vi "Auto_New.vi"() -> ()   [LabVIEW 2017]
uses:
  Control/Saurabh/prosucer_consumer_enum1.ctl
  <vilib>/Utility/error.llb/DialogType.ctl
  <vilib>/addons/database/Connection.llb/DB Tools Open Connec (String).vi
  Global/Global 1.vi
  Global/DATA LOG.vi
  <vilib>/addons/database/NI_Database_API.lvlib
panel:
  out "OP30 BARCODE STRING EMPRTY 2":bool
  out "SHIFT":string
  in  "BARCODE RECIPE":string(combo)
  out "PLC COM.":bool
  out "SHIFT_DATA":string[](array[string])
  out "OP30 BARCODE STRING EMPRTY":bool
  out "stop":bool
  out "error out 2":errorcluster
  out "Shift 4":i32
  out "Time Stamp Out":timestamp[](array[timestamp]) format="%<%X>T"
  out "Time Stamp Out 4":timestamp[](array[timestamp]) format="%<%X>T"
  out "Shift_change":bool
  out "appended array":string[][](array[string])
  out "SHIFT_DATA 2":string[](array[string])
  in  "error in (no error)":errorcluster
  in  "Tab Control":enum32{"Screen 1", "Screen 2"}(tab)
  out "OP 50":bool
  out "OP 40":bool
  out "OP 30":bool
  out "OP - 50":T1
  out "OP - 40":T2
  out "OP - 30":T3
  in  "stop 2":bool
  out "OP - 10":T4
  in  "SIMULATE INPUT":bool[](array[boolean])=[FALSE, FALSE, FALSE, FALSE]
  out "OP - 20":T5
  out "OP 10 & 20":bool
  out "OP - 110":cluster{"BARCODE":string}
  out "OP - 80":T6
  out "OP - 70":T7
  out "OP - 90":T8
  out "OP - 100":T9
  out "OP - 60":T10
  out "OP 60":bool
  out "OP 70 & 80":bool
  out "OP 90 -100 - 110":bool
  # "Op10 20\nOp30\nOp 40\nOp50\nOp60\nOp70-80\nOp 90-100-110"
  # "SENSOR MIN VLTG"
  # "Op10 20\nOp30\nOp 40\nOp50\nOp60\nOp70-80\nOp 90-100-110"
  # "OP - 50"
  # "OP - 40"
  # "OP - 30"
  # "OP - 10"
  # "OP - 20"
  # "OP - 110"
  # "OP - 80"
  # "OP - 70"
  # "OP - 90"
  # "OP - 100"
  # "OP - 60"
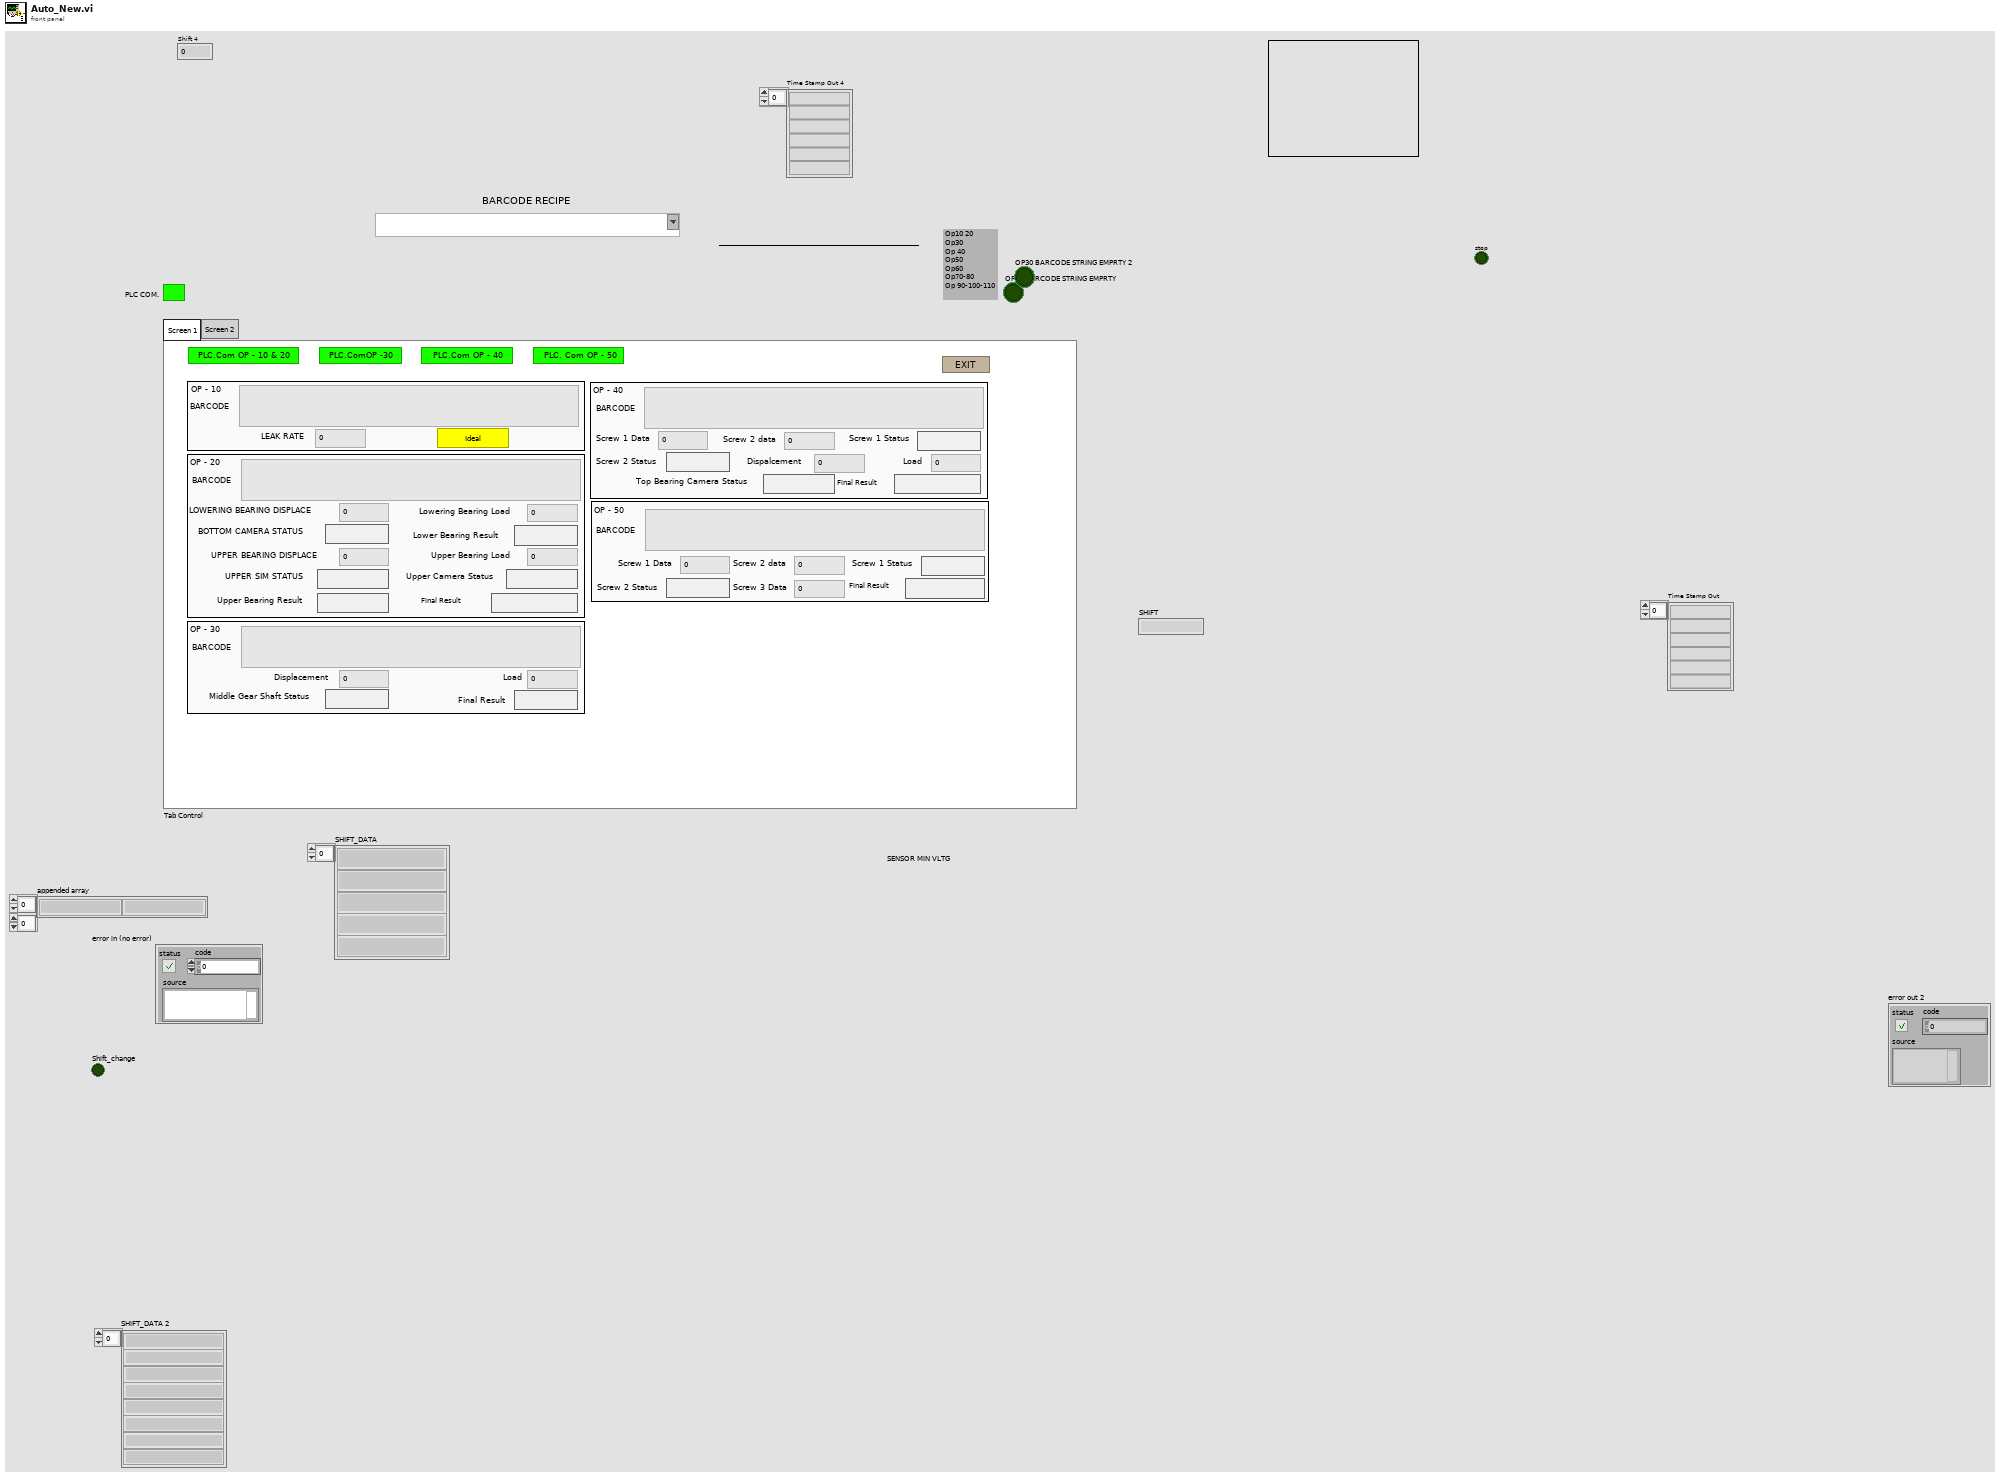
[diagram p1: front panel]
types:
  T1 = cluster{"BARCODE":string, "Screw 1 Data":dbl, "Screw 2 data":dbl, "Screw 1 Status":bool, "Screw 2 Status":bool, "Screw 3 Data":dbl, "Final Result":bool}
  T2 = cluster{"BARCODE":string, "Screw 1 Data":dbl, "Screw 2 data":dbl, "Screw 1 Status":bool, "Screw 2 Status":bool, "Dispalcement ":dbl, "Load ":dbl, "Top Bearing Camera Status":bool, "Final Result":bool}
  T3 = cluster{"BARCODE":string, "Displacement":dbl, "Load":dbl, "Middle Gear Shaft Status":bool, "Final Result":bool}
  T4 = cluster{"BARCODE":string, "LEAK RATE":dbl, "RESULT":bool}
  T5 = cluster{"BARCODE":string, "LOWERING BEARING DISPLACE":dbl, "Lowering Bearing Load":dbl, "BOTTOM CAMERA STATUS":bool, "Lower Bearing Result":bool, "UPPER BEARING DISPLACE":dbl, "Upper Bearing Load ":dbl, "UPPER SIM STATUS":bool, "Upper Camera Status":bool, "Upper Bearing Result":bool, "Final Result":bool}
  T6 = cluster{"BARCODE":string, "Load":dbl, "Final Result":bool, "Dispensing":bool}
  T7 = cluster{"BARCODE":string, "Sensor MIN Vltg":dbl, "Sensor MAX Vltg":dbl, "Final Result":bool}
  T8 = cluster{"BARCODE":string, "Seat LT Data":dbl, "Seat Status":bool, "Steam LT Data":dbl, "Final Result":bool}
  T9 = cluster{"BARCODE":string, "Sensor O/P Open V":dbl, "Start Of Close Sensor V":dbl, "Final Result":bool, "Sensor O/P Full Close V":dbl, "Response Time FWD (mSec)":dbl, "Response Time REV (mSec)":dbl, "Motor V Start Of Close A":dbl, "Motor V Full Close B R":dbl, "Motor V Start Back C":dbl, "Motor V Full Open D":dbl, "Motor RMS Current A":dbl}
  T10 = cluster{"BARCODE":string, "Screw 1 Data":dbl, "Screw 2 data":dbl, "Screw 1 Status":bool, "Screw 2 Status":bool, "Screw3 Data":dbl, "Final Result":bool, "Screw3 Status":bool, "Screw4 Data":dbl, "Screw5 Data":dbl, "Screw4 Status":bool, "Screw5 Status":bool, "Screw6 Data":dbl, "Screw6 Status":bool}
  T11 = cluster{"OP - 10":cluster{"BARCODE":string, "LEAK RATE":dbl, "RESULT":bool}, "OP - 20":cluster{"BARCODE":string, "LOWERING BEARING DISPLACE":dbl, "LOWERING BEARING LOAD":dbl, "BOTTOM CAMERA STATUS":bool, "LOWER BEARING RESULT":bool, "UPPER BEARING DISPLACE":dbl, "UPPER BEARING LOAD ":dbl, "UPPER SIM STATUS":bool, "UPPER CAMERA STATUS":bool, "UPPER BEARING RESULT":bool, "FINAL RESULT":bool}, "OP - 30":cluster{"BARCODE":string, "Displacement":dbl, "Load":dbl, "Middle Gear Shaft Status":bool, "Final Result":bool}, "OP - 40":cluster{"BARCODE":string, "Screw 1 Data":dbl, "Screw 2 data":dbl, "Screw 1 Status":bool, "Screw 2 Status":bool, "Dispalcement ":dbl, "Load ":dbl, "Top Bearing Camera Status":bool, "Final Result":bool}, "OP - 50":cluster{"BARCODE":string, "Screw 1 Data":dbl, "Screw 2 data":dbl, "Screw 1 Status":bool, "Screw 2 Status":bool, "Screw 3 Data":dbl, "Final Result":bool}, "OP - 60":cluster{"BARCODE":string, "Screw 1 Data":dbl, "Screw 2 data":dbl, "Screw 1 Status":bool, "Screw 2 Status":bool, "Screw3 Data":dbl, "Final Result":bool, "Screw3 Status":bool, "Screw4 Data":dbl, "Screw5 Data":dbl, "Screw4 Status":bool, "Screw5 Status":bool, "Screw6 Data":dbl, "Screw6 Status":bool}, "OP - 70":cluster{"BARCODE":string, "Sensor MIN Vltg":dbl, "Sensor MAX Vltg":dbl, "Final Result":bool}, "OP - 80":cluster{"BARCODE":string, "Load":dbl, "Final Result":bool, "Dispensing":bool}, "OP - 90":cluster{"BARCODE":string, "Seat LT Data":dbl, "Seat Status":bool, "Steam LT Data":dbl, "Final Result":bool}, "OP - 100":cluster{"BARCODE":string, "Sensor O/P Open V":dbl, "Start Of Close Sensor V":dbl, "Final Result":bool, "Sensor O/P Full Close V":dbl, "Response Time FWD (mSec)":dbl, "Response Time REV (mSec)":dbl, "Motor V Start Of Close A":dbl, "Motor V Full Close B R":dbl, "Motor V Start Back C":dbl, "Motor V Full Open D":dbl, "Motor RMS Current A":dbl}, "OP - 110":cluster{"BARCODE":string}}
  T12 = typedef "prosucer_consumer_enum1.ctl" = enum16{"SCAN1", "SCAN2", "SCAN3", "SCAN4", "SCAN5", "SCAN6", "SCAN7", "SCAN8", "SCAN9", "SCAN10", "SCAN11", "STOP", "DATALOG1", "DATALOG2", "DATALOG3", "DATALOG4", "DATALOG5", "DATALOG6", "DATALOG7", "DATALOG8", "DATALOG9", "DATALOG10", "DATALOG11", "-1", "CYCLE_START1", "CYCLE_START2", "CYCLE_START3", "CYCLE_START4", "BARCODE RECIPE", "EMERGENCY STOP"}
  T13 = typedef "NI_Database_API.lvlib/Conn ObjectReference.ctl" = refnum<k1>
  T14 = typedef "DialogType.ctl" = u16
  T15 = cluster{"trimmed string":string, "SHIFT":string, "date/time string":string, string, "Input 2":string}
  T16 = cluster{"SHIFT":string, "date/time string":string, "Input 2":string, string}
  T17 = cluster{"date/time string":string, "Input 2":string, "Input 2":string, "Input 2":string, "Input 2":string, "Input 2":string, "Input 2":string, "Input 2":string, "Input 2":string, "Input 2":string, "Input 2":string}
  T18 = cluster{"date/time string":string, "SHIFT":string, "Input 2":string, "Input 2":string, "Input 2":string, "Input 2":string, "Input 2":string, "Input 2":string, "Input 2":string, "Input 2":string, "Input 2":string, "Input 2":string}
  T19 = cluster{"date/time string":string, "Input 2":string, "Input 2":string, "Input 2":string, "Input 2":string}
  T20 = cluster{"date/time string":string, "SHIFT":string, "Input 2":string, "Input 2":string, "Input 2":string, "Input 2":string}
  T21 = cluster{"date/time string":string, "Input 2":string, "Input 2":string, "Input 2":string, "Input 2":string, "Input 2":string, "Input 2":string, "Input 2":string, "Input 2":string}
  T22 = cluster{"date/time string":string, "SHIFT":string, "Input 2":string, "Input 2":string, "Input 2":string, "Input 2":string, "Input 2":string, "Input 2":string, "Input 2":string, "Input 2":string}
  T23 = cluster{"date/time string":string, "Input 2":string, "Input 2":string, "Input 2":string, "Input 2":string, "Input 2":string, "Input 2":string}
  T24 = cluster{"date/time string":string, "SHIFT":string, "Input 2":string, "Input 2":string, "Input 2":string, "Input 2":string, "Input 2":string, "Input 2":string}
  T25 = cluster{"date/time string":string, "Input 2":string, "Input 2":string, "Input 2":string, "Input 2":string, "Input 2":string, "Input 2":string, "Input 2":string, "Input 2":string, "Input 2":string, "Input 2":string, "Input 2":string, "Input 2":string}
  T26 = cluster{"date/time string":string, "SHIFT":string, "Input 2":string, "Input 2":string, "Input 2":string, "Input 2":string, "Input 2":string, "Input 2":string, "Input 2":string, "Input 2":string, "Input 2":string, "Input 2":string, "Input 2":string, "Input 2":string}
  T27 = cluster{"date/time string":string, "Input 2":string, "Input 2":string, "Input 2":string}
  T28 = cluster{"date/time string":string, "SHIFT":string, "Input 2":string, "Input 2":string, "Input 2":string}
  T29 = cluster{"date/time string":string, "Input 2":string, "Input 2":string, "Input 2":string, "time string":string, "time string":string, "Input 2":string, "Input 2":string, "Input 2":string, "Input 2":string, "Input 2":string, "Input 2":string, "Input 2":string}
  T30 = cluster{"date/time string":string, "SHIFT":string, "Input 2":string, "Input 2":string, "Input 2":string, "time string":string, "time string":string, "Input 2":string, "Input 2":string, "Input 2":string, "Input 2":string, "Input 2":string, "Input 2":string, "Input 2":string}
  T31 = cluster{"BARCODE":string, "LOWERING BEARING DISPLACE":dbl, "LOWERING BEARING LOAD":dbl, "BOTTOM CAMERA STATUS":bool, "LOWER BEARING RESULT":bool, "UPPER BEARING DISPLACE":dbl, "UPPER BEARING LOAD ":dbl, "UPPER SIM STATUS":bool, "UPPER CAMERA STATUS":bool, "UPPER BEARING RESULT":bool, "FINAL RESULT":bool}
  T32 = enum32{"invalid app kind", "Development System", "Run Time System", "Student Edition", "Embedded LabVIEW", "Evaluation", "Custom"}
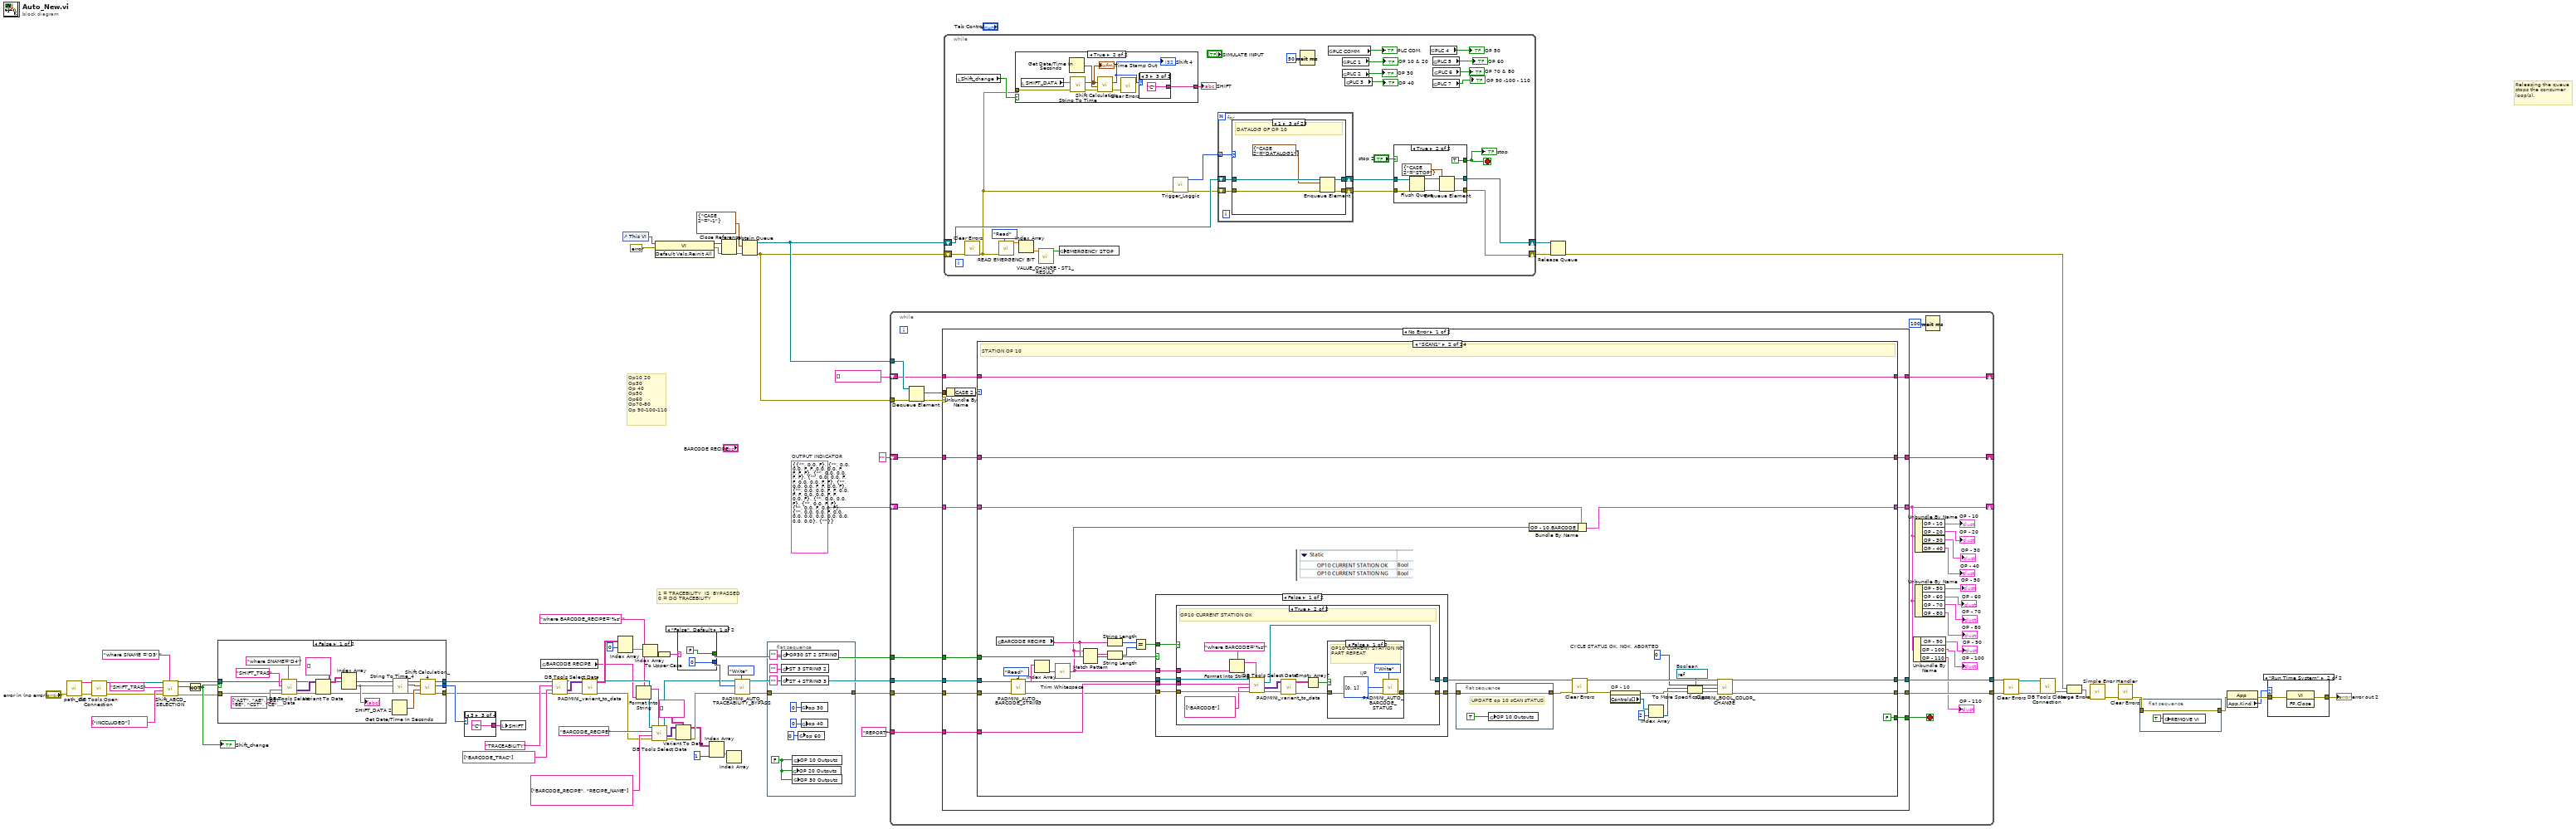
[diagram p0: block diagram]
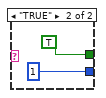
[diagram p2: hidden frame]
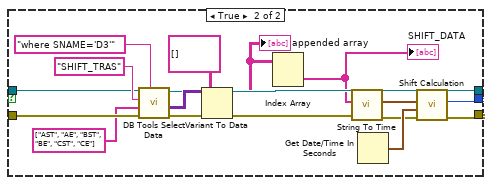
[diagram p3: hidden frame]
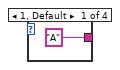
[diagram p4: hidden frame]
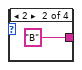
[diagram p5: hidden frame]
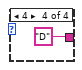
[diagram p6: hidden frame]
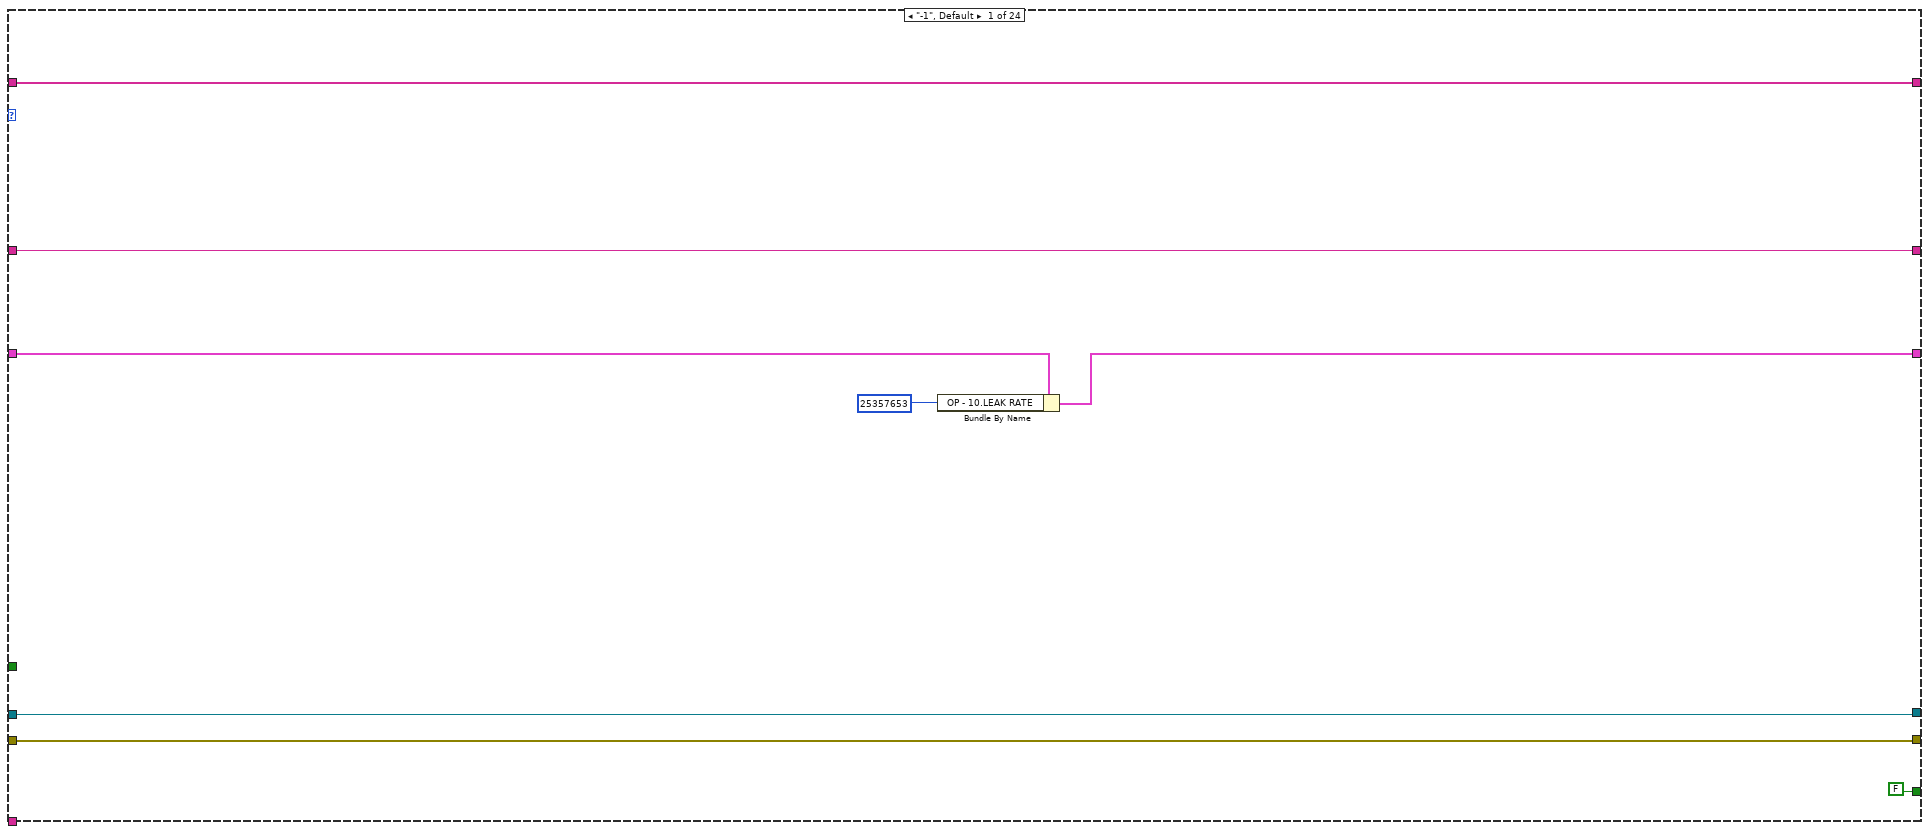
[diagram p7: hidden frame]
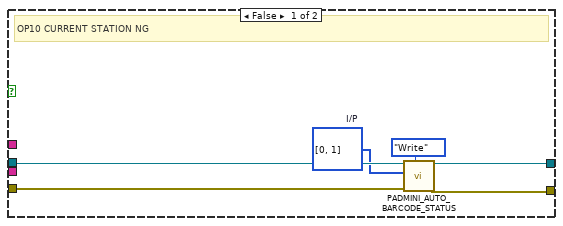
[diagram p8: hidden frame]
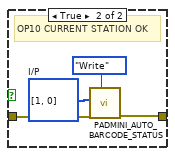
[diagram p9: hidden frame]
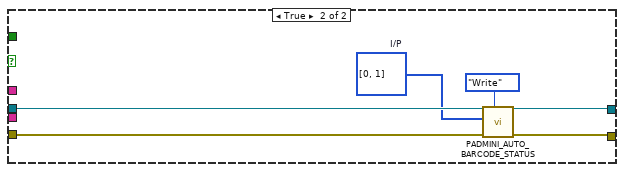
[diagram p10: hidden frame]
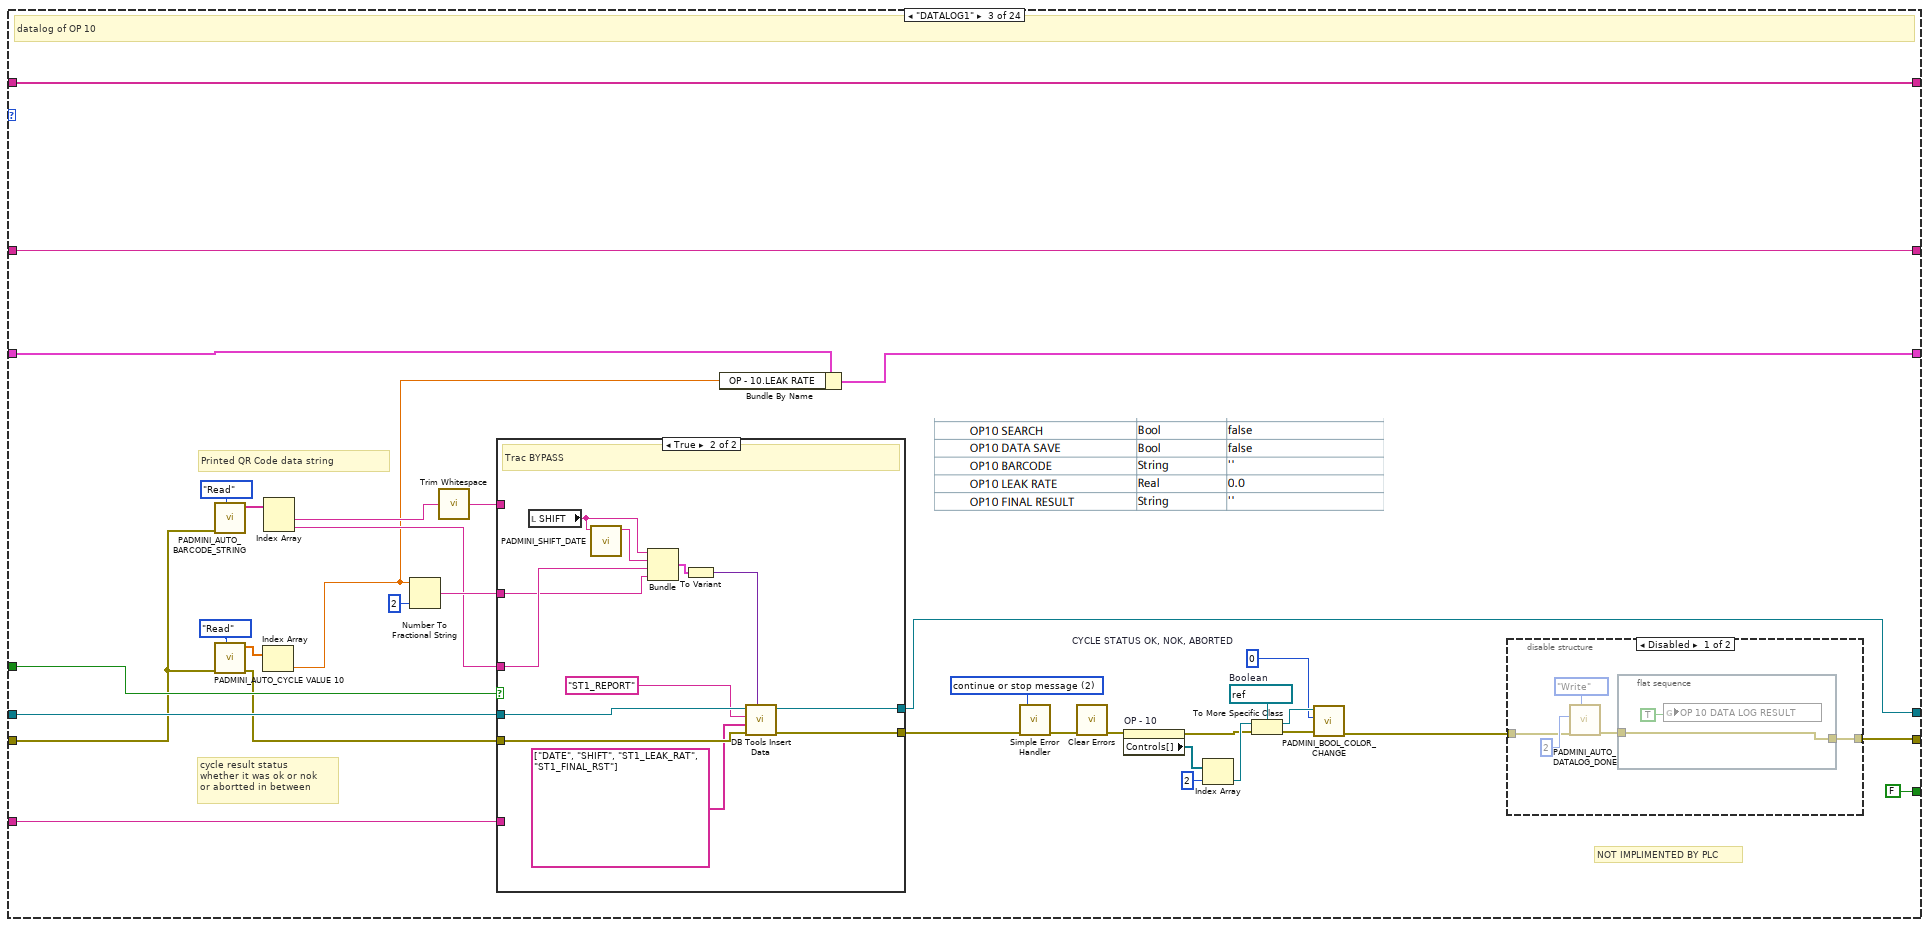
[diagram p11: hidden frame]
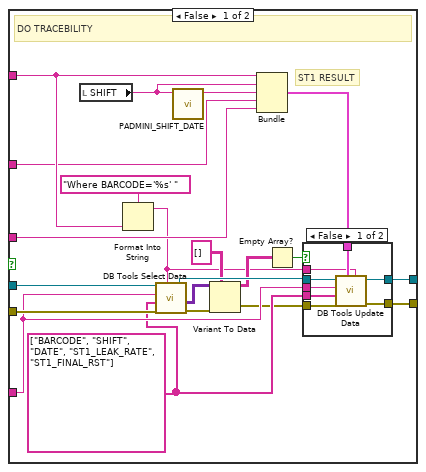
[diagram p13: hidden frame]
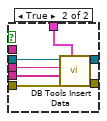
[diagram p14: hidden frame]
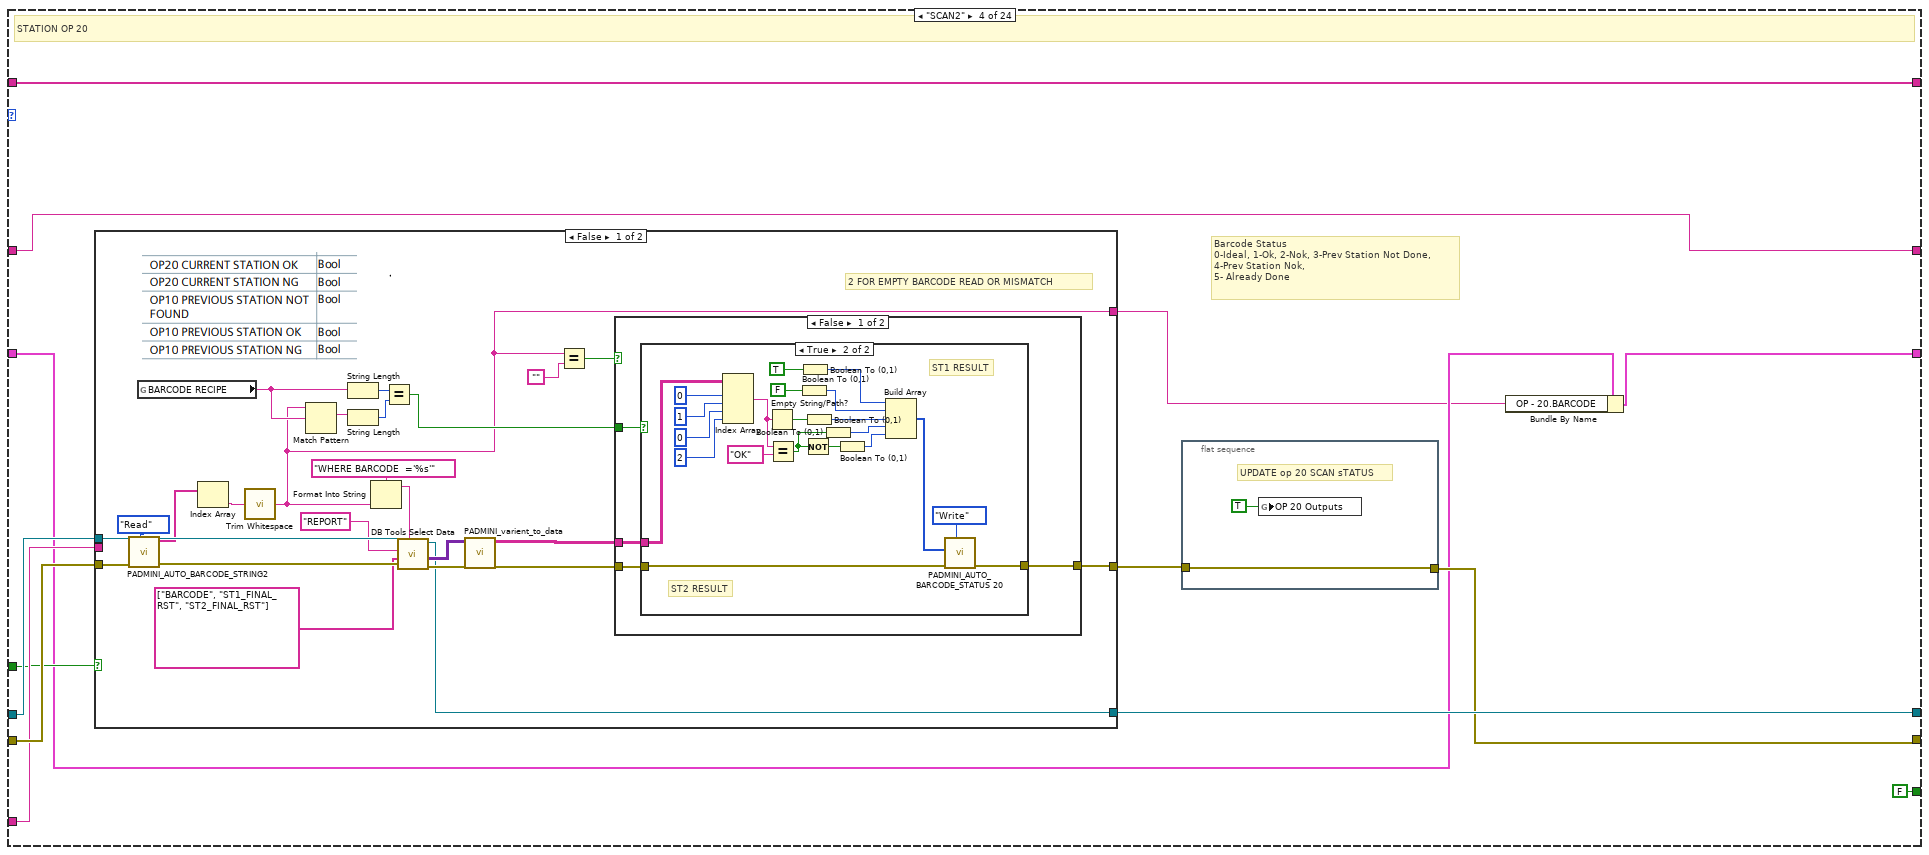
[diagram p15: hidden frame]
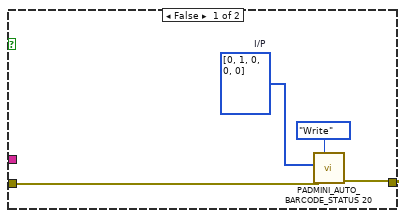
[diagram p16: hidden frame]
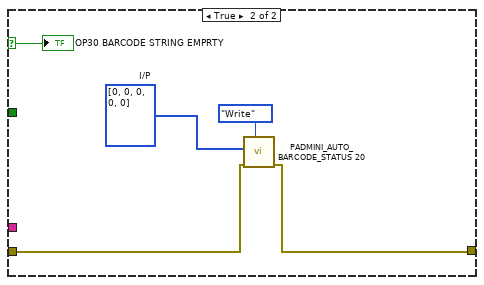
[diagram p17: hidden frame]
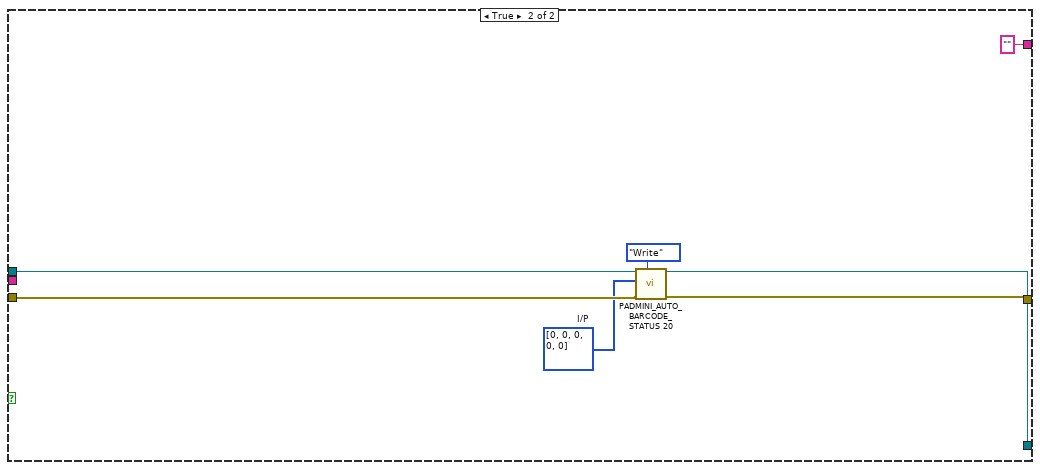
[diagram p18: hidden frame]
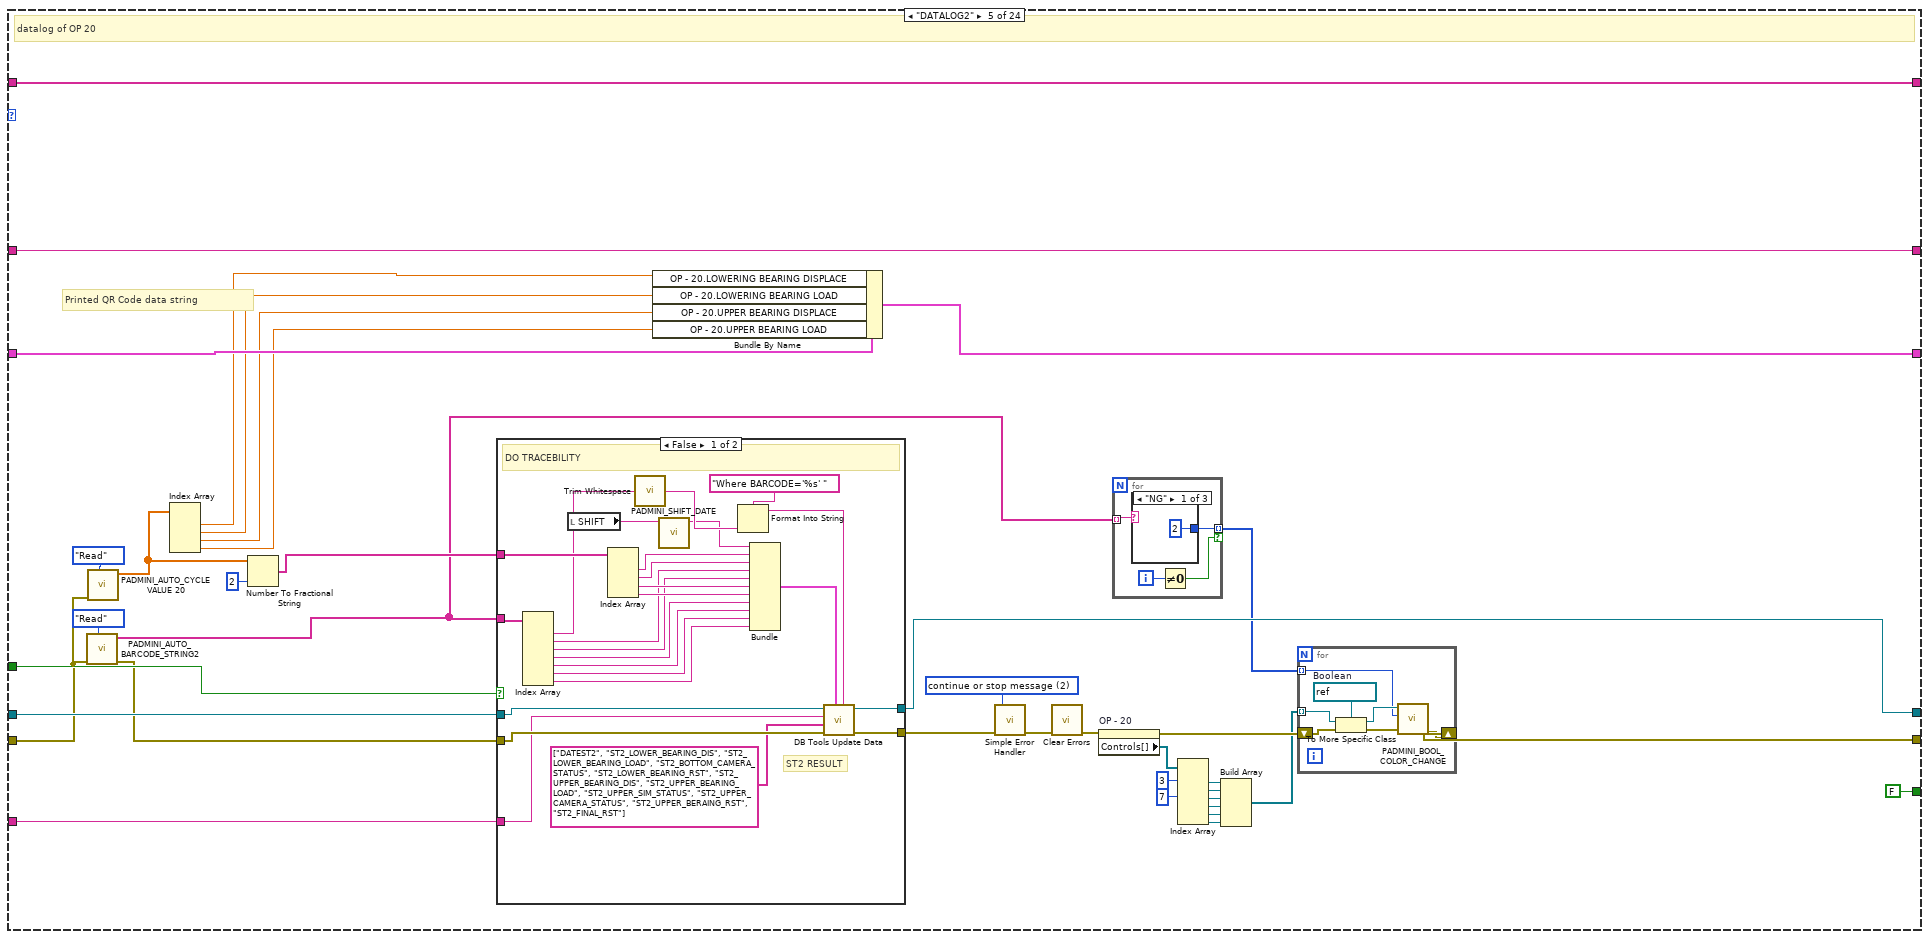
[diagram p19: hidden frame]
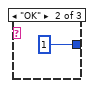
[diagram p20: hidden frame]
diagram:
  w2 = T11 {"OP - 10"={"BARCODE"="", "LEAK RATE"=0.0, "RESULT"=FALSE}, "OP - 20"={"BARCODE"="", "LOWERING BEARING DISPLACE"=0.0, "LOWERING BEARING LOAD"=0.0, "BOTTOM CAMERA STATUS"=FALSE, "LOWER BEARING RESULT"=FALSE, "UPPER BEARING DISPLACE"=0.0, "UPPER BEARING LOAD "=0.0, "UPPER SIM STATUS"=FALSE, "UPPER CAMERA STATUS"=FALSE, "UPPER BEARING RESULT"=FALSE, "FINAL RESULT"=FALSE}, "OP - 30"={"BARCODE"="", "Displacement"=0.0, "Load"=0.0, "Middle Gear Shaft Status"=FALSE, "Final Result"=FALSE}, "OP - 40"={"BARCODE"="", "Screw 1 Data"=0.0, "Screw 2 data"=0.0, "Screw 1 Status"=FALSE, "Screw 2 Status"=FALSE, "Dispalcement "=0.0, "Load "=0.0, "Top Bearing Camera Status"=FALSE, "Final Result"=FALSE}, "OP - 50"={"BARCODE"="", "Screw 1 Data"=0.0, "Screw 2 data"=0.0, "Screw 1 Status"=FALSE, "Screw 2 Status"=FALSE, "Screw 3 Data"=0.0, "Final Result"=FALSE}, "OP - 60"={"BARCODE"="", "Screw 1 Data"=0.0, "Screw 2 data"=0.0, "Screw 1 Status"=FALSE, "Screw 2 Status"=FALSE, "Screw3 Data"=0.0, "Final Result"=FALSE, "Screw3 Status"=FALSE, "Screw4 Data"=0.0, "Screw5 Data"=0.0, "Screw4 Status"=FALSE, "Screw5 Status"=FALSE, "Screw6 Data"=0.0, "Screw6 Status"=FALSE}, "OP - 70"={"BARCODE"="", "Sensor MIN Vltg"=0.0, "Sensor MAX Vltg"=0.0, "Final Result"=FALSE}, "OP - 80"={"BARCODE"="", "Load"=0.0, "Final Result"=FALSE, "Dispensing"=FALSE}, "OP - 90"={"BARCODE"="", "Seat LT Data"=0.0, "Seat Status"=FALSE, "Steam LT Data"=0.0, "Final Result"=FALSE}, "OP - 100"={"BARCODE"="", "Sensor O/P Open V"=0.0, "Start Of Close Sensor V"=0.0, "Final Result"=FALSE, "Sensor O/P Full Close V"=0.0, "Response Time FWD (mSec)"=0.0, "Response Time REV (mSec)"=0.0, "Motor V Start Of Close A"=0.0, "Motor V Full Close B R"=0.0, "Motor V Start Back C"=0.0, "Motor V Full Open D"=0.0, "Motor RMS Current A"=0.0}, "OP - 110"={"BARCODE"=""}}  # OUTPUT INDICATOR
  # "Op10 20\nOp30\nOp 40\nOp50\nOp60\nOp70-80\nOp 90-100-110"
  # "1 = TRACEBILITY  IS  BYPASSED\n0 = DO TRACEBILITY"
  # "Releasing the queue stops the consumer loop(s)."
  n1 = call "path_db.vi"("error in"="error in (no error)") -> ("error out"=w47:errorcluster, "resulting string"=w68:string)  [unwired: 9 in]
  n2 = call-poly <vilib>:"DB Tools Open Connection.vi"("error in (no error)"=w47, "connection information"=w68) -> ("error out"=w46:errorcluster, "connection reference"=w39:T13)  [unwired: 6 in]
  n3 = call "Shift_ABCD_SELECTION.vi"("Where"="where SNAME ='D3' ", "error in (no error)"=w46, "Array"=string[] ["INCCLUDED"], "table"="SHIFT_TRAS", "Refnum in"=w39) -> ("error out"=w1:errorcluster, "Boolean"=w59:bool, "Refnum out"=w60:T13)  [unwired: 4 in]
  n4 = Not(x=w59) -> (.not. x?=w58:bool)
  "Shift_change" <- w58
  n5 = case shown="False" w58 {
    tunnel: [w73 w97] -> w64
    tunnel: w60 -> [w76 w95]
    tunnel: w1 -> [w75 w94]
    tunnel: [w74 w93] -> w28
    tunnel: [w72 w87] -> w27
    frame False {
      n6 = call <vilib>:"DB Tools Select Data.vi"("condition"="where SNAME='D4'", "error in (no error)"=w75, "columns"=string[] ["AST", "AE", "BST", "BE", "CST", "CE", "DST", "DE"], "table"="SHIFT_TRAS", "connection reference"=w76) -> ("error out"=w82:errorcluster, "data"=w86:variant[][], "connection reference out"=w74:T13)  [unwired: 1 in]
      n7 = Variant To Data(error in=w82, type=string[][] [], Variant=w86) -> (data=w79:string[][], error out=w72:errorcluster)
      n8 = Index Array(array=w79) -> (element=w78:string[])  [unwired: 2 in]
      "SHIFT_DATA 2" <- w78
      n9 = Get Date/Time In Seconds() -> (seconds since 1Jan1904=w81:timestamp)
      n10 = call "String To Time_4.vi"("String Array In"=w78) -> ("Time Stamp Out"=w77:timestamp[])  [unwired: 9 in, 1 out]
      n11 = call "Shift Calculation_4.vi"("Current Time"=w81, "Time Stamp Out"=w77) -> ("Shift"=w73:i32)  [unwired: 8 in, 1 out]
    }
    frame True {
      n12 = call <vilib>:"DB Tools Select Data.vi"("condition"="where SNAME='D3'", "error in (no error)"=w94, "columns"=string[] ["AST", "AE", "BST", "BE", "CST", "CE"], "table"="SHIFT_TRAS", "connection reference"=w95) -> ("error out"=w99:errorcluster, "data"=w103:variant[][], "connection reference out"=w93:T13)  [unwired: 1 in]
      n13 = Variant To Data(error in=w99, type=string[][] [], Variant=w103) -> (data=w91:string[][], error out=w89:errorcluster)
      "appended array" <- w91
      n14 = Index Array(array=w91) -> (element=w90:string[])  [unwired: 2 in]
      "SHIFT_DATA" <- w90
      n15 = call "String To Time.vi"("error in (no error)"=w89, "String Array In"=w90) -> ("error out"=w88:errorcluster, "Time Stamp Out"=w96:timestamp[])  [unwired: 8 in]
      n16 = Get Date/Time In Seconds() -> (seconds since 1Jan1904=w98:timestamp)
      n17 = call "Shift Calculation.vi"("error in (no error)"=w88, "Current Time"=w98, "Time Stamp Out"=w96) -> ("error out"=w87:errorcluster, "Shift"=w97:i32)  [unwired: 7 in]
    }
  }
  n18 = case shown="3" w64 {
    tunnel: ["A" "B" "C" "D"] -> w57
    frame 1, Default {
    }
    frame 2 {
    }
    frame 3 {
    }
    frame 4 {
    }
  }
  n19 = local write "SHIFT"(w57) -> ()
  n20 = global read "Global 1.vi" "BARCODE RECIPE"() -> (w8:string)
  n21 = call <vilib>:"DB Tools Select Data.vi"("error in (no error)"=w27, "columns"=string[] ["BARCODE_TRAC"], "table"="TRACEABILITY", "connection reference"=w28) -> ("error out"=w37:errorcluster, "data"=w36:variant[][], "connection reference out"=w14:T13)  [unwired: 2 in]
  n22 = call "PADMINI_varient_to_data.vi"("error in (no error)"=w37, "data"=w36) -> ("error out"=w12:errorcluster, "Array"=w35:string[][])  [unwired: 8 in]
  n23 = Index Array(array=w35, index (row)=0 ("disabled index (col)")) -> (element=w34:string[])  [unwired: 1 in]
  n24 = control-ref of="This VI"() -> (w44:refnum<vi>)
  n25 = Format Into String(format string="where BARCODE_RECIPE='%s' ", w8) -> (resulting string=w6:string)  [unwired: 2 in, 1 out]
  n26 = Index Array(array=w34) -> (element=w30:string)  [unwired: 1 in]
  n27 = call <vilib>:"DB Tools Select Data.vi"("condition"=w6, "error in (no error)"=w12, "columns"=string[] ["BARCODE_RECIPE", "RECIPE_NAME"], "table"="BARCODE_RECIPE", "connection reference"=w14) -> ("error out"=w16:errorcluster, "data"=w15:variant[][], "connection reference out"=w13:T13)  [unwired: 1 in]
  n28 = invoke class="VI" method="Default Vals.Reinit All"(reference=w44, error in=errorcluster {"status"=FALSE, "code"=0, "source"=""} ("error in (no error)")) -> (reference out=w42:refnum<vi>, error out=w43:errorcluster)  [unwired: 1 in, 1 out]
  n29 = To Upper Case(1:w30) -> (0:w29:string)
  n30 = Variant To Data(error in=w16, type=string[][] [], Variant=w15) -> (data=w9:string[][], error out=w11:errorcluster)
  n31 = case shown="\"False\", Default" w29 {
    tunnel: [FALSE ("BARCODE TRACEABILITY") TRUE ("BARCODE TRACEABILITY")] -> w19
    tunnel: [0 1] -> w25
    frame "False", Default {
    }
    frame "TRUE" {
    }
  }
  n32 = Index Array(array=w9, index (col)=1 ("disabled index (col)")) -> (element=w4:string[])  [unwired: 1 in]
  n33 = Close Reference(reference=w42, error in (no error)=w43) -> (error out=w40:errorcluster)
  n34 = Index Array(array=w4) -> ()  [unwired: 1 in, 1 out]
  n35 = call "PADMINI_AUTO_TRACEABILITY_BYPASS.vi"("Enum"=enum16{"Read", "Write"}."Write", "error in (no error)"=w11, "I/P"=w25) -> ("error out"=w23:errorcluster)  [unwired: 7 in, 1 out]
  n36 = Obtain Queue(element data type=cluster{"CASE 2":T12} {"CASE 2"=enum."-1"}, error in (no error)=w40) -> (queue out=w69:refnum<queue>, error out=w20:errorcluster)  [unwired: 3 in, 1 out]
  n37 = flat-sequence {
    tunnel: w23 -> [w116]
    tunnel: [w116] -> w22
    frame #0 {
      w112 = FALSE
      n38 = global write "DATA LOG.vi" "OP30 ST 2 STRING"("" ("OP30 ST 2 STRING")) -> ()
      n39 = global write "DATA LOG.vi" "ST 3 STRING 2"("" ("ST 3 STRING 2")) -> ()
      n40 = global write "DATA LOG.vi" "ST 4 STRING 3"("" ("ST 4 STRING 3")) -> ()
      n41 = global write "DATA LOG.vi" "OP 20 Outputs"(w112) -> ()
      n42 = global write "DATA LOG.vi" "OP 10 Outputs"(w112) -> ()
      n43 = global write "DATA LOG.vi" "OP 30 Outputs"(w112) -> ()
      n44 = global write "DATA LOG.vi" "op 60"(0 ("op 30")) -> ()
      n45 = global write "DATA LOG.vi" "op 30"(0 ("op 30")) -> ()
      n46 = global write "DATA LOG.vi" "op 40"(0 ("op 30")) -> ()
    }
  }
  n47 = while {
    tunnel: w69 -> [w148]
    tunnel: w20 -> [w144]
    tunnel: w22 -> [w143]
    tunnel: w13 -> [w142]
    tunnel: [w141] -> w67
    tunnel: [w140] -> w66
    tunnel: w19 -> [w139]
    tunnel: "REPORT" -> [w138]
    shift-right: [w136] -> _
    shift-left: string[] [] -> [w137]
    shift-right: [w135] -> _
    shift-left: "" ("trimmed string") -> [w134]
    shift-right: [w123] -> _
    shift-left: w2 -> [w132]
    stop <- w145 stop-if-true
    n48 = Dequeue Element(queue=w148, error in (no error)=w144) -> (element=w146:cluster{"CASE 2":T12}, error out=w147:errorcluster)  [unwired: 1 in, 2 out]
    n49 = case shown="No Error" w147 {
      tunnel: w146 -> [w163 _]
      tunnel: [w159 TRUE] -> w145
      tunnel: w143 -> [w160 w1951]
      tunnel: w142 -> [w161 w1950]
      tunnel: [w157 w1951] -> w141
      tunnel: [w158 w1950] -> w140
      tunnel: w139 -> [w156 _]
      tunnel: w138 -> [w155 _]
      tunnel: w137 -> [w154 w1949]
      tunnel: [w153 w1949] -> w136
      tunnel: [w152 w1948] -> w135
      tunnel: w134 -> [w151 w1948]
      tunnel: w132 -> [w150 w1947]
      tunnel: [w149 w1947] -> w123
      frame No Error {
        n50 = Unbundle By Name(w163) -> ("CASE 2"=w162:T12)
        n51 = case shown="\"SCAN1\"" w162 {
          tunnel: w161 -> [w170 w202 w278 w348 w451 w526 w624 w687 w789 w860 w959 w1026 w1134 w1213 w1305 w1366 w1461 w1522 w1618 w1681 w1757 w1863 w1934 w1942]
          tunnel: w160 -> [w169 w198 w245 w347 w432 w525 w605 w686 w770 w859 w940 w1025 w1115 w1212 w1286 w1365 w1442 w1521 w1599 w1680 w1756 w1828 w1933 w1944]
          tunnel: [FALSE FALSE FALSE FALSE FALSE FALSE FALSE FALSE FALSE FALSE FALSE FALSE FALSE FALSE FALSE FALSE FALSE FALSE FALSE FALSE FALSE FALSE FALSE TRUE] -> w159
          tunnel: [w170 w200 w275 w345 w448 w523 w621 w684 w786 w857 w956 w1023 w1131 w1210 w1302 w1363 w1458 w1519 w1615 w1678 w1754 w1860 w1934 w1941] -> w158
          tunnel: [w169 w177 w274 w342 w438 w520 w611 w681 w776 w854 w946 w1020 w1121 w1207 w1292 w1360 w1448 w1516 w1605 w1675 w1751 w1850 w1933 w1943] -> w157
          tunnel: w156 -> [_ w195 w277 w344 w450 w522 w623 w683 w788 w856 w958 w1022 w1133 w1209 w1304 w1362 w1460 w1518 w1617 w1677 w1753 w1862 _ _]
          tunnel: w155 -> [_ w201 w276 w346 w449 w524 w622 w685 w787 w858 w957 w1024 w1132 w1211 w1303 w1364 w1459 w1520 w1616 w1679 w1755 w1861 _ _]
          tunnel: w154 -> [w168 w199 w271 w339 w447 w518 w620 w679 w785 w852 w955 w1018 w1130 w1205 w1301 w1358 w1457 w1514 w1614 w1673 w1749 w1859 w1931 w1945]
          tunnel: [w168 w199 w271 w339 w447 w518 w620 w679 w785 w852 w955 w1018 w1130 w1205 w1301 w1358 w1457 w1514 w1614 w1673 w1749 w1859 w1931 w1945] -> w153
          tunnel: [w167 w194 w267 w340 w443 w517 w616 w678 w781 w851 w951 w1017 w1126 w1204 w1297 w1357 w1453 w1513 w1610 w1672 w1748 w1855 w1930 w1936] -> w152
          tunnel: w151 -> [w167 w194 w267 w340 w443 w517 w616 w678 w781 w851 w951 w1017 w1126 w1204 w1297 w1357 w1453 w1513 w1610 w1672 w1748 w1855 w1930 w1936]
          tunnel: w150 -> [w166 w188 w256 w338 w437 w516 w610 w677 w775 w850 w945 w1016 w1120 w1203 w1291 w1356 w1447 w1512 w1604 w1671 w1747 w1849 w1929 w1935]
          tunnel: [w165 w187 w255 w337 w436 w515 w609 w676 w774 w849 w944 w1015 w1119 w1202 w1290 w1355 w1446 w1511 w1603 w1670 w1747 w1848 w1929 w1935] -> w149
          frame "-1", Default {
            n52 = Bundle By Name(cluster=w166, "OP - 10.LEAK RATE"=25357653) -> (w165:T11)
          }
          frame "SCAN1" {
            w180 = u16 0  # CYCLE STATUS OK, NOK, ABORTED
            w179 = refnum<vi> refnum  # Boolean
            # "STATION OP 10"
            n53 = global read "Global 1.vi" "BARCODE RECIPE"() -> (w189:string)
            n54 = call "PADMINI_AUTO_BARCODE_STRING.vi"("Enum"=enum16{"Read", "Write"}."Read", "error in (no error)"=w198) -> ("error out"=w197:errorcluster, "Input 2"=w174:string[])  [unwired: 8 in]
            n55 = Index Array(array=w174) -> (element=w173:string)  [unwired: 1 in]
            n56 = call <vilib>:"Trim Whitespace.vi"("string"=w173) -> ("trimmed string"=w172:string)  [unwired: 1 in]
            n57 = Match Pattern(string=w172, regular expression=w189) -> (match substring=w192:string)  [unwired: 1 in, 3 out]
            n58 = String Length(string=w189) -> (length=w191:i32)
            n59 = String Length(string=w192) -> (length=w190:i32)
            n60 = Equal?(x=w191, y=w190) -> (x = y?=w196:bool)
            n61 = case shown="False" w195 {
              tunnel: w202 -> [w212 w244]
              tunnel: w197 -> [w211 w242]
              tunnel: w201 -> [w210 _]
              tunnel: [w209 w241] -> w176
              tunnel: [w208 w244] -> w200
              tunnel: w196 -> [w207 _]
              tunnel: w172 -> [w206 _]
              frame False {
                n62 = case shown="True" w207 {
                  tunnel: w212 -> [w214 w231]
                  tunnel: w211 -> [w216 w230]
                  tunnel: w210 -> [_ w229]
                  tunnel: [w215 w220] -> w209
                  tunnel: [w214 w219] -> w208
                  tunnel: w206 -> [_ w218]
                  frame False {
                    w213 = i32[] [0, 1]  # I/P
                    # "OP10 CURRENT STATION NG"
                    n63 = call "PADMINI_AUTO_BARCODE_STATUS.vi"("Enum"=enum16{"Read", "Write"}."Write", "error in (no error)"=w216, "I/P"=w213) -> ("error out"=w215:errorcluster)  [unwired: 7 in, 1 out]
                  }
                  frame True {
                    # "OP10 CURRENT STATION OK"
                    n64 = Format Into String(format string="where BARCODE='%s'", w218) -> (resulting string=w226:string)  [unwired: 2 in, 1 out]
                    n65 = call <vilib>:"DB Tools Select Data.vi"("condition"=w226, "error in (no error)"=w230, "columns"=string[] ["BARCODE"], "table"=w229, "connection reference"=w231) -> ("error out"=w225:errorcluster, "data"=w224:variant[][], "connection reference out"=w219:T13)  [unwired: 1 in]
                    n66 = call "PADMINI_varient_to_data.vi"("error in (no error)"=w225, "data"=w224) -> ("error out"=w221:errorcluster, "Array"=w223:string[][])  [unwired: 8 in]
                    n67 = Empty Array?(array=w223) -> (empty?=w222:bool)
                    n68 = case shown="False" w222 {
                      tunnel: w221 -> [w235 w239]
                      tunnel: [w234 w237] -> w220
                      frame False {
                        w232 = i32[] [0, 1]  # I/P
                        # "OP10 CURRENT STATION NG\nPART REPEAT"
                        n69 = call "PADMINI_AUTO_BARCODE_STATUS.vi"("Enum"=enum16{"Read", "Write"}."Write", "error in (no error)"=w235, "I/P"=w232) -> ("error out"=w234:errorcluster)  [unwired: 7 in, 1 out]
                      }
                      frame True {
                        w236 = i32[] [1, 0]  # I/P
                        # "OP10 CURRENT STATION OK"
                        n70 = call "PADMINI_AUTO_BARCODE_STATUS.vi"("Enum"=enum16{"Read", "Write"}."Write", "error in (no error)"=w239, "I/P"=w236) -> ("error out"=w237:errorcluster)  [unwired: 7 in, 1 out]
                      }
                    }
                  }
                }
              }
              frame True {
                w240 = i32[] [0, 1]  # I/P
                n71 = call "PADMINI_AUTO_BARCODE_STATUS.vi"("Enum"=enum16{"Read", "Write"}."Write", "error in (no error)"=w242, "I/P"=w240) -> ("error out"=w241:errorcluster)  [unwired: 7 in, 1 out]
              }
            }
            n72 = flat-sequence {
              tunnel: [w205] -> w175
              tunnel: w176 -> [w205]
              frame #0 {
                # "UPDATE op 10 sCAN sTATUS"
                n73 = global write "DATA LOG.vi" "OP 10 Outputs"(TRUE) -> ()
              }
            }
            n74 = Bundle By Name(cluster=w188, "OP - 10.BARCODE"=w172) -> (w187:T11)
            n75 = call <vilib>:"Clear Errors.vi"("error in (no error)"=w175) -> ("error out"=w181:errorcluster)  [unwired: 5 in, 1 out]
            n76 = property on="OP - 10" class="Clust"(error in=w181) -> (error out=w185:errorcluster, "Controls[]"=w183:refnum<vi>[])  [unwired: 1 in, 1 out]
            n77 = Index Array(array=w183, index=2) -> (element=w184:refnum<vi>)
            n78 = To More Specific Class(target class=w179, reference=w184, error in=w185) -> (specific class reference=w182:refnum<vi>, error out=w186:errorcluster)
            n79 = call "PADMINI_BOOL_COLOR_CHANGE.vi"("error in (no error)"=w186, "Numeric"=w180, "Boolean in"=w182) -> ("error out"=w177:errorcluster)  [unwired: 8 in]
          }
          frame "DATALOG1" {
            w257 = u16 0  # CYCLE STATUS OK, NOK, ABORTED
            w261 = refnum<vi> refnum  # Boolean
            w269 = T14 2 items=["no dialog", "OK message", "continue or stop message", "OK message + warnings", "continue/stop + warnings"] ("type of dialog (OK msg:1)")
            # "NOT IMPLIMENTED BY PLC"
            # "cycle result status\nwhether it was ok or nok\nor abortted in between"
            # "Printed QR Code data string"
            # "datalog of OP 10"
            n80 = call "PADMINI_AUTO_BARCODE_STRING.vi"("Enum"=enum16{"Read", "Write"}."Read", "error in (no error)"=w245) -> ("Input 2"=w252:string[])  [unwired: 8 in, 1 out]
            n81 = call "PADMINI_AUTO_CYCLE VALUE 10.vi"("Enum"=enum16{"Read", "Write"}."Read", "error in (no error)"=w245) -> ("error out"=w248:errorcluster, "Input 2"=w247:dbl[])  [unwired: 8 in]
            n82 = Index Array(array=w247) -> (element=w246:dbl)  [unwired: 1 in]
            n83 = Index Array(array=w252) -> (element #1=w251:string, element #2=w250:string)  [unwired: 2 in]
            n84 = Number To Fractional String(number=w246, precision (6)=i16 2) -> (F-format string=w253:string)  [unwired: 2 in]
            n85 = call <vilib>:"Trim Whitespace.vi"("string"=w251) -> ("trimmed string"=w272:string)  [unwired: 1 in]
            n86 = case shown="True" w277 {
              tunnel: w278 -> [w300 w335]
              tunnel: w248 -> [w302 w334]
              tunnel: [w308 w333] -> w275
              tunnel: [w307 w332] -> w270
              tunnel: w276 -> [w297 _]
              tunnel: w272 -> [w294 _]
              tunnel: w250 -> [w304 w325]
              tunnel: w253 -> [w288 w324]
              frame False {
                w296 = string[] ["BARCODE", "SHIFT", "DATE", "ST1_LEAK_RATE", "ST1_FINAL_RST"]
                # "ST1 RESULT"
                # "DO TRACEBILITY"
                n87 = local read "SHIFT"() -> (w306:string)
                n88 = Format Into String(format string="Where BARCODE='%s' ", w294) -> (resulting string=w289:string)  [unwired: 2 in, 1 out]
                n89 = call <vilib>:"DB Tools Select Data.vi"("condition"=w289, "error in (no error)"=w302, "columns"=w296, "table"=w297, "connection reference"=w300) -> ("error out"=w298:errorcluster, "data"=w301:variant[][], "connection reference out"=w299:T13)  [unwired: 1 in]
                n90 = call "PADMINI_SHIFT_DATE.vi"("SHIFT"=w306) -> ("date/time string"=w305:string)  [unwired: 10 in]
                n91 = Variant To Data(error in=w298, type=string[][] [], Variant=w301) -> (data=w292:string[][], error out=w290:errorcluster)
                n92 = Bundle("trimmed string"=w294, "SHIFT"=w306, "date/time string"=w305, w288, "Input 2"=w304) -> (w303:T15)  [unwired: 1 in]
                n93 = Empty Array?(array=w292) -> (empty?=w291:bool)
                n94 = case shown="False" w291 {
                  tunnel: w299 -> [w313 w323]
                  tunnel: w290 -> [w312 w322]
                  tunnel: [w316 w321] -> w308
                  tunnel: [w315 w320] -> w307
                  tunnel: w296 -> [w310 w319]
                  tunnel: w297 -> [w311 w318]
                  tunnel: w303 -> [w314 w317]
                  tunnel: w289 -> [w309 _]
                  frame False {
                    n95 = call <vilib>:"DB Tools Update Data.vi"("condition"=w309, "data"=w314, "error in (no error)"=w312, "columns"=w310, "table"=w311, "connection reference"=w313) -> ("error out"=w315:errorcluster, "connection reference out"=w316:T13)  [unwired: 4 in]
                  }
                  frame True {
                    n96 = call <vilib>:"DB Tools Insert Data.vi"("data"=w317, "error in (no error)"=w322, "columns"=w319, "table"=w318, "connection reference"=w323) -> ("error out"=w320:errorcluster, "connection reference out"=w321:T13)  [unwired: 5 in]
                  }
                }
              }
              frame True {
                # "Trac BYPASS"
                n97 = local read "SHIFT"() -> (w330:string)
                n98 = call "PADMINI_SHIFT_DATE.vi"("SHIFT"=w330) -> ("date/time string"=w329:string)  [unwired: 10 in]
                n99 = Bundle("SHIFT"=w330, "date/time string"=w329, "Input 2"=w325, w324) -> (w328:T16)  [unwired: 1 in]
                n100 = To Variant(anything=w328) -> (Variant=w327:variant)
                n101 = call <vilib>:"DB Tools Insert Data.vi"("data"=w327, "error in (no error)"=w334, "columns"=string[] ["DATE", "SHIFT", "ST1_LEAK_RAT", "ST1_FINAL_RST"], "table"="ST1_REPORT", "connection reference"=w335) -> ("error out"=w332:errorcluster, "connection reference out"=w333:T13)  [unwired: 5 in]
              }
            }
            n102 = Bundle By Name(cluster=w256, "OP - 10.LEAK RATE"=w246) -> (w255:T11)
            n103 = call <vilib>:"Simple Error Handler.vi"("type of dialog (OK msg:1)"=w269, "error in (no error)"=w270) -> ("error out"=w268:errorcluster)  [unwired: 3 in, 4 out]
            n104 = call <vilib>:"Clear Errors.vi"("error in (no error)"=w268) -> ("error out"=w266:errorcluster)  [unwired: 5 in, 1 out]
            n105 = property on="OP - 10" class="Clust"(error in=w266) -> (error out=w260:errorcluster, "Controls[]"=w264:refnum<vi>[])  [unwired: 1 in, 1 out]
            n106 = Index Array(array=w264, index=2) -> (element=w262:refnum<vi>)
            n107 = To More Specific Class(target class=w261, reference=w262, error in=w260) -> (specific class reference=w265:refnum<vi>, error out=w259:errorcluster)
            n108 = call "PADMINI_BOOL_COLOR_CHANGE.vi"("error in (no error)"=w259, "Numeric"=w257, "Boolean in"=w265) -> ("error out"=w258:errorcluster)  [unwired: 8 in]
            n109 = disable-structure shown="Disabled" {
              disable-tunnel: [w281 w287] -> w274
              disable-tunnel: w258 -> [w280 w287]
              frame Disabled {
                n110 = call "PADMINI_AUTO_DATALOG_DONE.vi"("Enum"=enum16{"Read", "Write"}."Write", "error in (no error)"=w280, "I/P"=u16 2) -> ("error out"=w282:errorcluster)  [unwired: 7 in, 1 out]
                n111 = flat-sequence {
                  tunnel: [w285] -> w281
                  tunnel: w282 -> [w285]
                  frame #0 {
                    n112 = global write "DATA LOG.vi" "OP 10 DATA LOG RESULT"(TRUE ("DATA LOG RESET")) -> ()
                  }
                }
              }
              frame Enabled {
              }
            }
          }
          frame "SCAN2" {
            # "Barcode Status\n0-Ideal, 1-Ok, 2-Nok, 3-Prev Station Not Done,\n4-Prev Station Nok,\n5- Already Done"
            # "STATION OP 20"
            n113 = case shown="False" w344 {
              tunnel: w348 -> [w372 w412]
              tunnel: w347 -> [w364 w410]
              tunnel: w346 -> [_ _]
              tunnel: [w367 w409] -> w343
              tunnel: [w365 w412] -> w345
              tunnel: [w349 "" ("trimmed string")] -> w336
              frame False {
                # "2 FOR EMPTY BARCODE READ OR MISMATCH"
                n114 = call "PADMINI_AUTO_BARCODE_STRING2.vi"("Enum"=enum16{"Read", "Write"}."Read", "error in (no error)"=w364) -> ("error out"=w363:errorcluster, "Input 2"=w351:string[])  [unwired: 8 in]
                n115 = global read "Global 1.vi" "BARCODE RECIPE"() -> (w352:string)
                n116 = Index Array(array=w351) -> (element=w350:string)  [unwired: 1 in]
                n117 = call <vilib>:"Trim Whitespace.vi"("string"=w350) -> ("trimmed string"=w349:string)  [unwired: 1 in]
                n118 = Match Pattern(string=w349, regular expression=w352) -> (match substring=w353:string)  [unwired: 1 in, 3 out]
                n119 = String Length(string=w352) -> (length=w355:i32)
                n120 = String Length(string=w353) -> (length=w354:i32)
                n121 = Format Into String(format string="WHERE BARCODE  ='%s'", w349) -> (resulting string=w359:string)  [unwired: 2 in, 1 out]
                n122 = Equal?(x=w355, y=w354) -> (x = y?=w356:bool)
                n123 = call <vilib>:"DB Tools Select Data.vi"("condition"=w359, "error in (no error)"=w363, "columns"=string[] ["BARCODE", "ST1_FINAL_RST", "ST2_FINAL_RST"], "table"="REPORT", "connection reference"=w372) -> ("error out"=w370:errorcluster, "data"=w369:variant[][], "connection reference out"=w365:T13)  [unwired: 1 in]
                n124 = call "PADMINI_varient_to_data.vi"("error in (no error)"=w370, "data"=w369) -> ("error out"=w368:errorcluster, "Array"=w366:string[][])  [unwired: 8 in]
                n125 = Equal?(x=w349, y="") -> (x = y?=w357:bool)
                n126 = case shown="False" w357 {
                  selector: w357 -> [_ w406]
                  tunnel: w368 -> [w376 w405]
                  tunnel: [w375 w404] -> w367
                  tunnel: w366 -> [w374 _]
                  tunnel: w356 -> [w373 _]
                  frame False {
                    n127 = case shown="True" w373 {
                      tunnel: w376 -> [w379 w394]
                      tunnel: [w378 w401] -> w375
                      tunnel: w374 -> [_ w400]
                      frame False {
                        w377 = i32[] [0, 1, 0, 0, 0]  # I/P
                        n128 = call "PADMINI_AUTO_BARCODE_STATUS 20.vi"("Enum"=enum16{"Read", "Write"}."Write", "error in (no error)"=w379, "I/P"=w377) -> ("error out"=w378:errorcluster)  [unwired: 7 in, 1 out]
                      }
                      frame True {
                        # "ST2 RESULT"
                        # "ST1 RESULT"
                        n129 = Index Array(array=w400, index (row) #1=0 ("index (row)"), index (col) #1=1 ("disabled index (col)"), index (row) #2=0 ("index (row)"), index (col) #2=2 ("disabled index (col)")) -> (element #1=w393:string)  [unwired: 1 out]
                        n130 = Empty String/Path?(string/path=w393) -> (empty?=w391:bool)
                        n131 = Equal?(x=w393, y="OK") -> (x = y?=w387:bool)
                        n132 = Boolean To (0,1)(Boolean=FALSE ("element")) -> (0, 1=w384:i16)
                        n133 = Boolean To (0,1)(Boolean=TRUE ("element")) -> (0, 1=w385:i16)
                        n134 = Not(x=w387) -> (.not. x?=w386:bool)
                        n135 = Boolean To (0,1)(Boolean=w391) -> (0, 1=w383:i16)
                        n136 = Boolean To (0,1)(Boolean=w387) -> (0, 1=w382:i16)
                        n137 = Boolean To (0,1)(Boolean=w386) -> (0, 1=w381:i16)
                        n138 = Build Array(w385, w384, w383, w382, w381) -> (w390:i16[])
                        n139 = call "PADMINI_AUTO_BARCODE_STATUS 20.vi"("Enum"=enum16{"Read", "Write"}."Write", "error in (no error)"=w394, "I/P"=w390) -> ("error out"=w401:errorcluster)  [unwired: 7 in, 1 out]
                      }
                    }
                  }
                  frame True {
                    w402 = i32[] [0, 0, 0, 0, 0]  # I/P
                    n140 = call "PADMINI_AUTO_BARCODE_STATUS 20.vi"("Enum"=enum16{"Read", "Write"}."Write", "error in (no error)"=w405, "I/P"=w402) -> ("error out"=w404:errorcluster)  [unwired: 7 in, 1 out]
                    "OP30 BARCODE STRING EMPRTY" <- w406
                  }
                }
              }
              frame True {
                w407 = i32[] [0, 0, 0, 0, 0]  # I/P
                n141 = call "PADMINI_AUTO_BARCODE_STATUS 20.vi"("Enum"=enum16{"Read", "Write"}."Write", "error in (no error)"=w410, "I/P"=w407) -> ("error out"=w409:errorcluster)  [unwired: 7 in, 1 out]
              }
            }
            n142 = flat-sequence {
              tunnel: [w414] -> w342
              tunnel: w343 -> [w414]
              frame #0 {
                # "UPDATE op 20 SCAN sTATUS"
                n143 = global write "DATA LOG.vi" "OP 20 Outputs"(TRUE) -> ()
              }
            }
            n144 = Bundle By Name(cluster=w338, "OP - 20.BARCODE"=w336) -> (w337:T11)
          }
          frame "DATALOG2" {
            w445 = T14 2 items=["no dialog", "OK message", "continue or stop message", "OK message + warnings", "continue/stop + warnings"] ("type of dialog (OK msg:1)")
            # "Printed QR Code data string"
            # "datalog of OP 20"
            n145 = call "PADMINI_AUTO_BARCODE_STRING2.vi"("Enum"=enum16{"Read", "Write"}."Read", "error in (no error)"=w432) -> ("error out"=w434:errorcluster, "Input 2"=w416:string[])  [unwired: 8 in]
            n146 = call "PADMINI_AUTO_CYCLE VALUE 20.vi"("Enum"=enum16{"Read", "Write"}."Read", "error in (no error)"=w432) -> ("Input 2"=w426:dbl[])  [unwired: 8 in, 1 out]
            n147 = Index Array(array=w426) -> (element #1=w431:dbl, element #2=w430:dbl, element #3=w429:dbl, element #4=w428:dbl)  [unwired: 4 in]
            n148 = Number To Fractional String(number=w426, precision (6)=i16 2) -> (F-format string=w425:string[])  [unwired: 2 in]
            n149 = case shown="False" w450 {
              tunnel: w451 -> [w487 w513]
              tunnel: w434 -> [w488 w512]
              tunnel: [w491 w511] -> w448
              tunnel: [w490 w510] -> w446
              tunnel: w449 -> [w486 _]
              tunnel: w425 -> [w482 w495]
              tunnel: w416 -> [w474 w496]
              frame False {
                # "ST2 RESULT"
                # "DO TRACEBILITY"
                n150 = Index Array(array=w474) -> (element #1=w475:string, element #2=w473:string, element #3=w472:string, element #4=w471:string, element #5=w470:string, element #6=w469:string, element #7=w468:string)  [unwired: 7 in]
                n151 = local read "SHIFT"() -> (w489:string)
                n152 = Index Array(array=w482) -> (element #1=w481:string, element #2=w480:string, element #3=w479:string, element #4=w478:string)  [unwired: 4 in]
                n153 = call <vilib>:"Trim Whitespace.vi"("string"=w475) -> ("trimmed string"=w476:string)  [unwired: 1 in]
                n154 = call "PADMINI_SHIFT_DATE.vi"("SHIFT"=w489) -> ("date/time string"=w467:string)  [unwired: 10 in]
                n155 = Format Into String(format string="Where BARCODE='%s' ", w476) -> (resulting string=w484:string)  [unwired: 2 in, 1 out]
                n156 = Bundle("date/time string"=w467, "Input 2"=w481, "Input 2"=w480, "Input 2"=w473, "Input 2"=w472, "Input 2"=w479, "Input 2"=w478, "Input 2"=w471, "Input 2"=w470, "Input 2"=w469, "Input 2"=w468) -> (w477:T17)  [unwired: 1 in]
                n157 = call <vilib>:"DB Tools Update Data.vi"("condition"=w484, "data"=w477, "error in (no error)"=w488, "columns"=string[] ["DATEST2", "ST2_LOWER_BEARING_DIS", "ST2_LOWER_BEARING_LOAD", "ST2_BOTTOM_CAMERA_STATUS", "ST2_LOWER_BEARING_RST", "ST2_UPPER_BEARING_DIS", "ST2_UPPER_BEARING_LOAD", "ST2_UPPER_SIM_STATUS", "ST2_UPPER_CAMERA_STATUS", "ST2_UPPER_BERAING_RST", "ST2_FINAL_RST"], "table"=w486, "connection reference"=w487) -> ("error out"=w490:errorcluster, "connection reference out"=w491:T13)  [unwired: 4 in]
              }
              frame True {
                n158 = local read "SHIFT"() -> (w493:string)
                n159 = Index Array(array=w496) -> (element #2=w502:string, element #3=w501:string, element #4=w500:string, element #5=w499:string, element #6=w498:string, element #7=w492:string)  [unwired: 7 in, 1 out]
                n160 = call "PADMINI_SHIFT_DATE.vi"("SHIFT"=w493) -> ("date/time string"=w494:string)  [unwired: 10 in]
                n161 = Index Array(array=w495) -> (element #1=w506:string, element #2=w505:string, element #3=w504:string, element #4=w503:string)  [unwired: 4 in]
                n162 = Bundle("date/time string"=w494, "SHIFT"=w493, "Input 2"=w506, "Input 2"=w505, "Input 2"=w502, "Input 2"=w501, "Input 2"=w504, "Input 2"=w503, "Input 2"=w500, "Input 2"=w499, "Input 2"=w498, "Input 2"=w492) -> (w497:T18)  [unwired: 1 in]
                n163 = To Variant(anything=w497) -> (Variant=w508:variant)
                n164 = call <vilib>:"DB Tools Insert Data.vi"("data"=w508, "error in (no error)"=w512, "columns"=string[] ["DATE", "SHIFT", "ST2_LOWER_BEARING_DIS", "ST2_LOWER_BEARING_LOAD", "ST2_BOTTOM_CAMERA_STATUS", "ST2_LOWER_BEARING_RST", "ST2_UPPER_BEARING_DIS", "ST2_UPPER_BEARING_LOAD", "ST2_UPPER_SIM_STATUS", "ST2_UPPER_CAMERA_STATUS", "ST2_UPPER_BERAING_RST", "ST2_FINAL_RST"], "table"="ST2_REPORT", "connection reference"=w513) -> ("error out"=w510:errorcluster, "connection reference out"=w511:T13)  [unwired: 5 in]
              }
            }
            n165 = Bundle By Name(cluster=w437, "OP - 20.LOWERING BEARING DISPLACE"=w431, "OP - 20.LOWERING BEARING LOAD"=w430, "OP - 20.UPPER BEARING DISPLACE"=w429, "OP - 20.UPPER BEARING LOAD"=w428) -> (w436:T11)
            n166 = call <vilib>:"Simple Error Handler.vi"("type of dialog (OK msg:1)"=w445, "error in (no error)"=w446) -> ("error out"=w444:errorcluster)  [unwired: 3 in, 4 out]
            n167 = call <vilib>:"Clear Errors.vi"("error in (no error)"=w444) -> ("error out"=w442:errorcluster)  [unwired: 5 in, 1 out]
            n168 = property on="OP - 20" class="Clust"(error in=w442) -> (error out=w439:errorcluster, "Controls[]"=w441:refnum<vi>[])  [unwired: 1 in, 1 out]
            n169 = for {
              tunnel: w416 -> [w456] mode=indexing
              tunnel: [w455] -> w415 mode=indexing if=w453
              i -> [w454]
              n170 = case shown="\"NG\"" w456 {
                tunnel: [2 ("CYCLE STATUS OK, NOK, ABORTED") 1 ("CYCLE STATUS OK, NOK, ABORTED") 0 ("CYCLE STATUS OK, NOK, ABORTED")] -> w455
                frame "NG" {
                }
                frame "OK" {
                }
                frame "-1", Default {
                }
              }
              n171 = Not Equal To 0?(x=w454) -> (x != 0?=w453:bool)
            }
            n172 = Index Array(array=w441, index #1=3 ("index"), index #3=7 ("index")) -> (element #1=w423:refnum<vi>, element #2=w422:refnum<vi>, element #3=w421:refnum<vi>, element #4=w420:refnum<vi>, element #5=w419:refnum<vi>, element #6=w418:refnum<vi>)  [unwired: 4 in]
            n173 = Build Array(w423, w422, w421, w420, w419, w418) -> (w417:refnum<vi>[])
            n174 = for {
              tunnel: w417 -> [w465] mode=indexing
              shift-right: [w461] -> w438
              shift-left: w439 -> [w463]
              tunnel: w415 -> [w460] mode=indexing
              w464 = refnum<vi> refnum  # Boolean
              n175 = To More Specific Class(target class=w464, reference=w465, error in=w463) -> (specific class reference=w466:refnum<vi>, error out=w462:errorcluster)
              n176 = call "PADMINI_BOOL_COLOR_CHANGE.vi"("error in (no error)"=w462, "Numeric"=w460, "Boolean in"=w466) -> ("error out"=w461:errorcluster)  [unwired: 8 in]
            }
          }
          frame "SCAN3" {
            # "STATION OP 30"
            n177 = case shown="False" w522 {
              tunnel: w526 -> [w550 w590]
              tunnel: w525 -> [w542 w588]
              tunnel: w524 -> [_ _]
              tunnel: [w545 w587] -> w521
              tunnel: [w543 w590] -> w523
              tunnel: [w527 "" ("trimmed string")] -> w514
              frame False {
                n178 = call "PADMINI_AUTO_BARCODE_STRING 30.vi"("Enum"=enum16{"Read", "Write"}."Read", "error in (no error)"=w542) -> ("error out"=w541:errorcluster, "Input 2"=w529:string[])  [unwired: 8 in]
                n179 = global read "Global 1.vi" "BARCODE RECIPE"() -> (w530:string)
                n180 = Index Array(array=w529) -> (element=w528:string)  [unwired: 1 in]
                n181 = call <vilib>:"Trim Whitespace.vi"("string"=w528) -> ("trimmed string"=w527:string)  [unwired: 1 in]
                n182 = Match Pattern(string=w527, regular expression=w530) -> (match substring=w531:string)  [unwired: 1 in, 3 out]
                n183 = String Length(string=w530) -> (length=w533:i32)
                n184 = String Length(string=w531) -> (length=w532:i32)
                n185 = Format Into String(format string="WHERE BARCODE  ='%s'", w527) -> (resulting string=w537:string)  [unwired: 2 in, 1 out]
                n186 = Equal?(x=w533, y=w532) -> (x = y?=w534:bool)
                n187 = call <vilib>:"DB Tools Select Data.vi"("condition"=w537, "error in (no error)"=w541, "columns"=string[] ["BARCODE", "ST2_FINAL_RST", "ST3_FINAL_RST"], "table"="REPORT", "connection reference"=w550) -> ("error out"=w548:errorcluster, "data"=w547:variant[][], "connection reference out"=w543:T13)  [unwired: 1 in]
                n188 = call "PADMINI_varient_to_data.vi"("error in (no error)"=w548, "data"=w547) -> ("error out"=w546:errorcluster, "Array"=w544:string[][])  [unwired: 8 in]
                n189 = Equal?(x=w527, y="") -> (x = y?=w535:bool)
                n190 = case shown="True" w535 {
                  selector: w535 -> [_ w584]
                  tunnel: w546 -> [w554 w583]
                  tunnel: [w553 w582] -> w545
                  tunnel: w544 -> [w552 _]
                  tunnel: w534 -> [w551 _]
                  frame False {
                    n191 = case shown="False" w551 {
                      tunnel: w554 -> [w557 w572]
                      tunnel: [w556 w579] -> w553
                      tunnel: w552 -> [_ w578]
                      frame False {
                        w555 = i32[] [0, 1, 0, 0, 0]  # I/P
                        n192 = call "PADMINI_AUTO_BARCODE_STATUS 30.vi"("Enum"=enum16{"Read", "Write"}."Write", "error in (no error)"=w557, "I/P"=w555) -> ("error out"=w556:errorcluster)  [unwired: 7 in, 1 out]
                      }
                      frame True {
                        n193 = Index Array(array=w578, index (row) #1=0 ("index (row)"), index (col) #1=1 ("disabled index (col)"), index (row) #2=0 ("index (row)"), index (col) #2=2 ("disabled index (col)")) -> (element #1=w571:string)  [unwired: 1 out]
                        n194 = Empty String/Path?(string/path=w571) -> (empty?=w569:bool)
                        n195 = Equal?(x=w571, y="OK") -> (x = y?=w566:bool)
                        n196 = Boolean To (0,1)(Boolean=FALSE ("element")) -> (0, 1=w563:i16)
                        n197 = Boolean To (0,1)(Boolean=w569) -> (0, 1=w562:i16)
                        n198 = Boolean To (0,1)(Boolean=TRUE ("element")) -> (0, 1=w564:i16)
                        n199 = Not(x=w566) -> (.not. x?=w565:bool)
                        n200 = Boolean To (0,1)(Boolean=w566) -> (0, 1=w561:i16)
                        n201 = Boolean To (0,1)(Boolean=w565) -> (0, 1=w560:i16)
                        n202 = Build Array(w564, w563, w562, w561, w560) -> (w559:i16[])
                        n203 = call "PADMINI_AUTO_BARCODE_STATUS 30.vi"("Enum"=enum16{"Read", "Write"}."Write", "error in (no error)"=w572, "I/P"=w559) -> ("error out"=w579:errorcluster)  [unwired: 7 in, 1 out]
                      }
                    }
                  }
                  frame True {
                    w580 = i32[] [0, 0, 0, 0, 0]  # I/P
                    n204 = call "PADMINI_AUTO_BARCODE_STATUS 30.vi"("Enum"=enum16{"Read", "Write"}."Write", "error in (no error)"=w583, "I/P"=w580) -> ("error out"=w582:errorcluster)  [unwired: 7 in, 1 out]
                    "OP30 BARCODE STRING EMPRTY 2" <- w584
                  }
                }
              }
              frame True {
                w585 = i32[] [0, 0, 0, 0, 0]  # I/P
                n205 = call "PADMINI_AUTO_BARCODE_STATUS 30.vi"("Enum"=enum16{"Read", "Write"}."Write", "error in (no error)"=w588, "I/P"=w585) -> ("error out"=w587:errorcluster)  [unwired: 7 in, 1 out]
              }
            }
            n206 = flat-sequence {
              tunnel: [w593] -> w520
              tunnel: w521 -> [w593]
              frame #0 {
                # "UPDATE op 30 SCAN sTATUS"
                n207 = local write "OP30 BARCODE STRING EMPRTY 2"(FALSE ("Boolean 5")) -> ()
                n208 = global write "DATA LOG.vi" "OP 30 Outputs"(TRUE) -> ()
              }
            }
            n209 = Bundle By Name(cluster=w516, "OP - 30.BARCODE"=w514) -> (w515:T11)
          }
          frame "DATALOG3" {
            w618 = T14 2 items=["no dialog", "OK message", "continue or stop message", "OK message + warnings", "continue/stop + warnings"] ("type of dialog (OK msg:1)")
            # "Printed QR Code data string"
            # "datalog of OP 30"
            n210 = call "PADMINI_AUTO_BARCODE_STRING 30.vi"("Enum"=enum16{"Read", "Write"}."Read", "error in (no error)"=w605) -> ("error out"=w607:errorcluster, "Input 2"=w596:string[])  [unwired: 8 in]
            n211 = call "PADMINI_AUTO_CYCLE VALUE 30.vi"("Enum"=enum16{"Read", "Write"}."Read", "error in (no error)"=w605) -> ("Input 2"=w601:dbl[])  [unwired: 8 in, 1 out]
            n212 = Index Array(array=w601) -> (element #1=w604:dbl, element #2=w603:dbl)  [unwired: 2 in]
            n213 = Number To Fractional String(number=w601, precision (6)=i16 2) -> (F-format string=w600:string[])  [unwired: 2 in]
            n214 = case shown="False" w623 {
              tunnel: w624 -> [w654 w674]
              tunnel: w607 -> [w655 w673]
              tunnel: [w658 w672] -> w621
              tunnel: [w657 w671] -> w619
              tunnel: w622 -> [w653 _]
              tunnel: w600 -> [w649 w659]
              tunnel: w596 -> [w643 w660]
              frame False {
                # "DO TRACEBILITY"
                n215 = Index Array(array=w643) -> (element #1=w644:string, element #2=w642:string, element #3=w641:string)  [unwired: 3 in]
                n216 = local read "SHIFT"() -> (w656:string)
                n217 = Index Array(array=w649) -> (element #1=w648:string, element #2=w647:string)  [unwired: 2 in]
                n218 = call <vilib>:"Trim Whitespace.vi"("string"=w644) -> ("trimmed string"=w645:string)  [unwired: 1 in]
                n219 = call "PADMINI_SHIFT_DATE.vi"("SHIFT"=w656) -> ("date/time string"=w640:string)  [unwired: 10 in]
                n220 = Format Into String(format string="Where BARCODE='%s' ", w645) -> (resulting string=w651:string)  [unwired: 2 in, 1 out]
                n221 = Bundle("date/time string"=w640, "Input 2"=w648, "Input 2"=w647, "Input 2"=w642, "Input 2"=w641) -> (w646:T19)  [unwired: 1 in]
                n222 = call <vilib>:"DB Tools Update Data.vi"("condition"=w651, "data"=w646, "error in (no error)"=w655, "columns"=string[] ["DATEST3", "ST3_DISPLACEMENT", "ST3_LOAD", "ST3_MIDDLE_GEAR_SHAFT_STATUS", "ST3_FINAL_RST"], "table"=w653, "connection reference"=w654) -> ("error out"=w657:errorcluster, "connection reference out"=w658:T13)  [unwired: 4 in]
              }
              frame True {
                # "TRAC BYPASS"
                n223 = local read "SHIFT"() -> (w661:string)
                n224 = call "PADMINI_SHIFT_DATE.vi"("SHIFT"=w661) -> ("date/time string"=w662:string)  [unwired: 10 in]
                n225 = Index Array(array=w660) -> (element #2=w666:string, element #3=w665:string)  [unwired: 3 in, 1 out]
                n226 = Index Array(array=w659) -> (element #1=w668:string, element #2=w667:string)  [unwired: 2 in]
                n227 = Bundle("date/time string"=w662, "SHIFT"=w661, "Input 2"=w668, "Input 2"=w667, "Input 2"=w666, "Input 2"=w665) -> (w663:T20)  [unwired: 1 in]
                n228 = To Variant(anything=w663) -> (Variant=w664:variant)
                n229 = call <vilib>:"DB Tools Insert Data.vi"("data"=w664, "error in (no error)"=w673, "columns"=string[] ["DATE", "SHIFT", "ST3_DISPLACEMENT", "ST3_LOAD", "ST3_MIDDLE_GEAR_SHAFT_STATUS", "ST3_FINAL_RST"], "table"="ST3_REPORT", "connection reference"=w674) -> ("error out"=w671:errorcluster, "connection reference out"=w672:T13)  [unwired: 5 in]
              }
            }
            n230 = Bundle By Name(cluster=w610, "OP - 30.Displacement"=w604, "OP - 30.Load"=w603) -> (w609:T11)
            n231 = call <vilib>:"Simple Error Handler.vi"("type of dialog (OK msg:1)"=w618, "error in (no error)"=w619) -> ("error out"=w617:errorcluster)  [unwired: 3 in, 4 out]
            n232 = call <vilib>:"Clear Errors.vi"("error in (no error)"=w617) -> ("error out"=w615:errorcluster)  [unwired: 5 in, 1 out]
            n233 = property on="OP - 30" class="Clust"(error in=w615) -> (error out=w612:errorcluster, "Controls[]"=w614:refnum<vi>[])  [unwired: 1 in, 1 out]
            n234 = for {
              tunnel: w596 -> [w629] mode=indexing
              tunnel: [w628] -> w595 mode=indexing if=w626
              i -> [w627]
              n235 = case shown="\"NG\"" w629 {
                tunnel: [2 ("CYCLE STATUS OK, NOK, ABORTED") 1 ("CYCLE STATUS OK, NOK, ABORTED") 0 ("CYCLE STATUS OK, NOK, ABORTED")] -> w628
                frame "NG" {
                }
                frame "OK" {
                }
                frame "-1", Default {
                }
              }
              n236 = Not Equal To 0?(x=w627) -> (x != 0?=w626:bool)
            }
            n237 = Index Array(array=w614, index #1=3 ("index"), index #2=4 ("index")) -> (element #1=w599:refnum<vi>, element #2=w598:refnum<vi>)
            n238 = Build Array(w599, w598) -> (w597:refnum<vi>[])
            n239 = for {
              tunnel: w597 -> [w638] mode=indexing
              shift-right: [w634] -> w611
              shift-left: w612 -> [w636]
              tunnel: w595 -> [w633] mode=indexing
              w637 = refnum<vi> refnum  # Boolean
              n240 = To More Specific Class(target class=w637, reference=w638, error in=w636) -> (specific class reference=w639:refnum<vi>, error out=w635:errorcluster)
              n241 = call "PADMINI_BOOL_COLOR_CHANGE.vi"("error in (no error)"=w635, "Numeric"=w633, "Boolean in"=w639) -> ("error out"=w634:errorcluster)  [unwired: 8 in]
            }
          }
          frame "SCAN4" {
            # "STATION OP 40"
            n242 = case shown="False" w683 {
              tunnel: w687 -> [w711 w750]
              tunnel: w686 -> [w703 w749]
              tunnel: w685 -> [_ _]
              tunnel: [w706 w748] -> w682
              tunnel: [w704 w750] -> w684
              tunnel: [w688 "" ("trimmed string")] -> w675
              frame False {
                n243 = call "PADMINI_AUTO_BARCODE_STRING 40.vi"("Enum"=enum16{"Read", "Write"}."Read", "error in (no error)"=w703) -> ("error out"=w702:errorcluster, "Input 2"=w690:string[])  [unwired: 8 in]
                n244 = global read "Global 1.vi" "BARCODE RECIPE"() -> (w691:string)
                n245 = Index Array(array=w690) -> (element=w689:string)  [unwired: 1 in]
                n246 = call <vilib>:"Trim Whitespace.vi"("string"=w689) -> ("trimmed string"=w688:string)  [unwired: 1 in]
                n247 = Match Pattern(string=w688, regular expression=w691) -> (match substring=w692:string)  [unwired: 1 in, 3 out]
                n248 = String Length(string=w691) -> (length=w694:i32)
                n249 = String Length(string=w692) -> (length=w693:i32)
                n250 = Format Into String(format string="WHERE BARCODE  ='%s'", w688) -> (resulting string=w698:string)  [unwired: 2 in, 1 out]
                n251 = Equal?(x=w694, y=w693) -> (x = y?=w695:bool)
                n252 = call <vilib>:"DB Tools Select Data.vi"("condition"=w698, "error in (no error)"=w702, "columns"=string[] ["BARCODE", "ST3_FINAL_RST", "ST4_FINAL_RST"], "table"="REPORT", "connection reference"=w711) -> ("error out"=w709:errorcluster, "data"=w708:variant[][], "connection reference out"=w704:T13)  [unwired: 1 in]
                n253 = call "PADMINI_varient_to_data.vi"("error in (no error)"=w709, "data"=w708) -> ("error out"=w707:errorcluster, "Array"=w705:string[][])  [unwired: 8 in]
                n254 = Equal?(x=w688, y="") -> (x = y?=w696:bool)
                n255 = case shown="False" w696 {
                  tunnel: w707 -> [w715 w744]
                  tunnel: [w714 w743] -> w706
                  tunnel: w705 -> [w713 _]
                  tunnel: w695 -> [w712 _]
                  frame False {
                    n256 = case shown="True" w712 {
                      tunnel: w715 -> [w719 w728]
                      tunnel: [w718 w727] -> w714
                      tunnel: w713 -> [_ w740]
                      frame False {
                        w716 = i32[] [0, 0, 0, 0, 0]  # I/P
                        n257 = call "PADMINI_AUTO_BARCODE_STATUS 40.vi"("Enum"=enum16{"Read", "Write"}."Write", "error in (no error)"=w719, "I/P"=w716) -> ("error out"=w718:errorcluster)  [unwired: 7 in, 1 out]
                      }
                      frame True {
                        n258 = Index Array(array=w740, index (row) #1=0 ("index (row)"), index (col) #1=1 ("disabled index (col)"), index (row) #2=0 ("index (row)"), index (col) #2=2 ("disabled index (col)")) -> (element #1=w734:string)  [unwired: 1 out]
                        n259 = Empty String/Path?(string/path=w734) -> (empty?=w732:bool)
                        n260 = Equal?(x=w734, y="OK") -> (x = y?=w730:bool)
                        n261 = Boolean To (0,1)(Boolean=FALSE ("element")) -> (0, 1=w724:i16)
                        n262 = Boolean To (0,1)(Boolean=w732) -> (0, 1=w723:i16)
                        n263 = Boolean To (0,1)(Boolean=TRUE ("element")) -> (0, 1=w725:i16)
                        n264 = Not(x=w730) -> (.not. x?=w729:bool)
                        n265 = Boolean To (0,1)(Boolean=w730) -> (0, 1=w722:i16)
                        n266 = Boolean To (0,1)(Boolean=w729) -> (0, 1=w721:i16)
                        n267 = Build Array(w725, w724, w723, w722, w721) -> (w720:i16[])
                        n268 = call "PADMINI_AUTO_BARCODE_STATUS 40.vi"("Enum"=enum16{"Read", "Write"}."Write", "error in (no error)"=w728, "I/P"=w720) -> ("error out"=w727:errorcluster)  [unwired: 7 in, 1 out]
                      }
                    }
                  }
                  frame True {
                    w741 = i32[] [0, 0, 0, 0, 0]  # I/P
                    n269 = call "PADMINI_AUTO_BARCODE_STATUS 40.vi"("Enum"=enum16{"Read", "Write"}."Write", "error in (no error)"=w744, "I/P"=w741) -> ("error out"=w743:errorcluster)  [unwired: 7 in, 1 out]
                  }
                }
              }
              frame True {
                w745 = i32[] [0, 0, 0, 0, 0]  # I/P
                n270 = call "PADMINI_AUTO_BARCODE_STATUS 40.vi"("Enum"=enum16{"Read", "Write"}."Write", "error in (no error)"=w749, "I/P"=w745) -> ("error out"=w748:errorcluster)  [unwired: 7 in, 1 out]
              }
            }
            n271 = flat-sequence {
              tunnel: [w752] -> w681
              tunnel: w682 -> [w752]
              frame #0 {
                # "UPDATE op 40 SCAN sTATUS"
                n272 = global write "DATA LOG.vi" "OP 40 Outputs"(TRUE) -> ()
              }
            }
            n273 = Bundle By Name(cluster=w677, "OP - 40.BARCODE"=w675) -> (w676:T11)
          }
          frame "DATALOG4" {
            w783 = T14 2 items=["no dialog", "OK message", "continue or stop message", "OK message + warnings", "continue/stop + warnings"] ("type of dialog (OK msg:1)")
            # "datalog of OP 40"
            n274 = call "PADMINI_AUTO_BARCODE_STRING 40.vi"("Enum"=enum16{"Read", "Write"}."Read", "error in (no error)"=w770) -> ("error out"=w772:errorcluster, "Input 2"=w761:string[])  [unwired: 8 in]
            n275 = call "PADMINI_AUTO_CYCLE VALUE 40.vi"("Enum"=enum16{"Read", "Write"}."Read", "error in (no error)"=w770) -> ("Input 2"=w766:dbl[])  [unwired: 8 in, 1 out]
            n276 = Index Array(array=w766) -> (element #1=w769:dbl, element #2=w768:dbl, element #3=w758:dbl, element #4=w757:dbl)  [unwired: 4 in]
            n277 = Number To Fractional String(number=w766, precision (6)=i16 2) -> (F-format string=w765:string[])  [unwired: 2 in]
            n278 = case shown="False" w788 {
              tunnel: w789 -> [w823 w847]
              tunnel: w772 -> [w824 w846]
              tunnel: [w827 w845] -> w786
              tunnel: [w826 w844] -> w784
              tunnel: w787 -> [w822 _]
              tunnel: w765 -> [w818 w829]
              tunnel: w761 -> [w813 w828]
              frame False {
                # "DO TRACEBILITY"
                n279 = Index Array(array=w813) -> (element #1=w814:string, element #2=w809:string, element #3=w808:string, element #4=w807:string, element #5=w806:string)  [unwired: 5 in]
                n280 = local read "SHIFT"() -> (w825:string)
                n281 = Index Array(array=w818) -> (element #1=w817:string, element #2=w812:string, element #3=w811:string, element #4=w810:string)  [unwired: 4 in]
                n282 = call <vilib>:"Trim Whitespace.vi"("string"=w814) -> ("trimmed string"=w815:string)  [unwired: 1 in]
                n283 = call "PADMINI_SHIFT_DATE.vi"("SHIFT"=w825) -> ("date/time string"=w805:string)  [unwired: 10 in]
                n284 = Format Into String(format string="Where BARCODE='%s' ", w815) -> (resulting string=w820:string)  [unwired: 2 in, 1 out]
                n285 = Bundle("date/time string"=w805, "Input 2"=w817, "Input 2"=w809, "Input 2"=w812, "Input 2"=w808, "Input 2"=w811, "Input 2"=w810, "Input 2"=w806, "Input 2"=w807) -> (w816:T21)  [unwired: 1 in]
                n286 = call <vilib>:"DB Tools Update Data.vi"("condition"=w820, "data"=w816, "error in (no error)"=w824, "columns"=string[] ["DATEST4", "ST4_SCREW1_DATA", "ST4_SCREW1_STATUS", "ST4_SCREW2_DATA", "ST4_SCREW2_STATUS", "ST4_DISPLACEMENT", "ST4_LOAD", "ST4_TOP_BEARING_CAMERA_STAUS", "ST4_FINAL_RST"], "table"=w822, "connection reference"=w823) -> ("error out"=w826:errorcluster, "connection reference out"=w827:T13)  [unwired: 4 in]
              }
              frame True {
                # "TRAC BYPASS"
                n287 = local read "SHIFT"() -> (w830:string)
                n288 = Index Array(array=w828) -> (element #2=w838:string, element #3=w837:string, element #4=w836:string, element #5=w835:string)  [unwired: 5 in, 1 out]
                n289 = call "PADMINI_SHIFT_DATE.vi"("SHIFT"=w830) -> ("date/time string"=w831:string)  [unwired: 10 in]
                n290 = Index Array(array=w829) -> (element #1=w832:string, element #2=w841:string, element #3=w840:string, element #4=w839:string)  [unwired: 4 in]
                n291 = Bundle("date/time string"=w831, "SHIFT"=w830, "Input 2"=w832, "Input 2"=w838, "Input 2"=w841, "Input 2"=w837, "Input 2"=w840, "Input 2"=w839, "Input 2"=w835, "Input 2"=w836) -> (w834:T22)  [unwired: 1 in]
                n292 = To Variant(anything=w834) -> (Variant=w833:variant)
                n293 = call <vilib>:"DB Tools Insert Data.vi"("data"=w833, "error in (no error)"=w846, "columns"=string[] ["DATE", "SHIFT", "ST4_SCREW1_DATA", "ST4_SCREW1_STATUS", "ST4_SCREW2_DATA", "ST4_SCREW2_STATUS", "ST4_DISPLACEMENT", "ST4_LOAD", "ST4_TOP_BEARING_CAMERA_STAUS", "ST4_FINAL_RST"], "table"="ST4_REPORT", "connection reference"=w847) -> ("error out"=w844:errorcluster, "connection reference out"=w845:T13)  [unwired: 5 in]
              }
            }
            n294 = Bundle By Name(cluster=w775, "OP - 40.Screw 1 Data"=w769, "OP - 40.Screw 2 data"=w768, "OP - 40.Dispalcement"=w758, "OP - 40.Load"=w757) -> (w774:T11)
            n295 = call <vilib>:"Simple Error Handler.vi"("type of dialog (OK msg:1)"=w783, "error in (no error)"=w784) -> ("error out"=w782:errorcluster)  [unwired: 3 in, 4 out]
            n296 = call <vilib>:"Clear Errors.vi"("error in (no error)"=w782) -> ("error out"=w780:errorcluster)  [unwired: 5 in, 1 out]
            n297 = property on="OP - 40" class="Clust"(error in=w780) -> (error out=w777:errorcluster, "Controls[]"=w779:refnum<vi>[])  [unwired: 1 in, 1 out]
            n298 = for {
              tunnel: w761 -> [w794] mode=indexing
              tunnel: [w793] -> w760 mode=indexing if=w791
              i -> [w792]
              n299 = case shown="\"NG\"" w794 {
                tunnel: [2 ("CYCLE STATUS OK, NOK, ABORTED") 1 ("CYCLE STATUS OK, NOK, ABORTED") 0 ("CYCLE STATUS OK, NOK, ABORTED")] -> w793
                frame "NG" {
                }
                frame "OK" {
                }
                frame "-1", Default {
                }
              }
              n300 = Not Equal To 0?(x=w792) -> (x != 0?=w791:bool)
            }
            n301 = Index Array(array=w779, index #1=3 ("index"), index #2=4 ("index"), index #3=8 ("index"), index #4=7 ("index")) -> (element #1=w764:refnum<vi>, element #2=w763:refnum<vi>, element #3=w754:refnum<vi>, element #4=w753:refnum<vi>)
            n302 = Build Array(w764, w763, w754, w753) -> (w762:refnum<vi>[])
            n303 = for {
              tunnel: w762 -> [w803] mode=indexing
              shift-right: [w799] -> w776
              shift-left: w777 -> [w801]
              tunnel: w760 -> [w798] mode=indexing
              w802 = refnum<vi> refnum  # Boolean
              n304 = To More Specific Class(target class=w802, reference=w803, error in=w801) -> (specific class reference=w804:refnum<vi>, error out=w800:errorcluster)
              n305 = call "PADMINI_BOOL_COLOR_CHANGE.vi"("error in (no error)"=w800, "Numeric"=w798, "Boolean in"=w804) -> ("error out"=w799:errorcluster)  [unwired: 8 in]
            }
          }
          frame "SCAN5" {
            # "STATION OP 50"
            n306 = case shown="False" w856 {
              tunnel: w860 -> [w884 w923]
              tunnel: w859 -> [w876 w922]
              tunnel: w858 -> [_ _]
              tunnel: [w879 w921] -> w855
              tunnel: [w877 w923] -> w857
              tunnel: [w861 "" ("trimmed string")] -> w848
              frame False {
                n307 = call "PADMINI_AUTO_BARCODE_STRING 50.vi"("Enum"=enum16{"Read", "Write"}."Read", "error in (no error)"=w876) -> ("error out"=w875:errorcluster, "Input 2"=w863:string[])  [unwired: 8 in]
                n308 = global read "Global 1.vi" "BARCODE RECIPE"() -> (w864:string)
                n309 = Index Array(array=w863) -> (element=w862:string)  [unwired: 1 in]
                n310 = call <vilib>:"Trim Whitespace.vi"("string"=w862) -> ("trimmed string"=w861:string)  [unwired: 1 in]
                n311 = Match Pattern(string=w861, regular expression=w864) -> (match substring=w865:string)  [unwired: 1 in, 3 out]
                n312 = String Length(string=w864) -> (length=w867:i32)
                n313 = String Length(string=w865) -> (length=w866:i32)
                n314 = Format Into String(format string="WHERE BARCODE  ='%s'", w861) -> (resulting string=w871:string)  [unwired: 2 in, 1 out]
                n315 = Equal?(x=w867, y=w866) -> (x = y?=w868:bool)
                n316 = call <vilib>:"DB Tools Select Data.vi"("condition"=w871, "error in (no error)"=w875, "columns"=string[] ["BARCODE", "ST4_FINAL_RST", "ST5_FINAL_RST"], "table"="REPORT", "connection reference"=w884) -> ("error out"=w882:errorcluster, "data"=w881:variant[][], "connection reference out"=w877:T13)  [unwired: 1 in]
                n317 = call "PADMINI_varient_to_data.vi"("error in (no error)"=w882, "data"=w881) -> ("error out"=w880:errorcluster, "Array"=w878:string[][])  [unwired: 8 in]
                n318 = Equal?(x=w861, y="") -> (x = y?=w869:bool)
                n319 = case shown="False" w869 {
                  tunnel: w880 -> [w888 w917]
                  tunnel: [w887 w916] -> w879
                  tunnel: w878 -> [w886 _]
                  tunnel: w868 -> [w885 _]
                  frame False {
                    n320 = case shown="False" w885 {
                      tunnel: w888 -> [w892 w901]
                      tunnel: [w891 w900] -> w887
                      tunnel: w886 -> [_ w913]
                      frame False {
                        w889 = i32[] [0, 0, 0, 0, 0]  # I/P
                        n321 = call "PADMINI_AUTO_BARCODE_STATUS 50.vi"("Enum"=enum16{"Read", "Write"}."Write", "error in (no error)"=w892, "I/P"=w889) -> ("error out"=w891:errorcluster)  [unwired: 7 in, 1 out]
                      }
                      frame True {
                        n322 = Index Array(array=w913, index (row) #1=0 ("index (row)"), index (col) #1=1 ("disabled index (col)"), index (row) #2=0 ("index (row)"), index (col) #2=2 ("disabled index (col)")) -> (element #1=w907:string)  [unwired: 1 out]
                        n323 = Empty String/Path?(string/path=w907) -> (empty?=w905:bool)
                        n324 = Equal?(x=w907, y="OK") -> (x = y?=w903:bool)
                        n325 = Boolean To (0,1)(Boolean=FALSE ("element")) -> (0, 1=w897:i16)
                        n326 = Boolean To (0,1)(Boolean=w905) -> (0, 1=w896:i16)
                        n327 = Boolean To (0,1)(Boolean=TRUE ("element")) -> (0, 1=w898:i16)
                        n328 = Not(x=w903) -> (.not. x?=w902:bool)
                        n329 = Boolean To (0,1)(Boolean=w903) -> (0, 1=w895:i16)
                        n330 = Boolean To (0,1)(Boolean=w902) -> (0, 1=w894:i16)
                        n331 = Build Array(w898, w897, w896, w895, w894) -> (w893:i16[])
                        n332 = call "PADMINI_AUTO_BARCODE_STATUS 50.vi"("Enum"=enum16{"Read", "Write"}."Write", "error in (no error)"=w901, "I/P"=w893) -> ("error out"=w900:errorcluster)  [unwired: 7 in, 1 out]
                      }
                    }
                  }
                  frame True {
                    w914 = i32[] [0, 0, 0, 0, 0]  # I/P
                    n333 = call "PADMINI_AUTO_BARCODE_STATUS 50.vi"("Enum"=enum16{"Read", "Write"}."Write", "error in (no error)"=w917, "I/P"=w914) -> ("error out"=w916:errorcluster)  [unwired: 7 in, 1 out]
                  }
                }
              }
              frame True {
                w918 = i32[] [0, 0, 0, 0, 0]  # I/P
                n334 = call "PADMINI_AUTO_BARCODE_STATUS 50.vi"("Enum"=enum16{"Read", "Write"}."Write", "error in (no error)"=w922, "I/P"=w918) -> ("error out"=w921:errorcluster)  [unwired: 7 in, 1 out]
              }
            }
            n335 = flat-sequence {
              tunnel: [w925] -> w854
              tunnel: w855 -> [w925]
              frame #0 {
                # "UPDATE op 50 SCAN sTATUS"
                n336 = global write "DATA LOG.vi" "OP 50 Outputs"(TRUE) -> ()
              }
            }
            n337 = Bundle By Name(cluster=w850, "OP - 50.BARCODE"=w848) -> (w849:T11)
          }
          frame "DATALOG5" {
            w953 = T14 2 items=["no dialog", "OK message", "continue or stop message", "OK message + warnings", "continue/stop + warnings"] ("type of dialog (OK msg:1)")
            # "datalog of OP 50"
            n338 = call "PADMINI_AUTO_BARCODE_STRING 50.vi"("Enum"=enum16{"Read", "Write"}."Read", "error in (no error)"=w940) -> ("error out"=w942:errorcluster, "Input 2"=w931:string[])  [unwired: 8 in]
            n339 = call "PADMINI_AUTO_CYCLE VALUE 50.vi"("Enum"=enum16{"Read", "Write"}."Read", "error in (no error)"=w940) -> ("Input 2"=w936:dbl[])  [unwired: 8 in, 1 out]
            n340 = Index Array(array=w936) -> (element #1=w939:dbl, element #2=w938:dbl, element #3=w928:dbl)  [unwired: 3 in]
            n341 = Number To Fractional String(number=w936, precision (6)=i16 2) -> (F-format string=w935:string[])  [unwired: 2 in]
            n342 = case shown="False" w958 {
              tunnel: w959 -> [w991 w1013]
              tunnel: w942 -> [w992 w1012]
              tunnel: [w995 w1011] -> w956
              tunnel: [w994 w1010] -> w954
              tunnel: w957 -> [w990 _]
              tunnel: w935 -> [w986 w997]
              tunnel: w931 -> [w981 w996]
              frame False {
                # "DO TRACEBILITY"
                n343 = Index Array(array=w981) -> (element #1=w982:string, element #2=w978:string, element #3=w977:string, element #4=w976:string)  [unwired: 4 in]
                n344 = local read "SHIFT"() -> (w993:string)
                n345 = Index Array(array=w986) -> (element #1=w985:string, element #2=w980:string, element #3=w979:string)  [unwired: 3 in]
                n346 = call <vilib>:"Trim Whitespace.vi"("string"=w982) -> ("trimmed string"=w983:string)  [unwired: 1 in]
                n347 = call "PADMINI_SHIFT_DATE.vi"("SHIFT"=w993) -> ("date/time string"=w975:string)  [unwired: 10 in]
                n348 = Format Into String(format string="Where BARCODE='%s' ", w983) -> (resulting string=w988:string)  [unwired: 2 in, 1 out]
                n349 = Bundle("date/time string"=w975, "Input 2"=w985, "Input 2"=w978, "Input 2"=w980, "Input 2"=w977, "Input 2"=w979, "Input 2"=w976) -> (w984:T23)  [unwired: 1 in]
                n350 = call <vilib>:"DB Tools Update Data.vi"("condition"=w988, "data"=w984, "error in (no error)"=w992, "columns"=string[] ["DATEST5", "ST5_SCREW1_DATA", "ST5_SCREW1_STATUS", "ST5_SCREW2_DATA", "ST5_SCREW2_STATUS", "ST5_SCREW3_DATA", "ST5_FINAL_RST"], "table"=w990, "connection reference"=w991) -> ("error out"=w994:errorcluster, "connection reference out"=w995:T13)  [unwired: 4 in]
              }
              frame True {
                # "TRAC BYPASS"
                n351 = local read "SHIFT"() -> (w998:string)
                n352 = Index Array(array=w996) -> (element #2=w1002:string, element #3=w1001:string, element #4=w1006:string)  [unwired: 4 in, 1 out]
                n353 = Index Array(array=w997) -> (element #1=w1005:string, element #2=w1004:string, element #3=w1003:string)  [unwired: 3 in]
                n354 = call "PADMINI_SHIFT_DATE.vi"("SHIFT"=w998) -> ("date/time string"=w999:string)  [unwired: 10 in]
                n355 = Bundle("date/time string"=w999, "SHIFT"=w998, "Input 2"=w1005, "Input 2"=w1002, "Input 2"=w1004, "Input 2"=w1001, "Input 2"=w1003, "Input 2"=w1006) -> (w1000:T24)  [unwired: 1 in]
                n356 = To Variant(anything=w1000) -> (Variant=w1009:variant)
                n357 = call <vilib>:"DB Tools Insert Data.vi"("data"=w1009, "error in (no error)"=w1012, "columns"=string[] ["DATE", "SHIFT", "ST5_SCREW1_DATA", "ST5_SCREW1_STATUS", "ST5_SCREW2_DATA", "ST5_SCREW2_STATUS", "ST5_SCREW3_DATA", "ST5_FINAL_RST"], "table"="ST5_REPORT", "connection reference"=w1013) -> ("error out"=w1010:errorcluster, "connection reference out"=w1011:T13)  [unwired: 5 in]
              }
            }
            n358 = Bundle By Name(cluster=w945, "OP - 50.Screw 1 Data"=w939, "OP - 50.Screw 2 data"=w938, "OP - 50.Screw 3 Data"=w928) -> (w944:T11)
            n359 = call <vilib>:"Simple Error Handler.vi"("type of dialog (OK msg:1)"=w953, "error in (no error)"=w954) -> ("error out"=w952:errorcluster)  [unwired: 3 in, 4 out]
            n360 = call <vilib>:"Clear Errors.vi"("error in (no error)"=w952) -> ("error out"=w950:errorcluster)  [unwired: 5 in, 1 out]
            n361 = property on="OP - 50" class="Clust"(error in=w950) -> (error out=w947:errorcluster, "Controls[]"=w949:refnum<vi>[])  [unwired: 1 in, 1 out]
            n362 = for {
              tunnel: w931 -> [w964] mode=indexing
              tunnel: [w963] -> w930 mode=indexing if=w961
              i -> [w962]
              n363 = case shown="\"NG\"" w964 {
                tunnel: [2 ("CYCLE STATUS OK, NOK, ABORTED") 1 ("CYCLE STATUS OK, NOK, ABORTED") 0 ("CYCLE STATUS OK, NOK, ABORTED")] -> w963
                frame "NG" {
                }
                frame "OK" {
                }
                frame "-1", Default {
                }
              }
              n364 = Not Equal To 0?(x=w962) -> (x != 0?=w961:bool)
            }
            n365 = Index Array(array=w949, index #1=3 ("index"), index #2=4 ("index"), index #3=6 ("index")) -> (element #1=w934:refnum<vi>, element #2=w933:refnum<vi>, element #3=w926:refnum<vi>)
            n366 = Build Array(w934, w933, w926) -> (w932:refnum<vi>[])
            n367 = for {
              tunnel: w932 -> [w973] mode=indexing
              shift-right: [w969] -> w946
              shift-left: w947 -> [w971]
              tunnel: w930 -> [w968] mode=indexing
              w972 = refnum<vi> refnum  # Boolean
              n368 = To More Specific Class(target class=w972, reference=w973, error in=w971) -> (specific class reference=w974:refnum<vi>, error out=w970:errorcluster)
              n369 = call "PADMINI_BOOL_COLOR_CHANGE.vi"("error in (no error)"=w970, "Numeric"=w968, "Boolean in"=w974) -> ("error out"=w969:errorcluster)  [unwired: 8 in]
            }
          }
          frame "SCAN6" {
            # "STATION OP 60"
            n370 = case shown="True" w1022 {
              tunnel: w1026 -> [w1050 w1087]
              tunnel: w1025 -> [w1042 w1086]
              tunnel: w1024 -> [_ _]
              tunnel: [w1045 w1085] -> w1021
              tunnel: [w1043 w1087] -> w1023
              tunnel: [w1027 "" ("trimmed string")] -> w1014
              frame False {
                n371 = call "PADMINI_AUTO_BARCODE_STRING 60.vi"("Enum"=enum16{"Read", "Write"}."Read", "error in (no error)"=w1042) -> ("error out"=w1041:errorcluster, "Input 2"=w1029:string[])  [unwired: 8 in]
                n372 = global read "Global 1.vi" "BARCODE RECIPE"() -> (w1030:string)
                n373 = Index Array(array=w1029) -> (element=w1028:string)  [unwired: 1 in]
                n374 = call <vilib>:"Trim Whitespace.vi"("string"=w1028) -> ("trimmed string"=w1027:string)  [unwired: 1 in]
                n375 = Match Pattern(string=w1027, regular expression=w1030) -> (match substring=w1031:string)  [unwired: 1 in, 3 out]
                n376 = String Length(string=w1030) -> (length=w1033:i32)
                n377 = String Length(string=w1031) -> (length=w1032:i32)
                n378 = Format Into String(format string="WHERE BARCODE  ='%s'", w1027) -> (resulting string=w1037:string)  [unwired: 2 in, 1 out]
                n379 = Equal?(x=w1033, y=w1032) -> (x = y?=w1034:bool)
                n380 = call <vilib>:"DB Tools Select Data.vi"("condition"=w1037, "error in (no error)"=w1041, "columns"=string[] ["BARCODE", "ST5_FINAL_RST", "ST6_FINAL_RST"], "table"="REPORT", "connection reference"=w1050) -> ("error out"=w1048:errorcluster, "data"=w1047:variant[][], "connection reference out"=w1043:T13)  [unwired: 1 in]
                n381 = call "PADMINI_varient_to_data.vi"("error in (no error)"=w1048, "data"=w1047) -> ("error out"=w1046:errorcluster, "Array"=w1044:string[][])  [unwired: 8 in]
                n382 = Equal?(x=w1027, y="") -> (x = y?=w1035:bool)
                n383 = case shown="False" w1035 {
                  tunnel: w1046 -> [w1054 w1081]
                  tunnel: [w1053 w1080] -> w1045
                  tunnel: w1044 -> [w1052 _]
                  tunnel: w1034 -> [w1051 _]
                  frame False {
                    n384 = case shown="True" w1051 {
                      tunnel: w1054 -> [w1058 w1070]
                      tunnel: [w1057 w1069] -> w1053
                      tunnel: w1052 -> [_ w1077]
                      frame False {
                        w1055 = i32[] [0, 0, 0, 0, 0]  # I/P
                        n385 = call "PADMINI_AUTO_BARCODE_STATUS 60.vi"("Enum"=enum16{"Read", "Write"}."Write", "error in (no error)"=w1058, "I/P"=w1055) -> ("error out"=w1057:errorcluster)  [unwired: 7 in, 1 out]
                      }
                      frame True {
                        n386 = Index Array(array=w1077, index (row) #1=0 ("index (row)"), index (col) #1=1 ("disabled index (col)"), index (row) #2=0 ("index (row)"), index (col) #2=2 ("disabled index (col)")) -> (element #1=w1071:string)  [unwired: 1 out]
                        n387 = Empty String/Path?(string/path=w1071) -> (empty?=w1060:bool)
                        n388 = Equal?(x=w1071, y="OK") -> (x = y?=w1063:bool)
                        n389 = Boolean To (0,1)(Boolean=w1060) -> (0, 1=w1059:i16)
                        n390 = Not(x=w1063) -> (.not. x?=w1062:bool)
                        n391 = Boolean To (0,1)(Boolean=w1063) -> (0, 1=w1064:i16)
                        n392 = Boolean To (0,1)(Boolean=w1062) -> (0, 1=w1061:i16)
                        n393 = Build Array(1, 0, w1059, w1064, w1061) -> (w1068:i32[])
                        n394 = call "PADMINI_AUTO_BARCODE_STATUS 60.vi"("Enum"=enum16{"Read", "Write"}."Write", "error in (no error)"=w1070, "I/P"=w1068) -> ("error out"=w1069:errorcluster)  [unwired: 7 in, 1 out]
                      }
                    }
                  }
                  frame True {
                    w1078 = i32[] [0, 0, 0, 0, 0]  # I/P
                    n395 = call "PADMINI_AUTO_BARCODE_STATUS 60.vi"("Enum"=enum16{"Read", "Write"}."Write", "error in (no error)"=w1081, "I/P"=w1078) -> ("error out"=w1080:errorcluster)  [unwired: 7 in, 1 out]
                  }
                }
              }
              frame True {
                w1082 = i32[] [0, 0, 0, 0, 0]  # I/P
                n396 = call "PADMINI_AUTO_BARCODE_STATUS 60.vi"("Enum"=enum16{"Read", "Write"}."Write", "error in (no error)"=w1086, "I/P"=w1082) -> ("error out"=w1085:errorcluster)  [unwired: 7 in, 1 out]
              }
            }
            n397 = flat-sequence {
              tunnel: [w1089] -> w1020
              tunnel: w1021 -> [w1089]
              frame #0 {
                # "UPDATE op 60 SCAN sTATUS"
                n398 = global write "DATA LOG.vi" "OP 60 Outputs"(TRUE) -> ()
              }
            }
            n399 = Bundle By Name(cluster=w1016, "OP - 60.BARCODE"=w1014) -> (w1015:T11)
          }
          frame "DATALOG6" {
            w1128 = T14 2 items=["no dialog", "OK message", "continue or stop message", "OK message + warnings", "continue/stop + warnings"] ("type of dialog (OK msg:1)")
            # "datalog of OP 60"
            n400 = call "PADMINI_AUTO_BARCODE_STRING 60.vi"("Enum"=enum16{"Read", "Write"}."Read", "error in (no error)"=w1115) -> ("error out"=w1117:errorcluster, "Input 2"=w1106:string[])  [unwired: 8 in]
            n401 = call "PADMINI_AUTO_CYCLE VALUE 60.vi"("Enum"=enum16{"Read", "Write"}."Read", "error in (no error)"=w1115) -> ("Input 2"=w1111:dbl[])  [unwired: 8 in, 1 out]
            n402 = Index Array(array=w1111) -> (element #1=w1114:dbl, element #2=w1113:dbl, element #3=w1103:dbl, element #4=w1100:dbl, element #5=w1099:dbl, element #6=w1098:dbl)  [unwired: 6 in]
            n403 = Number To Fractional String(number=w1111, precision (6)=i16 2) -> (F-format string=w1110:string[])  [unwired: 2 in]
            n404 = case shown="False" w1133 {
              tunnel: w1134 -> [w1172 w1200]
              tunnel: w1117 -> [w1173 w1199]
              tunnel: [w1176 w1198] -> w1131
              tunnel: [w1175 w1197] -> w1129
              tunnel: w1132 -> [w1171 _]
              tunnel: w1110 -> [w1167 w1180]
              tunnel: w1106 -> [w1162 w1179]
              frame False {
                # "DO TRACEBILITY"
                n405 = Index Array(array=w1162) -> (element #1=w1163:string, element #2=w1159:string, element #3=w1158:string, element #4=w1157:string, element #5=w1155:string, element #6=w1152:string, element #7=w1151:string)  [unwired: 7 in]
                n406 = local read "SHIFT"() -> (w1174:string)
                n407 = Index Array(array=w1167) -> (element #1=w1166:string, element #2=w1161:string, element #3=w1160:string, element #4=w1156:string, element #5=w1154:string, element #6=w1153:string)  [unwired: 6 in]
                n408 = call <vilib>:"Trim Whitespace.vi"("string"=w1163) -> ("trimmed string"=w1164:string)  [unwired: 1 in]
                n409 = call "PADMINI_SHIFT_DATE.vi"("SHIFT"=w1174) -> ("date/time string"=w1150:string)  [unwired: 10 in]
                n410 = Format Into String(format string="Where BARCODE='%s' ", w1164) -> (resulting string=w1169:string)  [unwired: 2 in, 1 out]
                n411 = Bundle("date/time string"=w1150, "Input 2"=w1166, "Input 2"=w1159, "Input 2"=w1161, "Input 2"=w1158, "Input 2"=w1160, "Input 2"=w1157, "Input 2"=w1156, "Input 2"=w1155, "Input 2"=w1154, "Input 2"=w1153, "Input 2"=w1152, "Input 2"=w1151) -> (w1165:T25)  [unwired: 1 in]
                n412 = call <vilib>:"DB Tools Update Data.vi"("condition"=w1169, "data"=w1165, "error in (no error)"=w1173, "columns"=string[] ["DATEST6", "ST6_SCREW1_DATA", "ST6_SCREW1_STATUS", "ST6_SCREW2_DATA", "ST6_SCREW2_STATUS", "ST6_SCREW3_DATA", "ST6_SCREW3_STATUS", "ST6_SCREW4_DATA", "ST6_SCREW4_STATUS", "ST6_SCREW5_DATA", "ST6_SCREW5_STATUS", "ST6_SCREW6_DATA", "ST6_SCREW6_STATUS", "ST6_FINAL_RST"], "table"=w1171, "connection reference"=w1172) -> ("error out"=w1175:errorcluster, "connection reference out"=w1176:T13)  [unwired: 4 in]
              }
              frame True {
                # "TRAC BYPASS"
                n413 = local read "SHIFT"() -> (w1177:string)
                n414 = call "PADMINI_SHIFT_DATE.vi"("SHIFT"=w1177) -> ("date/time string"=w1178:string)  [unwired: 10 in]
                n415 = Index Array(array=w1179) -> (element #2=w1188:string, element #3=w1187:string, element #4=w1186:string, element #5=w1184:string, element #6=w1192:string, element #7=w1193:string)  [unwired: 7 in, 1 out]
                n416 = Index Array(array=w1180) -> (element #1=w1191:string, element #2=w1190:string, element #3=w1189:string, element #4=w1185:string, element #5=w1183:string, element #6=w1182:string)  [unwired: 6 in]
                n417 = Bundle("date/time string"=w1178, "SHIFT"=w1177, "Input 2"=w1191, "Input 2"=w1188, "Input 2"=w1190, "Input 2"=w1187, "Input 2"=w1189, "Input 2"=w1186, "Input 2"=w1185, "Input 2"=w1184, "Input 2"=w1183, "Input 2"=w1182, "Input 2"=w1192, "Input 2"=w1193) -> (w1181:T26)  [unwired: 1 in]
                n418 = To Variant(anything=w1181) -> (Variant=w1196:variant)
                n419 = call <vilib>:"DB Tools Insert Data.vi"("data"=w1196, "error in (no error)"=w1199, "columns"=string[] ["DATE", "SHIFT", "ST6_SCREW1_DATA", "ST6_SCREW1_STATUS", "ST6_SCREW2_DATA", "ST6_SCREW2_STATUS", "ST6_SCREW3_DATA", "ST6_SCREW3_STATUS", "ST6_SCREW4_DATA", "ST6_SCREW4_STATUS", "ST6_SCREW5_DATA", "ST6_SCREW5_STATUS", "ST6_SCREW6_DATA", "ST6_SCREW6_STATUS", "ST6_FINAL_RST"], "table"="ST6_REPORT", "connection reference"=w1200) -> ("error out"=w1197:errorcluster, "connection reference out"=w1198:T13)  [unwired: 5 in]
              }
            }
            n420 = Bundle By Name(cluster=w1120, "OP - 60.Screw 1 Data"=w1114, "OP - 60.Screw 2 data"=w1113, "OP - 60.Screw3 Data"=w1103, "OP - 60.Screw4 Data"=w1100, "OP - 60.Screw5 Data"=w1099, "OP - 60.Screw6 Data"=w1098) -> (w1119:T11)
            n421 = call <vilib>:"Simple Error Handler.vi"("type of dialog (OK msg:1)"=w1128, "error in (no error)"=w1129) -> ("error out"=w1127:errorcluster)  [unwired: 3 in, 4 out]
            n422 = call <vilib>:"Clear Errors.vi"("error in (no error)"=w1127) -> ("error out"=w1125:errorcluster)  [unwired: 5 in, 1 out]
            n423 = property on="OP - 60" class="Clust"(error in=w1125) -> (error out=w1122:errorcluster, "Controls[]"=w1124:refnum<vi>[])  [unwired: 1 in, 1 out]
            n424 = for {
              tunnel: w1106 -> [w1139] mode=indexing
              tunnel: [w1138] -> w1105 mode=indexing if=w1136
              i -> [w1137]
              n425 = case shown="\"NG\"" w1139 {
                tunnel: [2 ("CYCLE STATUS OK, NOK, ABORTED") 1 ("CYCLE STATUS OK, NOK, ABORTED") 0 ("CYCLE STATUS OK, NOK, ABORTED")] -> w1138
                frame "NG" {
                }
                frame "OK" {
                }
                frame "-1", Default {
                }
              }
              n426 = Not Equal To 0?(x=w1137) -> (x != 0?=w1136:bool)
            }
            n427 = Index Array(array=w1124, index #1=3 ("index"), index #2=4 ("index"), index #3=7 ("index"), index #4=10 ("index"), index #5=11 ("index"), index #6=13 ("index"), index #7=6 ("index")) -> (element #1=w1109:refnum<vi>, element #2=w1108:refnum<vi>, element #3=w1101:refnum<vi>, element #4=w1094:refnum<vi>, element #5=w1093:refnum<vi>, element #6=w1092:refnum<vi>, element #7=w1090:refnum<vi>)
            n428 = Build Array(w1109, w1108, w1101, w1094, w1093, w1092, w1090) -> (w1107:refnum<vi>[])
            n429 = for {
              tunnel: w1107 -> [w1148] mode=indexing
              shift-right: [w1144] -> w1121
              shift-left: w1122 -> [w1146]
              tunnel: w1105 -> [w1143] mode=indexing
              w1147 = refnum<vi> refnum  # Boolean
              n430 = To More Specific Class(target class=w1147, reference=w1148, error in=w1146) -> (specific class reference=w1149:refnum<vi>, error out=w1145:errorcluster)
              n431 = call "PADMINI_BOOL_COLOR_CHANGE.vi"("error in (no error)"=w1145, "Numeric"=w1143, "Boolean in"=w1149) -> ("error out"=w1144:errorcluster)  [unwired: 8 in]
            }
          }
          frame "SCAN7" {
            # "STATION OP 70"
            n432 = case shown="False" w1209 {
              tunnel: w1213 -> [w1237 w1274]
              tunnel: w1212 -> [w1229 w1273]
              tunnel: w1211 -> [w1214 _]
              tunnel: [w1232 w1272] -> w1208
              tunnel: [w1230 w1274] -> w1210
              tunnel: [w1215 "" ("trimmed string")] -> w1201
              frame False {
                (unwired) "REPORT"
                n433 = call "PADMINI_AUTO_BARCODE_STRING 70.vi"("Enum"=enum16{"Read", "Write"}."Read", "error in (no error)"=w1229) -> ("error out"=w1228:errorcluster, "Input 2"=w1217:string[])  [unwired: 8 in]
                n434 = global read "Global 1.vi" "BARCODE RECIPE"() -> (w1218:string)
                n435 = Index Array(array=w1217) -> (element=w1216:string)  [unwired: 1 in]
                n436 = call <vilib>:"Trim Whitespace.vi"("string"=w1216) -> ("trimmed string"=w1215:string)  [unwired: 1 in]
                n437 = Match Pattern(string=w1215, regular expression=w1218) -> (match substring=w1219:string)  [unwired: 1 in, 3 out]
                n438 = String Length(string=w1218) -> (length=w1221:i32)
                n439 = String Length(string=w1219) -> (length=w1220:i32)
                n440 = Format Into String(format string="WHERE BARCODE  ='%s'", w1215) -> (resulting string=w1225:string)  [unwired: 2 in, 1 out]
                n441 = Equal?(x=w1221, y=w1220) -> (x = y?=w1222:bool)
                n442 = call <vilib>:"DB Tools Select Data.vi"("condition"=w1225, "error in (no error)"=w1228, "columns"=string[] ["BARCODE", "ST6_FINAL_RST", "ST7_FINAL_RST"], "table"=w1214, "connection reference"=w1237) -> ("error out"=w1235:errorcluster, "data"=w1234:variant[][], "connection reference out"=w1230:T13)  [unwired: 1 in]
                n443 = call "PADMINI_varient_to_data.vi"("error in (no error)"=w1235, "data"=w1234) -> ("error out"=w1233:errorcluster, "Array"=w1231:string[][])  [unwired: 8 in]
                n444 = Equal?(x=w1215, y="") -> (x = y?=w1223:bool)
                n445 = case shown="False" w1223 {
                  tunnel: w1233 -> [w1241 w1268]
                  tunnel: [w1240 w1267] -> w1232
                  tunnel: w1231 -> [w1239 _]
                  tunnel: w1222 -> [w1238 _]
                  frame False {
                    n446 = case shown="True" w1238 {
                      tunnel: w1241 -> [w1245 w1257]
                      tunnel: [w1244 w1256] -> w1240
                      tunnel: w1239 -> [_ w1264]
                      frame False {
                        w1242 = i32[] [0, 0, 0, 0, 0]  # I/P
                        n447 = call "PADMINI_AUTO_BARCODE_STATUS 70.vi"("Enum"=enum16{"Read", "Write"}."Write", "error in (no error)"=w1245, "I/P"=w1242) -> ("error out"=w1244:errorcluster)  [unwired: 7 in, 1 out]
                      }
                      frame True {
                        n448 = Index Array(array=w1264, index (row) #1=0 ("index (row)"), index (col) #1=1 ("disabled index (col)"), index (row) #2=0 ("index (row)"), index (col) #2=2 ("disabled index (col)")) -> (element #1=w1258:string)  [unwired: 1 out]
                        n449 = Empty String/Path?(string/path=w1258) -> (empty?=w1251:bool)
                        n450 = Equal?(x=w1258, y="OK") -> (x = y?=w1246:bool)
                        n451 = Boolean To (0,1)(Boolean=w1251) -> (0, 1=w1250:i16)
                        n452 = Not(x=w1246) -> (.not. x?=w1249:bool)
                        n453 = Boolean To (0,1)(Boolean=w1246) -> (0, 1=w1247:i16)
                        n454 = Boolean To (0,1)(Boolean=w1249) -> (0, 1=w1248:i16)
                        n455 = Build Array(1, 0, w1250, w1247, w1248) -> (w1255:i32[])
                        n456 = call "PADMINI_AUTO_BARCODE_STATUS 70.vi"("Enum"=enum16{"Read", "Write"}."Write", "error in (no error)"=w1257, "I/P"=w1255) -> ("error out"=w1256:errorcluster)  [unwired: 7 in, 1 out]
                      }
                    }
                  }
                  frame True {
                    w1265 = i32[] [0, 0, 0, 0, 0]  # I/P
                    n457 = call "PADMINI_AUTO_BARCODE_STATUS 70.vi"("Enum"=enum16{"Read", "Write"}."Write", "error in (no error)"=w1268, "I/P"=w1265) -> ("error out"=w1267:errorcluster)  [unwired: 7 in, 1 out]
                  }
                }
              }
              frame True {
                w1269 = i32[] [0, 0, 0, 0, 0]  # I/P
                n458 = call "PADMINI_AUTO_BARCODE_STATUS 70.vi"("Enum"=enum16{"Read", "Write"}."Write", "error in (no error)"=w1273, "I/P"=w1269) -> ("error out"=w1272:errorcluster)  [unwired: 7 in, 1 out]
              }
            }
            n459 = flat-sequence {
              tunnel: [w1276] -> w1207
              tunnel: w1208 -> [w1276]
              frame #0 {
                # "UPDATE op 70 SCAN sTATUS"
                n460 = global write "DATA LOG.vi" "OP 70 Outputs"(TRUE) -> ()
              }
            }
            n461 = Bundle By Name(cluster=w1203, "OP - 70.BARCODE"=w1201) -> (w1202:T11)
          }
          frame "DATALOG7" {
            w1299 = T14 2 items=["no dialog", "OK message", "continue or stop message", "OK message + warnings", "continue/stop + warnings"] ("type of dialog (OK msg:1)")
            # "datalog of OP 70"
            n462 = call "PADMINI_AUTO_BARCODE_STRING 70.vi"("Enum"=enum16{"Read", "Write"}."Read", "error in (no error)"=w1286) -> ("error out"=w1288:errorcluster, "Input 2"=w1278:string[])  [unwired: 8 in]
            n463 = call "PADMINI_AUTO_CYCLE VALUE 70.vi"("Enum"=enum16{"Read", "Write"}."Read", "error in (no error)"=w1286) -> ("Input 2"=w1282:dbl[])  [unwired: 8 in, 1 out]
            n464 = Index Array(array=w1282) -> (element #1=w1285:dbl, element #2=w1284:dbl)  [unwired: 2 in]
            n465 = Number To Fractional String(number=w1282, precision (6)=i16 2) -> (F-format string=w1281:string[])  [unwired: 2 in]
            n466 = case shown="True" w1304 {
              tunnel: w1305 -> [w1335 w1353]
              tunnel: w1288 -> [w1336 w1352]
              tunnel: [w1338 w1351] -> w1302
              tunnel: [w1337 w1350] -> w1300
              tunnel: w1303 -> [w1334 _]
              tunnel: w1281 -> [w1330 w1340]
              tunnel: w1278 -> [w1325 w1339]
              frame False {
                # "DO TRACEBILITY"
                n467 = Index Array(array=w1325) -> (element #1=w1326:string, element #2=w1324:string)  [unwired: 2 in]
                n468 = call <vilib>:"Trim Whitespace.vi"("string"=w1326) -> ("trimmed string"=w1327:string)  [unwired: 1 in]
                n469 = local read "SHIFT"() -> (w1322:string)
                n470 = Index Array(array=w1330) -> (element #1=w1329:string, element #2=w1323:string)  [unwired: 2 in]
                n471 = call "PADMINI_SHIFT_DATE.vi"("SHIFT"=w1322) -> ("date/time string"=w1321:string)  [unwired: 10 in]
                n472 = Bundle("date/time string"=w1321, "Input 2"=w1329, "Input 2"=w1323, "Input 2"=w1324) -> (w1328:T27)  [unwired: 1 in]
                n473 = Format Into String(format string="Where BARCODE='%s' ", w1327) -> (resulting string=w1332:string)  [unwired: 2 in, 1 out]
                n474 = call <vilib>:"DB Tools Update Data.vi"("condition"=w1332, "data"=w1328, "error in (no error)"=w1336, "columns"=string[] ["DATEST7", "ST7_SENSOR_MIN_VLTG", "ST7_SENSOR_MAX_VLTG", "ST7_FINAL_RST"], "table"=w1334, "connection reference"=w1335) -> ("error out"=w1337:errorcluster, "connection reference out"=w1338:T13)  [unwired: 4 in]
              }
              frame True {
                # "TRAC BYPASS"
                n475 = local read "SHIFT"() -> (w1341:string)
                n476 = call "PADMINI_SHIFT_DATE.vi"("SHIFT"=w1341) -> ("date/time string"=w1342:string)  [unwired: 10 in]
                n477 = Index Array(array=w1339) -> (element #2=w1345:string)  [unwired: 2 in, 1 out]
                n478 = Index Array(array=w1340) -> (element #1=w1346:string, element #2=w1344:string)  [unwired: 2 in]
                n479 = Bundle("date/time string"=w1342, "SHIFT"=w1341, "Input 2"=w1346, "Input 2"=w1344, "Input 2"=w1345) -> (w1343:T28)  [unwired: 1 in]
                n480 = To Variant(anything=w1343) -> (Variant=w1349:variant)
                n481 = call <vilib>:"DB Tools Insert Data.vi"("data"=w1349, "error in (no error)"=w1352, "columns"=string[] ["DATE", "SHIFT", "ST7_SENSOR_MIN_VLTG", "ST7_SENSOR_MAX_VLTG", "ST7_FINAL_RST"], "table"="ST7_REPORT", "connection reference"=w1353) -> ("error out"=w1350:errorcluster, "connection reference out"=w1351:T13)  [unwired: 5 in]
              }
            }
            n482 = Bundle By Name(cluster=w1291, "OP - 70.Sensor MIN Vltg"=w1285, "OP - 70.Sensor MAX Vltg"=w1284) -> (w1290:T11)
            n483 = call <vilib>:"Simple Error Handler.vi"("type of dialog (OK msg:1)"=w1299, "error in (no error)"=w1300) -> ("error out"=w1298:errorcluster)  [unwired: 3 in, 4 out]
            n484 = call <vilib>:"Clear Errors.vi"("error in (no error)"=w1298) -> ("error out"=w1296:errorcluster)  [unwired: 5 in, 1 out]
            n485 = property on="OP - 70" class="Clust"(error in=w1296) -> (error out=w1293:errorcluster, "Controls[]"=w1295:refnum<vi>[])  [unwired: 1 in, 1 out]
            n486 = for {
              tunnel: w1278 -> [w1310] mode=indexing
              tunnel: [w1309] -> w1277 mode=indexing if=w1307
              i -> [w1308]
              n487 = case shown="\"NG\"" w1310 {
                tunnel: [2 ("CYCLE STATUS OK, NOK, ABORTED") 1 ("CYCLE STATUS OK, NOK, ABORTED") 0 ("CYCLE STATUS OK, NOK, ABORTED")] -> w1309
                frame "NG" {
                }
                frame "OK" {
                }
                frame "-1", Default {
                }
              }
              n488 = Not Equal To 0?(x=w1308) -> (x != 0?=w1307:bool)
            }
            n489 = Index Array(array=w1295, index=3) -> (element=w1280:refnum<vi>)
            n490 = Build Array(w1280) -> (w1279:refnum<vi>[])
            n491 = for {
              tunnel: w1279 -> [w1319] mode=indexing
              shift-right: [w1315] -> w1292
              shift-left: w1293 -> [w1317]
              tunnel: w1277 -> [w1314] mode=indexing
              w1318 = refnum<vi> refnum  # Boolean
              n492 = To More Specific Class(target class=w1318, reference=w1319, error in=w1317) -> (specific class reference=w1320:refnum<vi>, error out=w1316:errorcluster)
              n493 = call "PADMINI_BOOL_COLOR_CHANGE.vi"("error in (no error)"=w1316, "Numeric"=w1314, "Boolean in"=w1320) -> ("error out"=w1315:errorcluster)  [unwired: 8 in]
            }
          }
          frame "SCAN8" {
            # "STATION OP 80"
            n494 = case shown="False" w1362 {
              tunnel: w1366 -> [w1390 w1429]
              tunnel: w1365 -> [w1382 w1428]
              tunnel: w1364 -> [w1367 _]
              tunnel: [w1385 w1427] -> w1361
              tunnel: [w1383 w1429] -> w1363
              tunnel: [w1368 "" ("trimmed string")] -> w1354
              frame False {
                (unwired) "REPORT"
                n495 = call "PADMINI_AUTO_BARCODE_STRING 80.vi"("Enum"=enum16{"Read", "Write"}."Read", "error in (no error)"=w1382) -> ("error out"=w1381:errorcluster, "Input 2"=w1370:string[])  [unwired: 8 in]
                n496 = global read "Global 1.vi" "BARCODE RECIPE"() -> (w1371:string)
                n497 = Index Array(array=w1370) -> (element=w1369:string)  [unwired: 1 in]
                n498 = call <vilib>:"Trim Whitespace.vi"("string"=w1369) -> ("trimmed string"=w1368:string)  [unwired: 1 in]
                n499 = Match Pattern(string=w1368, regular expression=w1371) -> (match substring=w1372:string)  [unwired: 1 in, 3 out]
                n500 = String Length(string=w1371) -> (length=w1374:i32)
                n501 = String Length(string=w1372) -> (length=w1373:i32)
                n502 = Format Into String(format string="WHERE BARCODE  ='%s'", w1368) -> (resulting string=w1378:string)  [unwired: 2 in, 1 out]
                n503 = Equal?(x=w1374, y=w1373) -> (x = y?=w1375:bool)
                n504 = call <vilib>:"DB Tools Select Data.vi"("condition"=w1378, "error in (no error)"=w1381, "columns"=string[] ["BARCODE", "ST7_FINAL_RST", "ST8_FINAL_RST"], "table"=w1367, "connection reference"=w1390) -> ("error out"=w1388:errorcluster, "data"=w1387:variant[][], "connection reference out"=w1383:T13)  [unwired: 1 in]
                n505 = call "PADMINI_varient_to_data.vi"("error in (no error)"=w1388, "data"=w1387) -> ("error out"=w1386:errorcluster, "Array"=w1384:string[][])  [unwired: 8 in]
                n506 = Equal?(x=w1368, y="") -> (x = y?=w1376:bool)
                n507 = case shown="True" w1376 {
                  tunnel: w1386 -> [w1394 w1423]
                  tunnel: [w1393 w1422] -> w1385
                  tunnel: w1384 -> [w1392 _]
                  tunnel: w1375 -> [w1391 _]
                  frame False {
                    n508 = case shown="True" w1391 {
                      tunnel: w1394 -> [w1398 w1407]
                      tunnel: [w1397 w1406] -> w1393
                      tunnel: w1392 -> [_ w1419]
                      frame False {
                        w1395 = i32[] [0, 0, 0, 0, 0]  # I/P
                        n509 = call "PADMINI_AUTO_BARCODE_STATUS 80.vi"("Enum"=enum16{"Read", "Write"}."Write", "error in (no error)"=w1398, "I/P"=w1395) -> ("error out"=w1397:errorcluster)  [unwired: 7 in, 1 out]
                      }
                      frame True {
                        n510 = Index Array(array=w1419, index (row) #1=0 ("index (row)"), index (col) #1=1 ("disabled index (col)"), index (row) #2=0 ("index (row)"), index (col) #2=2 ("disabled index (col)")) -> (element #1=w1413:string)  [unwired: 1 out]
                        n511 = Empty String/Path?(string/path=w1413) -> (empty?=w1411:bool)
                        n512 = Equal?(x=w1413, y="OK") -> (x = y?=w1409:bool)
                        n513 = Not(x=w1409) -> (.not. x?=w1408:bool)
                        n514 = Boolean To (0,1)(Boolean=TRUE ("element")) -> (0, 1=w1404:i16)
                        n515 = Boolean To (0,1)(Boolean=FALSE ("element")) -> (0, 1=w1403:i16)
                        n516 = Boolean To (0,1)(Boolean=w1411) -> (0, 1=w1402:i16)
                        n517 = Boolean To (0,1)(Boolean=w1409) -> (0, 1=w1401:i16)
                        n518 = Boolean To (0,1)(Boolean=w1408) -> (0, 1=w1400:i16)
                        n519 = Build Array(w1404, w1403, w1402, w1401, w1400) -> (w1399:i16[])
                        n520 = call "PADMINI_AUTO_BARCODE_STATUS 80.vi"("Enum"=enum16{"Read", "Write"}."Write", "error in (no error)"=w1407, "I/P"=w1399) -> ("error out"=w1406:errorcluster)  [unwired: 7 in, 1 out]
                      }
                    }
                  }
                  frame True {
                    w1420 = i32[] [0, 0, 0, 0, 0]  # I/P
                    n521 = call "PADMINI_AUTO_BARCODE_STATUS 80.vi"("Enum"=enum16{"Read", "Write"}."Write", "error in (no error)"=w1423, "I/P"=w1420) -> ("error out"=w1422:errorcluster)  [unwired: 7 in, 1 out]
                  }
                }
              }
              frame True {
                w1424 = i32[] [0, 0, 0, 0, 0]  # I/P
                n522 = call "PADMINI_AUTO_BARCODE_STATUS 80.vi"("Enum"=enum16{"Read", "Write"}."Write", "error in (no error)"=w1428, "I/P"=w1424) -> ("error out"=w1427:errorcluster)  [unwired: 7 in, 1 out]
              }
            }
            n523 = flat-sequence {
              tunnel: [w1431] -> w1360
              tunnel: w1361 -> [w1431]
              frame #0 {
                # "UPDATE op 80 SCAN sTATUS"
                n524 = global write "DATA LOG.vi" "OP 80 Outputs"(TRUE) -> ()
              }
            }
            n525 = Bundle By Name(cluster=w1356, "OP - 80.BARCODE"=w1354) -> (w1355:T11)
          }
          frame "DATALOG8" {
            w1455 = T14 2 items=["no dialog", "OK message", "continue or stop message", "OK message + warnings", "continue/stop + warnings"] ("type of dialog (OK msg:1)")
            # "datalog of OP 80"
            n526 = call "PADMINI_AUTO_BARCODE_STRING 80.vi"("Enum"=enum16{"Read", "Write"}."Read", "error in (no error)"=w1442) -> ("error out"=w1444:errorcluster, "Input 2"=w1435:string[])  [unwired: 8 in]
            n527 = call "PADMINI_AUTO_CYCLE VALUE 80.vi"("Enum"=enum16{"Read", "Write"}."Read", "error in (no error)"=w1442) -> ("Input 2"=w1439:dbl[])  [unwired: 8 in, 1 out]
            n528 = Index Array(array=w1439) -> (element=w1441:dbl)  [unwired: 1 in]
            n529 = Number To Fractional String(number=w1439, precision (6)=i16 2) -> (F-format string=w1438:string[])  [unwired: 2 in]
            n530 = case shown="False" w1460 {
              tunnel: w1461 -> [w1491 w1509]
              tunnel: w1444 -> [w1492 w1508]
              tunnel: [w1494 w1507] -> w1458
              tunnel: [w1493 w1506] -> w1456
              tunnel: w1459 -> [w1490 _]
              tunnel: w1438 -> [w1486 w1497]
              tunnel: w1435 -> [w1482 w1498]
              frame False {
                # "DO TRACEBILITY"
                n531 = Index Array(array=w1482) -> (element #1=w1483:string, element #2=w1481:string, element #3=w1480:string)  [unwired: 3 in]
                n532 = call <vilib>:"Trim Whitespace.vi"("string"=w1483) -> ("trimmed string"=w1484:string)  [unwired: 1 in]
                n533 = local read "SHIFT"() -> (w1478:string)
                n534 = Index Array(array=w1486) -> (element=w1479:string)  [unwired: 1 in]
                n535 = call "PADMINI_SHIFT_DATE.vi"("SHIFT"=w1478) -> ("date/time string"=w1477:string)  [unwired: 10 in]
                n536 = Bundle("date/time string"=w1477, "Input 2"=w1479, "Input 2"=w1481, "Input 2"=w1480) -> (w1485:T27)  [unwired: 1 in]
                n537 = Format Into String(format string="Where BARCODE='%s' ", w1484) -> (resulting string=w1488:string)  [unwired: 2 in, 1 out]
                n538 = call <vilib>:"DB Tools Update Data.vi"("condition"=w1488, "data"=w1485, "error in (no error)"=w1492, "columns"=string[] ["DATEST8", "ST8_DISPENSING", "ST8_LOAD", "ST8_FINAL_RST"], "table"=w1490, "connection reference"=w1491) -> ("error out"=w1493:errorcluster, "connection reference out"=w1494:T13)  [unwired: 4 in]
              }
              frame True {
                # "TRAC BYPASS"
                n539 = local read "SHIFT"() -> (w1495:string)
                n540 = call "PADMINI_SHIFT_DATE.vi"("SHIFT"=w1495) -> ("date/time string"=w1496:string)  [unwired: 10 in]
                n541 = Index Array(array=w1498) -> (element #2=w1502:string, element #3=w1501:string)  [unwired: 3 in, 1 out]
                n542 = Index Array(array=w1497) -> (element=w1500:string)  [unwired: 1 in]
                n543 = Bundle("date/time string"=w1496, "SHIFT"=w1495, "Input 2"=w1500, "Input 2"=w1502, "Input 2"=w1501) -> (w1499:T28)  [unwired: 1 in]
                n544 = To Variant(anything=w1499) -> (Variant=w1505:variant)
                n545 = call <vilib>:"DB Tools Insert Data.vi"("data"=w1505, "error in (no error)"=w1508, "columns"=string[] ["DATE", "SHIFT", "ST8_DISPENSING", "ST8_LOAD", "ST8_FINAL_RST"], "table"="ST8_REPORT", "connection reference"=w1509) -> ("error out"=w1506:errorcluster, "connection reference out"=w1507:T13)  [unwired: 5 in]
              }
            }
            n546 = Bundle By Name(cluster=w1447, "OP - 80.Load"=w1441) -> (w1446:T11)
            n547 = call <vilib>:"Simple Error Handler.vi"("type of dialog (OK msg:1)"=w1455, "error in (no error)"=w1456) -> ("error out"=w1454:errorcluster)  [unwired: 3 in, 4 out]
            n548 = call <vilib>:"Clear Errors.vi"("error in (no error)"=w1454) -> ("error out"=w1452:errorcluster)  [unwired: 5 in, 1 out]
            n549 = property on="OP - 80" class="Clust"(error in=w1452) -> (error out=w1449:errorcluster, "Controls[]"=w1451:refnum<vi>[])  [unwired: 1 in, 1 out]
            n550 = for {
              tunnel: w1435 -> [w1466] mode=indexing
              tunnel: [w1465] -> w1434 mode=indexing if=w1463
              i -> [w1464]
              n551 = case shown="\"NG\"" w1466 {
                tunnel: [2 ("CYCLE STATUS OK, NOK, ABORTED") 1 ("CYCLE STATUS OK, NOK, ABORTED") 0 ("CYCLE STATUS OK, NOK, ABORTED")] -> w1465
                frame "NG" {
                }
                frame "OK" {
                }
                frame "-1", Default {
                }
              }
              n552 = Not Equal To 0?(x=w1464) -> (x != 0?=w1463:bool)
            }
            n553 = Index Array(array=w1451, index #1=3 ("index"), index #2=2 ("index")) -> (element #1=w1437:refnum<vi>, element #2=w1432:refnum<vi>)
            n554 = Build Array(w1437, w1432) -> (w1436:refnum<vi>[])
            n555 = for {
              tunnel: w1436 -> [w1475] mode=indexing
              shift-right: [w1471] -> w1448
              shift-left: w1449 -> [w1473]
              tunnel: w1434 -> [w1470] mode=indexing
              w1474 = refnum<vi> refnum  # Boolean
              n556 = To More Specific Class(target class=w1474, reference=w1475, error in=w1473) -> (specific class reference=w1476:refnum<vi>, error out=w1472:errorcluster)
              n557 = call "PADMINI_BOOL_COLOR_CHANGE.vi"("error in (no error)"=w1472, "Numeric"=w1470, "Boolean in"=w1476) -> ("error out"=w1471:errorcluster)  [unwired: 8 in]
            }
          }
          frame "SCAN9" {
            # "STATION OP 90"
            n558 = case shown="False" w1518 {
              tunnel: w1522 -> [w1546 w1585]
              tunnel: w1521 -> [w1538 w1584]
              tunnel: w1520 -> [w1523 _]
              tunnel: [w1541 w1583] -> w1517
              tunnel: [w1539 w1585] -> w1519
              tunnel: [w1524 "" ("trimmed string")] -> w1510
              frame False {
                (unwired) "REPORT"
                n559 = call "PADMINI_AUTO_BARCODE_STRING 90.vi"("Enum"=enum16{"Read", "Write"}."Read", "error in (no error)"=w1538) -> ("error out"=w1537:errorcluster, "Input 2"=w1526:string[])  [unwired: 8 in]
                n560 = global read "Global 1.vi" "BARCODE RECIPE"() -> (w1527:string)
                n561 = Index Array(array=w1526) -> (element=w1525:string)  [unwired: 1 in]
                n562 = call <vilib>:"Trim Whitespace.vi"("string"=w1525) -> ("trimmed string"=w1524:string)  [unwired: 1 in]
                n563 = Match Pattern(string=w1524, regular expression=w1527) -> (match substring=w1528:string)  [unwired: 1 in, 3 out]
                n564 = String Length(string=w1527) -> (length=w1530:i32)
                n565 = String Length(string=w1528) -> (length=w1529:i32)
                n566 = Format Into String(format string="WHERE BARCODE  ='%s'", w1524) -> (resulting string=w1534:string)  [unwired: 2 in, 1 out]
                n567 = Equal?(x=w1530, y=w1529) -> (x = y?=w1531:bool)
                n568 = call <vilib>:"DB Tools Select Data.vi"("condition"=w1534, "error in (no error)"=w1537, "columns"=string[] ["BARCODE", "ST8_FINAL_RST", "ST9_FINAL_RST"], "table"=w1523, "connection reference"=w1546) -> ("error out"=w1544:errorcluster, "data"=w1543:variant[][], "connection reference out"=w1539:T13)  [unwired: 1 in]
                n569 = call "PADMINI_varient_to_data.vi"("error in (no error)"=w1544, "data"=w1543) -> ("error out"=w1542:errorcluster, "Array"=w1540:string[][])  [unwired: 8 in]
                n570 = Equal?(x=w1524, y="") -> (x = y?=w1532:bool)
                n571 = case shown="False" w1532 {
                  tunnel: w1542 -> [w1550 w1579]
                  tunnel: [w1549 w1578] -> w1541
                  tunnel: w1540 -> [w1548 _]
                  tunnel: w1531 -> [w1547 _]
                  frame False {
                    n572 = case shown="True" w1547 {
                      tunnel: w1550 -> [w1554 w1563]
                      tunnel: [w1553 w1562] -> w1549
                      tunnel: w1548 -> [_ w1575]
                      frame False {
                        w1551 = i32[] [0, 0, 0, 0, 0]  # I/P
                        n573 = call "PADMINI_AUTO_BARCODE_STATUS 90.vi"("Enum"=enum16{"Read", "Write"}."Write", "error in (no error)"=w1554, "I/P"=w1551) -> ("error out"=w1553:errorcluster)  [unwired: 7 in, 1 out]
                      }
                      frame True {
                        n574 = Index Array(array=w1575, index (row) #1=0 ("index (row)"), index (col) #1=1 ("disabled index (col)"), index (row) #2=0 ("index (row)"), index (col) #2=2 ("disabled index (col)")) -> (element #1=w1569:string)  [unwired: 1 out]
                        n575 = Empty String/Path?(string/path=w1569) -> (empty?=w1567:bool)
                        n576 = Equal?(x=w1569, y="OK") -> (x = y?=w1565:bool)
                        n577 = Boolean To (0,1)(Boolean=TRUE ("element")) -> (0, 1=w1559:i16)
                        n578 = Boolean To (0,1)(Boolean=FALSE ("element")) -> (0, 1=w1558:i16)
                        n579 = Not(x=w1565) -> (.not. x?=w1564:bool)
                        n580 = Boolean To (0,1)(Boolean=w1567) -> (0, 1=w1557:i16)
                        n581 = Boolean To (0,1)(Boolean=w1565) -> (0, 1=w1556:i16)
                        n582 = Boolean To (0,1)(Boolean=w1564) -> (0, 1=w1555:i16)
                        n583 = Build Array(w1559, w1558, w1557, w1556, w1555) -> (w1560:i16[])
                        n584 = call "PADMINI_AUTO_BARCODE_STATUS 90.vi"("Enum"=enum16{"Read", "Write"}."Write", "error in (no error)"=w1563, "I/P"=w1560) -> ("error out"=w1562:errorcluster)  [unwired: 7 in, 1 out]
                      }
                    }
                  }
                  frame True {
                    w1576 = i32[] [0, 0, 0, 0, 0]  # I/P
                    n585 = call "PADMINI_AUTO_BARCODE_STATUS 90.vi"("Enum"=enum16{"Read", "Write"}."Write", "error in (no error)"=w1579, "I/P"=w1576) -> ("error out"=w1578:errorcluster)  [unwired: 7 in, 1 out]
                  }
                }
              }
              frame True {
                w1580 = i32[] [0, 0, 0, 0, 0]  # I/P
                n586 = call "PADMINI_AUTO_BARCODE_STATUS 90.vi"("Enum"=enum16{"Read", "Write"}."Write", "error in (no error)"=w1584, "I/P"=w1580) -> ("error out"=w1583:errorcluster)  [unwired: 7 in, 1 out]
              }
            }
            n587 = flat-sequence {
              tunnel: [w1587] -> w1516
              tunnel: w1517 -> [w1587]
              frame #0 {
                # "UPDATE op 90 SCAN sTATUS"
                n588 = global write "DATA LOG.vi" "OP 90 Outputs"(TRUE) -> ()
              }
            }
            n589 = Bundle By Name(cluster=w1512, "OP - 90.BARCODE"=w1510) -> (w1511:T11)
          }
          frame "DATALOG9" {
            w1612 = T14 2 items=["no dialog", "OK message", "continue or stop message", "OK message + warnings", "continue/stop + warnings"] ("type of dialog (OK msg:1)")
            # "datalog of OP 90"
            n590 = call "PADMINI_AUTO_BARCODE_STRING 90.vi"("Enum"=enum16{"Read", "Write"}."Read", "error in (no error)"=w1599) -> ("error out"=w1601:errorcluster, "Input 2"=w1593:string[])  [unwired: 8 in]
            n591 = call "PADMINI_AUTO_CYCLE VALUE 90.vi"("Enum"=enum16{"Read", "Write"}."Read", "error in (no error)"=w1599) -> ("Input 2"=w1589:dbl[])  [unwired: 8 in, 1 out]
            n592 = Index Array(array=w1589) -> (element #1=w1598:dbl, element #2=w1588:dbl)  [unwired: 2 in]
            n593 = Number To Fractional String(number=w1589, precision (6)=i16 2) -> (F-format string=w1596:string[])  [unwired: 2 in]
            n594 = case shown="False" w1617 {
              tunnel: w1618 -> [w1649 w1668]
              tunnel: w1601 -> [w1650 w1667]
              tunnel: [w1652 w1666] -> w1615
              tunnel: [w1651 w1665] -> w1613
              tunnel: w1616 -> [w1648 _]
              tunnel: w1596 -> [w1644 w1657]
              tunnel: w1593 -> [w1640 w1656]
              frame False {
                # "DO TRACEBILITY"
                n595 = Index Array(array=w1640) -> (element #1=w1641:string, element #2=w1638:string, element #3=w1636:string)  [unwired: 3 in]
                n596 = call <vilib>:"Trim Whitespace.vi"("string"=w1641) -> ("trimmed string"=w1642:string)  [unwired: 1 in]
                n597 = local read "SHIFT"() -> (w1635:string)
                n598 = Index Array(array=w1644) -> (element #1=w1639:string, element #2=w1637:string)  [unwired: 2 in]
                n599 = call "PADMINI_SHIFT_DATE.vi"("SHIFT"=w1635) -> ("date/time string"=w1634:string)  [unwired: 10 in]
                n600 = Bundle("date/time string"=w1634, "Input 2"=w1639, "Input 2"=w1638, "Input 2"=w1637, "Input 2"=w1636) -> (w1643:T19)  [unwired: 1 in]
                n601 = Format Into String(format string="Where BARCODE='%s' ", w1642) -> (resulting string=w1646:string)  [unwired: 2 in, 1 out]
                n602 = call <vilib>:"DB Tools Update Data.vi"("condition"=w1646, "data"=w1643, "error in (no error)"=w1650, "columns"=string[] ["DATEST9", "ST9_SEAT_LT_DATA", "ST9_SEAT_STATUS", "ST9_STEAM_LT_DATA", "ST9_FINAL_RST"], "table"=w1648, "connection reference"=w1649) -> ("error out"=w1651:errorcluster, "connection reference out"=w1652:T13)  [unwired: 4 in]
              }
              frame True {
                # "TRAC BYPASS"
                n603 = local read "SHIFT"() -> (w1653:string)
                n604 = call "PADMINI_SHIFT_DATE.vi"("SHIFT"=w1653) -> ("date/time string"=w1654:string)  [unwired: 10 in]
                n605 = Index Array(array=w1656) -> (element #2=w1661:string, element #3=w1659:string)  [unwired: 3 in, 1 out]
                n606 = Index Array(array=w1657) -> (element #1=w1662:string, element #2=w1660:string)  [unwired: 2 in]
                n607 = Bundle("date/time string"=w1654, "SHIFT"=w1653, "Input 2"=w1662, "Input 2"=w1661, "Input 2"=w1660, "Input 2"=w1659) -> (w1658:T20)  [unwired: 1 in]
                n608 = To Variant(anything=w1658) -> (Variant=w1664:variant)
                n609 = call <vilib>:"DB Tools Insert Data.vi"("data"=w1664, "error in (no error)"=w1667, "columns"=string[] ["DATE", "SHIFT", "ST9_SEAT_LT_DATA", "ST9_SEAT_STATUS", "ST9_STEAM_LT_DATA", "ST9_FINAL_RST"], "table"="ST9_REPORT", "connection reference"=w1668) -> ("error out"=w1665:errorcluster, "connection reference out"=w1666:T13)  [unwired: 5 in]
              }
            }
            n610 = Bundle By Name(cluster=w1604, "OP - 90.Seat LT Data"=w1598, "OP - 90.Steam LT Data"=w1588) -> (w1603:T11)
            n611 = call <vilib>:"Simple Error Handler.vi"("type of dialog (OK msg:1)"=w1612, "error in (no error)"=w1613) -> ("error out"=w1611:errorcluster)  [unwired: 3 in, 4 out]
            n612 = call <vilib>:"Clear Errors.vi"("error in (no error)"=w1611) -> ("error out"=w1609:errorcluster)  [unwired: 5 in, 1 out]
            n613 = property on="OP - 90" class="Clust"(error in=w1609) -> (error out=w1606:errorcluster, "Controls[]"=w1608:refnum<vi>[])  [unwired: 1 in, 1 out]
            n614 = for {
              tunnel: w1593 -> [w1623] mode=indexing
              tunnel: [w1622] -> w1592 mode=indexing if=w1620
              i -> [w1621]
              n615 = case shown="\"NG\"" w1623 {
                tunnel: [2 ("CYCLE STATUS OK, NOK, ABORTED") 1 ("CYCLE STATUS OK, NOK, ABORTED") 0 ("CYCLE STATUS OK, NOK, ABORTED")] -> w1622
                frame "NG" {
                }
                frame "OK" {
                }
                frame "-1", Default {
                }
              }
              n616 = Not Equal To 0?(x=w1621) -> (x != 0?=w1620:bool)
            }
            n617 = Index Array(array=w1608, index #1=2 ("index"), index #2=4 ("index")) -> (element #1=w1595:refnum<vi>, element #2=w1590:refnum<vi>)
            n618 = Build Array(w1595, w1590) -> (w1594:refnum<vi>[])
            n619 = for {
              tunnel: w1594 -> [w1632] mode=indexing
              shift-right: [w1628] -> w1605
              shift-left: w1606 -> [w1630]
              tunnel: w1592 -> [w1627] mode=indexing
              w1631 = refnum<vi> refnum  # Boolean
              n620 = To More Specific Class(target class=w1631, reference=w1632, error in=w1630) -> (specific class reference=w1633:refnum<vi>, error out=w1629:errorcluster)
              n621 = call "PADMINI_BOOL_COLOR_CHANGE.vi"("error in (no error)"=w1629, "Numeric"=w1627, "Boolean in"=w1633) -> ("error out"=w1628:errorcluster)  [unwired: 8 in]
            }
          }
          frame "SCAN10" {
            # "STATION OP 10"
            n622 = case shown="False" w1677 {
              tunnel: w1681 -> [w1705 w1744]
              tunnel: w1680 -> [w1697 w1743]
              tunnel: w1679 -> [w1682 _]
              tunnel: [w1700 w1742] -> w1676
              tunnel: [w1698 w1744] -> w1678
              tunnel: [w1683 "" ("trimmed string")] -> w1669
              frame False {
                (unwired) "REPORT"
                n623 = call "PADMINI_AUTO_BARCODE_STRING 100.vi"("Enum"=enum16{"Read", "Write"}."Read", "error in (no error)"=w1697) -> ("error out"=w1696:errorcluster, "Input 2"=w1685:string[])  [unwired: 8 in]
                n624 = global read "Global 1.vi" "BARCODE RECIPE"() -> (w1686:string)
                n625 = Index Array(array=w1685) -> (element=w1684:string)  [unwired: 1 in]
                n626 = call <vilib>:"Trim Whitespace.vi"("string"=w1684) -> ("trimmed string"=w1683:string)  [unwired: 1 in]
                n627 = Match Pattern(string=w1683, regular expression=w1686) -> (match substring=w1687:string)  [unwired: 1 in, 3 out]
                n628 = String Length(string=w1686) -> (length=w1689:i32)
                n629 = String Length(string=w1687) -> (length=w1688:i32)
                n630 = Format Into String(format string="WHERE BARCODE  ='%s'", w1683) -> (resulting string=w1693:string)  [unwired: 2 in, 1 out]
                n631 = Equal?(x=w1689, y=w1688) -> (x = y?=w1690:bool)
                n632 = call <vilib>:"DB Tools Select Data.vi"("condition"=w1693, "error in (no error)"=w1696, "columns"=string[] ["BARCODE", "ST9_FINAL_RST", "ST10_FINAL_RST"], "table"=w1682, "connection reference"=w1705) -> ("error out"=w1703:errorcluster, "data"=w1702:variant[][], "connection reference out"=w1698:T13)  [unwired: 1 in]
                n633 = call "PADMINI_varient_to_data.vi"("error in (no error)"=w1703, "data"=w1702) -> ("error out"=w1701:errorcluster, "Array"=w1699:string[][])  [unwired: 8 in]
                n634 = Equal?(x=w1683, y="") -> (x = y?=w1691:bool)
                n635 = case shown="False" w1691 {
                  tunnel: w1701 -> [w1709 w1738]
                  tunnel: [w1708 w1737] -> w1700
                  tunnel: w1699 -> [w1707 _]
                  tunnel: w1690 -> [w1706 _]
                  frame False {
                    n636 = case shown="True" w1706 {
                      tunnel: w1709 -> [w1713 w1722]
                      tunnel: [w1712 w1721] -> w1708
                      tunnel: w1707 -> [_ w1734]
                      frame False {
                        w1710 = i32[] [0, 0, 0, 0, 0]  # I/P
                        n637 = call "PADMINI_AUTO_BARCODE_STATUS 90.vi"("Enum"=enum16{"Read", "Write"}."Write", "error in (no error)"=w1713, "I/P"=w1710) -> ("error out"=w1712:errorcluster)  [unwired: 7 in, 1 out]
                      }
                      frame True {
                        n638 = Index Array(array=w1734, index (row) #1=0 ("index (row)"), index (col) #1=1 ("disabled index (col)"), index (row) #2=0 ("index (row)"), index (col) #2=2 ("disabled index (col)")) -> (element #1=w1728:string)  [unwired: 1 out]
                        n639 = Empty String/Path?(string/path=w1728) -> (empty?=w1726:bool)
                        n640 = Equal?(x=w1728, y="OK") -> (x = y?=w1724:bool)
                        n641 = Boolean To (0,1)(Boolean=TRUE ("element")) -> (0, 1=w1719:i16)
                        n642 = Not(x=w1724) -> (.not. x?=w1723:bool)
                        n643 = Boolean To (0,1)(Boolean=FALSE ("element")) -> (0, 1=w1718:i16)
                        n644 = Boolean To (0,1)(Boolean=w1726) -> (0, 1=w1717:i16)
                        n645 = Boolean To (0,1)(Boolean=w1724) -> (0, 1=w1716:i16)
                        n646 = Boolean To (0,1)(Boolean=w1723) -> (0, 1=w1715:i16)
                        n647 = Build Array(w1719, w1718, w1717, w1716, w1715) -> (w1714:i16[])
                        n648 = call "PADMINI_AUTO_BARCODE_STATUS 100.vi"("Enum"=enum16{"Read", "Write"}."Write", "error in (no error)"=w1722, "I/P"=w1714) -> ("error out"=w1721:errorcluster)  [unwired: 7 in, 1 out]
                      }
                    }
                  }
                  frame True {
                    w1735 = i32[] [0, 0, 0, 0, 0]  # I/P
                    n649 = call "PADMINI_AUTO_BARCODE_STATUS 100.vi"("Enum"=enum16{"Read", "Write"}."Write", "error in (no error)"=w1738, "I/P"=w1735) -> ("error out"=w1737:errorcluster)  [unwired: 7 in, 1 out]
                  }
                }
              }
              frame True {
                w1739 = i32[] [0, 0, 0, 0, 0]  # I/P
                n650 = call "PADMINI_AUTO_BARCODE_STATUS 100.vi"("Enum"=enum16{"Read", "Write"}."Write", "error in (no error)"=w1743, "I/P"=w1739) -> ("error out"=w1742:errorcluster)  [unwired: 7 in, 1 out]
              }
            }
            n651 = flat-sequence {
              tunnel: [w1746] -> w1675
              tunnel: w1676 -> [w1746]
              frame #0 {
                # "UPDATE op 100 SCAN sTATUS"
                n652 = global write "DATA LOG.vi" "OP 100 Outputs"(TRUE) -> ()
              }
            }
            n653 = Bundle By Name(cluster=w1671, "OP - 100.BARCODE"=w1669) -> (w1670:T11)
          }
          frame "SCAN11" {
            # "STATION OP 110"
            n654 = case shown="True" w1753 {
              tunnel: w1757 -> [w1781 w1819]
              tunnel: w1756 -> [w1773 w1818]
              tunnel: w1755 -> [w1758 _]
              tunnel: [w1776 w1817] -> w1752
              tunnel: [w1774 w1819] -> w1754
              frame False {
                (unwired) "REPORT"
                n655 = call "PADMINI_AUTO_BARCODE_STRING 100.vi"("Enum"=enum16{"Read", "Write"}."Read", "error in (no error)"=w1773) -> ("error out"=w1772:errorcluster, "Input 2"=w1760:string[])  [unwired: 8 in]
                n656 = global read "Global 1.vi" "BARCODE RECIPE"() -> (w1761:string)
                n657 = Index Array(array=w1760) -> (element=w1759:string)  [unwired: 1 in]
                n658 = call <vilib>:"Trim Whitespace.vi"("string"=w1759) -> ("trimmed string"=w1765:string)  [unwired: 1 in]
                n659 = Match Pattern(string=w1765, regular expression=w1761) -> (match substring=w1762:string)  [unwired: 1 in, 3 out]
                n660 = String Length(string=w1761) -> (length=w1764:i32)
                n661 = String Length(string=w1762) -> (length=w1763:i32)
                n662 = Format Into String(format string="WHERE BARCODE  ='%s'", w1765) -> (resulting string=w1769:string)  [unwired: 2 in, 1 out]
                n663 = Equal?(x=w1764, y=w1763) -> (x = y?=w1766:bool)
                n664 = call <vilib>:"DB Tools Select Data.vi"("condition"=w1769, "error in (no error)"=w1772, "columns"=string[] ["BARCODE", "ST9_FINAL_RST", "ST10_FINAL_RST"], "table"=w1758, "connection reference"=w1781) -> ("error out"=w1779:errorcluster, "data"=w1778:variant[][], "connection reference out"=w1774:T13)  [unwired: 1 in]
                n665 = call "PADMINI_varient_to_data.vi"("error in (no error)"=w1779, "data"=w1778) -> ("error out"=w1777:errorcluster, "Array"=w1775:string[][])  [unwired: 8 in]
                n666 = Equal?(x=w1765, y="") -> (x = y?=w1767:bool)
                n667 = case shown="False" w1767 {
                  tunnel: w1777 -> [w1785 w1814]
                  tunnel: [w1784 w1813] -> w1776
                  tunnel: w1775 -> [w1783 _]
                  tunnel: w1766 -> [w1782 _]
                  frame False {
                    n668 = case shown="True" w1782 {
                      tunnel: w1785 -> [w1789 w1798]
                      tunnel: [w1788 w1797] -> w1784
                      tunnel: w1783 -> [_ w1810]
                      frame False {
                        w1786 = i32[] [0, 0, 0, 0, 0]  # I/P
                        n669 = call "PADMINI_AUTO_BARCODE_STATUS 90.vi"("Enum"=enum16{"Read", "Write"}."Write", "error in (no error)"=w1789, "I/P"=w1786) -> ("error out"=w1788:errorcluster)  [unwired: 7 in, 1 out]
                      }
                      frame True {
                        n670 = Index Array(array=w1810, index (row) #1=0 ("index (row)"), index (col) #1=1 ("disabled index (col)"), index (row) #2=0 ("index (row)"), index (col) #2=2 ("disabled index (col)")) -> (element #1=w1804:string)  [unwired: 1 out]
                        n671 = Empty String/Path?(string/path=w1804) -> (empty?=w1802:bool)
                        n672 = Equal?(x=w1804, y="OK") -> (x = y?=w1800:bool)
                        n673 = Boolean To (0,1)(Boolean=TRUE ("element")) -> (0, 1=w1795:i16)
                        n674 = Boolean To (0,1)(Boolean=FALSE ("element")) -> (0, 1=w1794:i16)
                        n675 = Not(x=w1800) -> (.not. x?=w1799:bool)
                        n676 = Boolean To (0,1)(Boolean=w1802) -> (0, 1=w1793:i16)
                        n677 = Boolean To (0,1)(Boolean=w1800) -> (0, 1=w1792:i16)
                        n678 = Boolean To (0,1)(Boolean=w1799) -> (0, 1=w1791:i16)
                        n679 = Build Array(w1795, w1794, w1793, w1792, w1791) -> (w1790:i16[])
                        n680 = call "PADMINI_AUTO_BARCODE_STATUS 100.vi"("Enum"=enum16{"Read", "Write"}."Write", "error in (no error)"=w1798, "I/P"=w1790) -> ("error out"=w1797:errorcluster)  [unwired: 7 in, 1 out]
                      }
                    }
                  }
                  frame True {
                    w1811 = i32[] [0, 0, 0, 0, 0]  # I/P
                    n681 = call "PADMINI_AUTO_BARCODE_STATUS 100.vi"("Enum"=enum16{"Read", "Write"}."Write", "error in (no error)"=w1814, "I/P"=w1811) -> ("error out"=w1813:errorcluster)  [unwired: 7 in, 1 out]
                  }
                }
              }
              frame True {
                w1815 = i32[] [0, 0, 0, 0, 0]  # I/P
                n682 = call "PADMINI_AUTO_BARCODE_STATUS 100.vi"("Enum"=enum16{"Read", "Write"}."Write", "error in (no error)"=w1818, "I/P"=w1815) -> ("error out"=w1817:errorcluster)  [unwired: 7 in, 1 out]
              }
            }
            n683 = flat-sequence {
              tunnel: [w1821] -> w1751
              tunnel: w1752 -> [w1821]
              frame #0 {
                # "UPDATE op 100 SCAN sTATUS"
                n684 = global write "DATA LOG.vi" "OP 100 Outputs"(TRUE) -> ()
              }
            }
          }
          frame "DATALOG10" {
            w1822 = 0.0 ("OP - 100.Response Time FWD (mSec)")
            w1857 = T14 2 items=["no dialog", "OK message", "continue or stop message", "OK message + warnings", "continue/stop + warnings"] ("type of dialog (OK msg:1)")
            # "datalog of OP 100"
            n685 = call "PADMINI_AUTO_BARCODE_STRING 100.vi"("Enum"=enum16{"Read", "Write"}."Read", "error in (no error)"=w1828) -> ("error out"=w1846:errorcluster, "Input 2"=w1839:string[])  [unwired: 8 in]
            n686 = call "PADMINI_AUTO_CYCLE TIME 100.vi"("Enum"=enum16{"Read", "Write"}."Read", "error in (no error)"=w1828) -> ("Time of Day result array"=w1827:timestamp[])  [unwired: 8 in, 1 out]
            n687 = call "PADMINI_AUTO_CYCLE VALUE 100.vi"("Enum"=enum16{"Read", "Write"}."Read", "error in (no error)"=w1828) -> ("Input 2"=w1837:dbl[])  [unwired: 8 in, 1 out]
            n688 = Index Array(array=w1837) -> (element #1=w1844:dbl, element #2=w1836:dbl, element #3=w1835:dbl, element #4=w1834:dbl, element #5=w1833:dbl, element #6=w1832:dbl, element #7=w1831:dbl, element #8=w1830:dbl)  [unwired: 8 in]
            n689 = Index Array(array=w1827) -> (element #1=w1826:timestamp, element #2=w1825:timestamp)  [unwired: 2 in]
            n690 = Number To Fractional String(number=w1837, precision (6)=i16 2) -> (F-format string=w1842:string[])  [unwired: 2 in]
            n691 = Get Date/Time String(seconds (now)=w1826) -> (time string=w1824:string)  [unwired: 2 in, 1 out]
            n692 = Get Date/Time String(seconds (now)=w1825) -> (time string=w1823:string)  [unwired: 2 in, 1 out]
            n693 = case shown="False" w1862 {
              tunnel: w1863 -> [w1901 w1928]
              tunnel: w1846 -> [w1902 w1927]
              tunnel: [w1904 w1926] -> w1860
              tunnel: [w1903 w1925] -> w1858
              tunnel: w1861 -> [w1900 _]
              tunnel: w1842 -> [w1896 w1909]
              tunnel: w1839 -> [w1893 w1910]
              tunnel: w1824 -> [w1882 w1907]
              tunnel: w1823 -> [w1881 w1908]
              frame False {
                # "DO TRACEBILITY"
                n694 = Index Array(array=w1893) -> (element=w1885:string)  [unwired: 1 in]
                n695 = call <vilib>:"Trim Whitespace.vi"("string"=w1885) -> ("trimmed string"=w1894:string)  [unwired: 1 in]
                n696 = local read "SHIFT"() -> (w1880:string)
                n697 = Index Array(array=w1896) -> (element #1=w1892:string, element #2=w1891:string, element #3=w1890:string, element #4=w1883:string, element #5=w1889:string, element #6=w1884:string, element #7=w1888:string, element #8=w1887:string, element #9=w1886:string)  [unwired: 9 in]
                n698 = call "PADMINI_SHIFT_DATE.vi"("SHIFT"=w1880) -> ("date/time string"=w1879:string)  [unwired: 10 in]
                n699 = Bundle("date/time string"=w1879, "Input 2"=w1892, "Input 2"=w1891, "Input 2"=w1890, "time string"=w1882, "time string"=w1881, "Input 2"=w1883, "Input 2"=w1889, "Input 2"=w1884, "Input 2"=w1888, "Input 2"=w1887, "Input 2"=w1886, "Input 2"=w1885) -> (w1895:T29)  [unwired: 1 in]
                n700 = Format Into String(format string="Where BARCODE='%s' ", w1894) -> (resulting string=w1898:string)  [unwired: 2 in, 1 out]
                n701 = call <vilib>:"DB Tools Update Data.vi"("condition"=w1898, "data"=w1895, "error in (no error)"=w1902, "columns"=string[] ["DATEST10", "ST10_SENSOR_OP_OPEN_V", "ST10_START_OF_CLOSE_SENSOR_V", "ST10_SENSOR_OP_FULL_CLOSE_V", "ST10_RESPONSE_TIME_FWD", "ST10_RESPONSE_TIME_REV", "ST10_MOTOR_V_START_OF_CLOSE_A", "ST10_MOTOR_V_FULL_CLOSE_B", "ST10_MOTOR_V_START_BACK_C", "ST10_MOTOR_V_FULL_OPEN_D", "ST10_MOTOR_RMS_CURRENT_A", "ST10_FINAL_RST"], "table"=w1900, "connection reference"=w1901) -> ("error out"=w1903:errorcluster, "connection reference out"=w1904:T13)  [unwired: 4 in]
              }
              frame True {
                # "TRAC BYPASS"
                n702 = local read "SHIFT"() -> (w1905:string)
                n703 = Index Array(array=w1910) -> (element=w1914:string)  [unwired: 1 in]
                n704 = call "PADMINI_SHIFT_DATE.vi"("SHIFT"=w1905) -> ("date/time string"=w1906:string)  [unwired: 10 in]
                n705 = Index Array(array=w1909) -> (element #1=w1921:string, element #2=w1920:string, element #3=w1919:string, element #4=w1912:string, element #5=w1918:string, element #6=w1913:string, element #7=w1917:string, element #8=w1916:string, element #9=w1915:string)  [unwired: 9 in]
                n706 = Bundle("date/time string"=w1906, "SHIFT"=w1905, "Input 2"=w1921, "Input 2"=w1920, "Input 2"=w1919, "time string"=w1907, "time string"=w1908, "Input 2"=w1912, "Input 2"=w1918, "Input 2"=w1913, "Input 2"=w1917, "Input 2"=w1916, "Input 2"=w1915, "Input 2"=w1914) -> (w1911:T30)  [unwired: 1 in]
                n707 = To Variant(anything=w1911) -> (Variant=w1924:variant)
                n708 = call <vilib>:"DB Tools Insert Data.vi"("data"=w1924, "error in (no error)"=w1927, "columns"=string[] ["DATE", "SHIFT", "ST10_SENSOR_OP_OPEN_V", "ST10_START_OF_CLOSE_SENSOR_V", "ST10_SENSOR_OP_FULL_CLOSE_V", "ST10_RESPONSE_TIME_FWD", "ST10_RESPONSE_TIME_REV", "ST10_MOTOR_V_START_OF_CLOSE_A", "ST10_MOTOR_V_FULL_CLOSE_B", "ST10_MOTOR_V_START_BACK_C", "ST10_MOTOR_V_FULL_OPEN_D", "ST10_MOTOR_RMS_CURRENT_A", "ST10_FINAL_RST"], "table"="ST10_REPORT", "connection reference"=w1928) -> ("error out"=w1925:errorcluster, "connection reference out"=w1926:T13)  [unwired: 5 in]
              }
            }
            n709 = Bundle By Name(cluster=w1849, "OP - 100.Sensor O/P Open V"=w1844, "OP - 100.Start Of Close Sensor V"=w1836, "OP - 100.Sensor O/P Full Close V"=w1835, "OP - 100.Response Time FWD (mSec)"=w1822, "OP - 100.Response Time REV (mSec)"=w1822, "OP - 100.Motor V Start Of Close A"=w1834, "OP - 100.Motor V Full Close B R"=w1833, "OP - 100.Motor V Start Back C"=w1832, "OP - 100.Motor V Full Open D"=w1831, "OP - 100.Motor RMS Current A"=w1830) -> (w1848:T11)
            n710 = call <vilib>:"Simple Error Handler.vi"("type of dialog (OK msg:1)"=w1857, "error in (no error)"=w1858) -> ("error out"=w1856:errorcluster)  [unwired: 3 in, 4 out]
            n711 = call <vilib>:"Clear Errors.vi"("error in (no error)"=w1856) -> ("error out"=w1854:errorcluster)  [unwired: 5 in, 1 out]
            n712 = property on="OP - 100" class="Clust"(error in=w1854) -> (error out=w1851:errorcluster, "Controls[]"=w1853:refnum<vi>[])  [unwired: 1 in, 1 out]
            n713 = for {
              tunnel: w1839 -> [w1868] mode=indexing
              tunnel: [w1867] -> w1838 mode=indexing if=w1865
              i -> [w1866]
              n714 = case shown="\"NG\"" w1868 {
                tunnel: [2 ("CYCLE STATUS OK, NOK, ABORTED") 1 ("CYCLE STATUS OK, NOK, ABORTED") 0 ("CYCLE STATUS OK, NOK, ABORTED")] -> w1867
                frame "NG" {
                }
                frame "OK" {
                }
                frame "-1", Default {
                }
              }
              n715 = Not Equal To 0?(x=w1866) -> (x != 0?=w1865:bool)
            }
            n716 = Index Array(array=w1853, index=3) -> (element=w1841:refnum<vi>)
            n717 = Build Array(w1841) -> (w1840:refnum<vi>[])
            n718 = for {
              tunnel: w1840 -> [w1877] mode=indexing
              shift-right: [w1873] -> w1850
              shift-left: w1851 -> [w1875]
              tunnel: w1838 -> [w1872] mode=indexing
              w1876 = refnum<vi> refnum  # Boolean
              n719 = To More Specific Class(target class=w1876, reference=w1877, error in=w1875) -> (specific class reference=w1878:refnum<vi>, error out=w1874:errorcluster)
              n720 = call "PADMINI_BOOL_COLOR_CHANGE.vi"("error in (no error)"=w1874, "Numeric"=w1872, "Boolean in"=w1878) -> ("error out"=w1873:errorcluster)  [unwired: 8 in]
            }
          }
          frame "EMERGENCY STOP" {
          }
          frame "STOP" {
            n721 = global read "Global 1.vi" "BARCODE RECIPE"() -> (w1939:string)
            n722 = Bundle("BARCODE RECIPE"=w1939) -> (w1938:cluster{"BARCODE RECIPE":string})  [unwired: 1 in]
            n723 = call <vilib>:"DB Tools Update Data.vi"("data"=w1938, "error in (no error)"=w1944, "columns"=string[] ["PREVIOUS_LOADED_RECIPE"], "table"="BARCODE_RECIPE", "connection reference"=w1942) -> ("error out"=w1943:errorcluster, "connection reference out"=w1941:T13)  [unwired: 5 in]
          }
        }
      }
      frame Error {
        # "Return true in any case that should stop the loop."
      }
    }
    n724 = Unbundle By Name(w123) -> ("OP - 90"=→"OP - 90":T8, "OP - 100"=→"OP - 100":T9, "OP - 110"=→"OP - 110":cluster{"BARCODE":string})
    n725 = Unbundle By Name(w123) -> ("OP - 10"=→"OP - 10":T4, "OP - 20"=→"OP - 20":T31, "OP - 30"=→"OP - 30":T3, "OP - 40"=→"OP - 40":T2)
    n726 = Unbundle By Name(w123) -> ("OP - 50"=→"OP - 50":T1, "OP - 60"=→"OP - 60":T10, "OP - 70"=→"OP - 70":T7, "OP - 80"=→"OP - 80":T6)
    n727 = Wait (ms)(milliseconds to wait=u32 100) -> ()  [unwired: 1 out]
  }
  n728 = while {
    shift-right: [w1968] -> w71
    shift-left: w20 -> [w1962]
    shift-right: [w1969] -> w65
    shift-left: w69 -> [w1977]
    stop <- w1967 stop-if-true
    n729 = local read "Shift_change"() -> (w1975:bool)
    n730 = call <vilib>:"Clear Errors.vi"("error in (no error)"=w1962) -> ("error out"=w1953:errorcluster)  [unwired: 5 in, 1 out]
    n731 = call "READ EMERGENCY BIT.vi"("Enum"=enum16{"Read", "Write"}."Read", "error in (no error)"=w1953) -> ("Array Out"=w1965:dbl[])  [unwired: 8 in, 1 out]
    n732 = case shown="True" w1975 {
      tunnel: w1953 -> [w1994 w2007]
      tunnel: [w1995 w2006] -> w1974
      frame False {
        n733 = local read "SHIFT_DATA 2"() -> (w1997:string[])
        n734 = Get Date/Time In Seconds() -> (seconds since 1Jan1904=w1996:timestamp)
        n735 = call "String To Time_4.vi"("error in (no error)"=w1994, "String Array In"=w1997) -> ("error out"=w1993:errorcluster, "Time Stamp Out"=w1992:timestamp[])  [unwired: 8 in]
        "Time Stamp Out 4" <- w1992
        n736 = call "Shift Calculation_4.vi"("error in (no error)"=w1993, "Current Time"=w1996, "Time Stamp Out"=w1992) -> ("error out"=w1991:errorcluster, "Shift"=w1990:i32)  [unwired: 7 in]
        n737 = call <vilib>:"Clear Errors.vi"("error in (no error)"=w1991) -> ()  [unwired: 5 in, 2 out]
        n738 = case shown="4" w1990 {
          tunnel: ["A" "B" "C" "D"] -> w1995
          frame 1, Default {
          }
          frame 2 {
          }
          frame 3 {
          }
          frame 4 {
          }
        }
      }
      frame True {
        n739 = local read "SHIFT_DATA"() -> (w2005:string[])
        n740 = Get Date/Time In Seconds() -> (seconds since 1Jan1904=w2008:timestamp)
        n741 = call "String To Time.vi"("error in (no error)"=w2007, "String Array In"=w2005) -> ("error out"=w2004:errorcluster, "Time Stamp Out"=w2009:timestamp[])  [unwired: 8 in]
        "Time Stamp Out" <- w2009
        n742 = call "Shift Calculation.vi"("error in (no error)"=w2004, "Current Time"=w2008, "Time Stamp Out"=w2009) -> ("error out"=w2003:errorcluster, "Shift"=w2002:i32)  [unwired: 7 in]
        "Shift 4" <- w2002
        n743 = call <vilib>:"Clear Errors.vi"("error in (no error)"=w2003) -> ()  [unwired: 5 in, 2 out]
        n744 = case shown="3" w2002 {
          tunnel: ["A" "B" "C"] -> w2006
          frame 1, Default {
          }
          frame 2 {
          }
          frame 3 {
          }
        }
      }
    }
    "SHIFT" <- w1974
    n745 = Index Array(array=w1965) -> (element=w1964:dbl)  [unwired: 1 in]
    n746 = call "VALUE_CHANGE - ST1_RESULT.vi"("Numeric"=w1964) -> ("Boolean"=w1963:bool)  [unwired: 9 in, 1 out]
    n747 = global write "Global 1.vi" "EMERGENCY STOP"(w1963) -> ()
    n748 = call "Trigger_Loggic.vi"("error in (no error)"=w1953) -> ("error out"=w1958:errorcluster, "Array"=w1978:i32[])  [unwired: 9 in]
    n749 = for {
      tunnel: w1978 -> [w2013] mode=indexing
      shift-right: [w2017] -> w1971
      shift-left: w1977 -> [w2016]
      shift-right: [w2015] -> w1970
      shift-left: w1958 -> [w2014]
      n750 = case shown="1" w2013 {
        tunnel: [w2020 w2025 w2030 w2035 w2040 w2045 w2050 w2055 w2060 w2065 w2070 w2075 w2080 w2085 w2090 w2095 w2100 w2105 w2110 w2115 w2120 w2125 w2130] -> w2017
        tunnel: w2016 -> [w2022 w2027 w2032 w2037 w2042 w2047 w2052 w2057 w2062 w2067 w2072 w2077 w2082 w2087 w2092 w2097 w2102 w2107 w2112 w2117 w2122 w2127 w2132]
        tunnel: [w2019 w2024 w2029 w2034 w2039 w2044 w2049 w2054 w2059 w2064 w2069 w2074 w2079 w2084 w2089 w2094 w2099 w2104 w2109 w2114 w2119 w2124 w2129] -> w2015
        tunnel: w2014 -> [w2021 w2026 w2031 w2036 w2041 w2046 w2051 w2056 w2061 w2066 w2071 w2076 w2081 w2086 w2091 w2096 w2101 w2106 w2111 w2116 w2121 w2126 w2131]
        frame -1, Default {
          # "DEFAULT"
          n751 = Enqueue Element(queue=w2022, element=cluster{"CASE 2":T12} {"CASE 2"=enum."-1"}, error in (no error)=w2021) -> (queue out=w2020:refnum<queue>, error out=w2019:errorcluster)  [unwired: 1 in, 1 out]
        }
        frame 0 {
          # "SCAN BARCODE OP 10"
          n752 = Enqueue Element(queue=w2027, element=cluster{"CASE 2":T12} {"CASE 2"=enum."SCAN1"}, error in (no error)=w2026) -> (queue out=w2025:refnum<queue>, error out=w2024:errorcluster)  [unwired: 1 in, 1 out]
        }
        frame 1 {
          # "DATALOG OF OP 10"
          n753 = Enqueue Element(queue=w2032, element=cluster{"CASE 2":T12} {"CASE 2"=enum."DATALOG1"}, error in (no error)=w2031) -> (queue out=w2030:refnum<queue>, error out=w2029:errorcluster)  [unwired: 1 in, 1 out]
        }
        frame 2 {
          # "SCAN BARCODE OP 20"
          n754 = Enqueue Element(queue=w2037, element=cluster{"CASE 2":T12} {"CASE 2"=enum."SCAN2"}, error in (no error)=w2036) -> (queue out=w2035:refnum<queue>, error out=w2034:errorcluster)  [unwired: 1 in, 1 out]
        }
        frame 3 {
          # "DATALOG OF OP 20"
          n755 = Enqueue Element(queue=w2042, element=cluster{"CASE 2":T12} {"CASE 2"=enum."DATALOG2"}, error in (no error)=w2041) -> (queue out=w2040:refnum<queue>, error out=w2039:errorcluster)  [unwired: 1 in, 1 out]
        }
        frame 4 {
          # "SCAN BARCODE OP 30"
          n756 = Enqueue Element(queue=w2047, element=cluster{"CASE 2":T12} {"CASE 2"=enum."SCAN3"}, error in (no error)=w2046) -> (queue out=w2045:refnum<queue>, error out=w2044:errorcluster)  [unwired: 1 in, 1 out]
        }
        frame 5 {
          # "DATALOG OF OP 30"
          n757 = Enqueue Element(queue=w2052, element=cluster{"CASE 2":T12} {"CASE 2"=enum."DATALOG3"}, error in (no error)=w2051) -> (queue out=w2050:refnum<queue>, error out=w2049:errorcluster)  [unwired: 1 in, 1 out]
        }
        frame 6 {
          # "SCAN BARCODE OP 40"
          n758 = Enqueue Element(queue=w2057, element=cluster{"CASE 2":T12} {"CASE 2"=enum."SCAN4"}, error in (no error)=w2056) -> (queue out=w2055:refnum<queue>, error out=w2054:errorcluster)  [unwired: 1 in, 1 out]
        }
        frame 7 {
          # "DATALOG OF OP 40"
          n759 = Enqueue Element(queue=w2062, element=cluster{"CASE 2":T12} {"CASE 2"=enum."DATALOG4"}, error in (no error)=w2061) -> (queue out=w2060:refnum<queue>, error out=w2059:errorcluster)  [unwired: 1 in, 1 out]
        }
        frame 8 {
          # "SCAN BARCODE OP 50"
          n760 = Enqueue Element(queue=w2067, element=cluster{"CASE":T12} {"CASE"=enum."SCAN5"}, error in (no error)=w2066) -> (queue out=w2065:refnum<queue>, error out=w2064:errorcluster)  [unwired: 1 in, 1 out]
        }
        frame 9 {
          # "DATALOG OF OP 50"
          n761 = Enqueue Element(queue=w2072, element=cluster{"CASE":T12} {"CASE"=enum."DATALOG5"}, error in (no error)=w2071) -> (queue out=w2070:refnum<queue>, error out=w2069:errorcluster)  [unwired: 1 in, 1 out]
        }
        frame 10 {
          # "SCAN BARCODE OP 60"
          n762 = Enqueue Element(queue=w2077, element=cluster{"CASE 2":T12} {"CASE 2"=enum."SCAN6"}, error in (no error)=w2076) -> (queue out=w2075:refnum<queue>, error out=w2074:errorcluster)  [unwired: 1 in, 1 out]
        }
        frame 11 {
          # "DATALOG OF OP 60"
          n763 = Enqueue Element(queue=w2082, element=cluster{"CASE 2":T12} {"CASE 2"=enum."DATALOG6"}, error in (no error)=w2081) -> (queue out=w2080:refnum<queue>, error out=w2079:errorcluster)  [unwired: 1 in, 1 out]
        }
        frame 12 {
          # "SCAN BARCODE OP 70"
          n764 = Enqueue Element(queue=w2087, element=cluster{"CASE 2":T12} {"CASE 2"=enum."SCAN7"}, error in (no error)=w2086) -> (queue out=w2085:refnum<queue>, error out=w2084:errorcluster)  [unwired: 1 in, 1 out]
        }
        frame 13 {
          # "DATALOG OF OP 70"
          n765 = Enqueue Element(queue=w2092, element=cluster{"CASE 2":T12} {"CASE 2"=enum."DATALOG7"}, error in (no error)=w2091) -> (queue out=w2090:refnum<queue>, error out=w2089:errorcluster)  [unwired: 1 in, 1 out]
        }
        frame 14 {
          # "SCAN BARCODE 80"
          n766 = Enqueue Element(queue=w2097, element=cluster{"CASE 2":T12} {"CASE 2"=enum."SCAN8"}, error in (no error)=w2096) -> (queue out=w2095:refnum<queue>, error out=w2094:errorcluster)  [unwired: 1 in, 1 out]
        }
        frame 15 {
          # "DATALOG OF OP 80"
          n767 = Enqueue Element(queue=w2102, element=cluster{"CASE 2":T12} {"CASE 2"=enum."DATALOG8"}, error in (no error)=w2101) -> (queue out=w2100:refnum<queue>, error out=w2099:errorcluster)  [unwired: 1 in, 1 out]
        }
        frame 16 {
          # "SCAN BARCODE OP 90"
          n768 = Enqueue Element(queue=w2107, element=cluster{"CASE 2":T12} {"CASE 2"=enum."SCAN9"}, error in (no error)=w2106) -> (queue out=w2105:refnum<queue>, error out=w2104:errorcluster)  [unwired: 1 in, 1 out]
        }
        frame 17 {
          # "DATALOG OF OP 90"
          n769 = Enqueue Element(queue=w2112, element=cluster{"CASE 2":T12} {"CASE 2"=enum."DATALOG9"}, error in (no error)=w2111) -> (queue out=w2110:refnum<queue>, error out=w2109:errorcluster)  [unwired: 1 in, 1 out]
        }
        frame 18 {
          # "SCAN BARCODE OP 100"
          n770 = Enqueue Element(queue=w2117, element=cluster{"CASE 2":T12} {"CASE 2"=enum."SCAN10"}, error in (no error)=w2116) -> (queue out=w2115:refnum<queue>, error out=w2114:errorcluster)  [unwired: 1 in, 1 out]
        }
        frame 19 {
          # "DATALOG OF OP 100"
          n771 = Enqueue Element(queue=w2122, element=cluster{"CASE 2":T12} {"CASE 2"=enum."DATALOG10"}, error in (no error)=w2121) -> (queue out=w2120:refnum<queue>, error out=w2119:errorcluster)  [unwired: 1 in, 1 out]
        }
        frame 20 {
          # "SCAN BARCODE OP 110"
          n772 = Enqueue Element(queue=w2127, element=cluster{"CASE 2":T12} {"CASE 2"=enum."SCAN11"}, error in (no error)=w2126) -> (queue out=w2125:refnum<queue>, error out=w2124:errorcluster)  [unwired: 1 in, 1 out]
        }
        frame 21 {
          # "DATALOG OF OP 110"
          n773 = Enqueue Element(queue=w2132, element=cluster{"CASE 2":T12} {"CASE 2"=enum."DATALOG11"}, error in (no error)=w2131) -> (queue out=w2130:refnum<queue>, error out=w2129:errorcluster)  [unwired: 1 in, 1 out]
        }
      }
    }
    n774 = Wait (ms)(milliseconds to wait=u32 50) -> ()  [unwired: 1 out]
    n775 = global read "Global 1.vi" "PLC COMM"() -> (→"PLC COM.":bool)
    n776 = global read "Global 1.vi" "PLC 1"() -> (→"OP 10 & 20":bool)
    n777 = global read "Global 1.vi" "PLC 2"() -> (→"OP 30":bool)
    n778 = global read "Global 1.vi" "PLC 3"() -> (→"OP 40":bool)
    n779 = case shown="True" "stop 2" {
      tunnel: w1971 -> [w1981 w1987]
      tunnel: [w1981 w1986] -> w1969
      tunnel: w1970 -> [w1980 w1985]
      tunnel: [w1980 w1984] -> w1968
      tunnel: [FALSE TRUE] -> w1967
      frame False {
      }
      frame True {
        n780 = Flush Queue(queue=w1987, error in (no error)=w1985) -> (queue out=w1989:refnum<queue>, error out=w1988:errorcluster)  [unwired: 1 out]
        n781 = Enqueue Element(queue=w1989, element=cluster{"CASE 2":T12} {"CASE 2"=enum."STOP"}, error in (no error)=w1988) -> (queue out=w1986:refnum<queue>, error out=w1984:errorcluster)  [unwired: 1 in, 1 out]
      }
    }
    "stop" <- w1967
    n782 = global read "Global 1.vi" "PLC 4"() -> (→"OP 50":bool)
    n783 = global read "Global 1.vi" "PLC 5"() -> (→"OP 60":bool)
    n784 = global read "Global 1.vi" "PLC 7"() -> (→"OP 90 -100 - 110":bool)
    n785 = global read "Global 1.vi" "PLC 6"() -> (→"OP 70 & 80":bool)
  }
  n786 = Release Queue(queue=w65, error in (no error)=w71) -> (error out=w48:errorcluster)  [unwired: 1 in, 2 out]
  n787 = call <vilib>:"Clear Errors.vi"("error in (no error)"=w67) -> ("error out"=w52:errorcluster)  [unwired: 5 in, 1 out]
  n788 = call <vilib>:"DB Tools Close Connection.vi"("error in (no error)"=w52, "connection reference"=w66) -> ("error out"=w49:errorcluster)  [unwired: 5 in]
  n789 = Merge Errors(w48, w49) -> (w50:errorcluster)
  n790 = call <vilib>:"Simple Error Handler.vi"("error in (no error)"=w50) -> ("error out"=w45:errorcluster)  [unwired: 4 in, 4 out]
  n791 = call <vilib>:"Clear Errors.vi"("error in (no error)"=w45) -> ("error out"=w51:errorcluster)  [unwired: 5 in, 1 out]
  n792 = flat-sequence {
    tunnel: w51 -> [w2134]
    tunnel: [w2134] -> w53
    frame #0 {
      n793 = global write "Global 1.vi" "REMOVE VI"(TRUE ("remove_VI")) -> ()
    }
  }
  n794 = property class="App"(error in=w53) -> (error out=w55:errorcluster, "App.Kind"=w54:T32)  [unwired: 1 in, 1 out]
  n795 = case shown="\"Run Time System\"" w54 {
    tunnel: [w2135 w2137] -> w56
    tunnel: w55 -> [w2135 w2136]
    frame "Development System", Default {
    }
    frame "Run Time System" {
      n796 = invoke class="VI" method="FP.Close"(error in=w2136) -> (error out=w2137:errorcluster)  [unwired: 2 in, 2 out]
    }
  }
  "error out 2" <- w56
